vi "Recipe read write.vi"(7 "Use csv file":bool=TRUE, 8 "Write":bool, 9 "Info":string, 10 "Recipe path":path, 11 "Write input":T1={"SEM Scan Parameters"={"X size (um)"=20.0, "Y size (um)"=20.0, "X center (um)"=0.0, "Y center (um)"=0.0, "X size (V)"=6.190428211586902, "X size auto"=TRUE, "X stig"=[[0.0]], "Y stig"=[[0.0]], "X aln"=[[0.0]], "Y aln"=[[0.0]], "Scan rate (Hz)"=10000000, "Oversampling"=5, "Oversampling auto"=TRUE, "Frame line rampdown ratio"=0.1, "Pixel size (nm)"=10.0, "WD (mm)"=[[3.0]], "X tiles"=1, "Y tiles"=1, "Overlap (um)"=1.0, "Interlaced"=TRUE, "dX (um)"=[0.0], "dY (um)"=[0.0], "Frames"=1}, "Detector Information"={"Brightness A"=30.0, "Contrast A"=25.0, "Detector B name"="ESB", "Brightness B"=40.0, "Contrast B"=50.0, "Detector C name"="Detector C", "Detector D name"="Detector D"}, "SEM Options"={"GetInfo"=TRUE, "Set Det A para"=TRUE, "Set WD"=FALSE, "Set Mag"=TRUE, "Set stig"=FALSE, "Set aln"=FALSE, "Display"=TRUE, "Save"=TRUE, "8-bit"=TRUE, "Detector A"=TRUE, "Detector B"=FALSE, "Detector C"=FALSE, "Detector D"=FALSE, "Inverse A"=FALSE, "Inverse B"=FALSE, "Inverse C"=FALSE, "Inverse D"=FALSE, "Inverse PNG"=TRUE, "Freeze"=TRUE, "PNG only"=FALSE, "Upload"=TRUE, "Delete after upload"=FALSE}, "Focus Index Options"={"Keep aspect ratio"=FALSE, "Show Focus Index"=TRUE, "Focus Index primary grid center"=TRUE, "X Grids"=[[0]], "Y Grids"=[[0]], "Primary X index"=[[0]], "Primary Y index"=[[0]]}, "Image fit to"=0, "File Information"={"File path"=path "E:/Images", "Notes"="", "Save recipe"=FALSE, "Load recipe"=FALSE, "Sample ID"=""}, "Low mag SEM"={"Low mag scan"=TRUE, "Prior to main scan"=FALSE, "Low mag interval"=1, "Low mag scan FOV (micron)"=200.0, "Low mag scan rate (Hz)"=1000000, "Show HM box"=TRUE}, "Mid Mag SEM"={"Mid mag scan"=FALSE, "Prior to main scan"=FALSE, "Mid mag interval"=500, "X size (um)"=6144.0, "Y size (um)"=6144.0, "X center (um)"=0.0, "Y center (um)"=0.0, "Mid mag scan rate (Hz)"=1000000, "Pixel size (nm)"=10.0, "Show MM box"=TRUE}, "FIB-SEM Angle"=90.0, "Milling para"={"X resolution"=4096, "Z resolution"=125001, "X offset (um)"=0.0, "Z offset (um)"=0.0, "X center (um)"=0.0, "Z center (um)"=0.0, "X size (um)"=250.0, "Z size (um)"=250.0, "UL-Ang"=90.0, "UR-Ang"=90.0, "Line milling time (s)"=5.0, "Z-step (nm)"=2.0, "Lines auto pause"=1, "Auto pause"=FALSE, "Mill from Bottom"=FALSE, "FIB FOV (um)"=500.0, "Auto Profile"=FALSE, "Mill start from Last"=FALSE, "FIB PID on"=FALSE, "FIB PID reset"=TRUE, "FIB PID measured"=0, "FIB PID target"=0.0, "FIB PID target slope"=0.0, "FIB PID P"=0.001, "FIB PID I"=0.01, "FIB PID D"=0.0, "Emission (uA)"=1.36, "Suppressor (V)"=50.0, "Auto reheat"=FALSE}, "FI Detector"=0, "Auto Optimzation"=TRUE, "Images per Auto Optimization"=200, "AF Range (nm)"=1800.0, "AF Steps"=7, "AS Range (%)"=0.6, "AS Steps"=7, "AA Range (%)"=3.0, "AA Steps"=7, "X shift (nm/frame)"=0.0, "Y shift (nm/frame)"=0.0, "FIB Y zoom pixel (nm)"=20.0, "Mail server"="", "Email Alert Recipients"=[""], "Alert Settings"={"3D imaging paused alarm"=TRUE, "FIB emission limit warning"=TRUE, "Low limit"=1.4, "High limit"=2.0, "Specimen @ SEM alarm"=TRUE, "FIB CL current alarm"=TRUE, "Beam Dump 1 alarm"=TRUE, "Milling Z voltage alarm"=TRUE, "EHT off alarm"=TRUE, "Detector over scale warning"=TRUE, "Image clipping alarm"=TRUE, "Warning limit (um)"=1.4, "Stop limit (um)"=1.4, "Temperature alarm"=TRUE, "Pause 3D-ING"=FALSE, "Low limit (F)"=65.0, "High limit (F)"=80.0, "Temp limit auto"=TRUE, "Delta (F)"=0.2, "Gradient limit (F/min)"=0.03, "SW error warning"=TRUE, "Focus index warning"=TRUE, "Focus index low limit"=0.1, "Focus index stop limit"=0.0, "Run Auto Stig"=FALSE, "FI low limit auto"=TRUE, "FI stop limit auto"=TRUE}, "Reheat Parameters"={"Filament I (A)"=3.0, "Reheat time (s)"=45.0, "Emission (uA)"=2.2, "Calculate V/I slope"=TRUE, "Pre-calc delay (min)"=5.0, "Disable Reheat Retries"=FALSE, "Restore Voltages"=TRUE}, "Start FIB HV DataLog"=FALSE, "Interval (s)"=60} {"Milling para"."Suppressor (V)" step=0.1 format="%.1g"; "Milling para"."Emission (uA)" step=0.1 format="%.2g"; "Milling para"."FIB PID measured" items=["Spec.", "B.D. 1", "B.D. 2", "Mill", "Spec. +"]; "Milling para"."FIB PID target slope" min=-1 max=1 step=0.1; "Milling para"."UR-Ang" format="%.2f"; "Milling para"."UL-Ang" format="%.2f"; "Milling para"."Z offset (um)" step=0.02 format="%.3g"; "Milling para"."X offset (um)" step=1 format="%.3g"; "Milling para"."FIB FOV (um)" format="%.3g"; "Milling para"."Line milling time (s)" format="%.1f"; "Milling para"."Z center (um)" format="%#.3g"; "Milling para"."X center (um)" format="%#.3g"; "Alert Settings"."Stop limit (um)" format="%.2f"; "Alert Settings"."Warning limit (um)" format="%.2f"; "Alert Settings"."Focus index stop limit" format="%_3g"; "Alert Settings"."Focus index low limit" format="%_3g"; "Alert Settings"."High limit (F)" format="%.2g"; "Alert Settings"."Low limit (F)" format="%.2g"; "Alert Settings"."High limit" format="%.2f"; "Alert Settings"."Low limit" format="%.2f"; "SEM Scan Parameters"."dY (um)" format="%.1f"; "SEM Scan Parameters"."dX (um)" format="%.1f"; "SEM Scan Parameters"."Frames" min=1 step=1; "SEM Scan Parameters"."WD (mm)" format="%.1f"; "SEM Scan Parameters"."Y aln" format="%.1f"; "SEM Scan Parameters"."X aln" format="%.1f"; "SEM Scan Parameters"."Y stig" format="%.1f"; "SEM Scan Parameters"."X stig" format="%.1f"; "SEM Scan Parameters"."Overlap (um)" min=0; "SEM Scan Parameters"."Y tiles" min=1; "SEM Scan Parameters"."X tiles" min=1; "SEM Scan Parameters"."X size (um)" format="%.2f"; "SEM Scan Parameters"."Y size (um)" format="%.2f"; "SEM Scan Parameters"."Frame line rampdown ratio" min=0 max=1 step=0.05 format="%.2g"; "SEM Scan Parameters"."X center (um)" step=1.0 format="%.2f"; "SEM Scan Parameters"."Y center (um)" step=1.0 format="%.2f"; "SEM Scan Parameters"."X size (V)" format="%_4g"; "SEM Scan Parameters"."Scan rate (Hz)" max=4000000 step=100000 format="%.2e"; "Reheat Parameters"."Pre-calc delay (min)" format="%.2f"; "Reheat Parameters"."Emission (uA)" format="%.1f"; "Reheat Parameters"."Filament I (A)" format="%.2f"; "Reheat Parameters"."Reheat time (s)" format="%.1f"; "Image fit to" items=["Width", "Height"]; "Mid Mag SEM"."X center (um)" step=1.0 format="%.4f"; "Mid Mag SEM"."Y center (um)" step=1.0 format="%.4f"; "Mid Mag SEM"."Mid mag interval" min=1 step=1; "Mid Mag SEM"."Mid mag scan rate (Hz)" max=4000000 step=100000 format="%.2e"; "FIB Y zoom pixel (nm)" format="%.1g"; "X shift (nm/frame)" step=0.1; "Y shift (nm/frame)" step=0.1; "FI Detector" items=["A", "B", "C", "D"]; "Low mag SEM"."Low mag interval" min=1 step=1; "Low mag SEM"."Low mag scan rate (Hz)" max=4000000 step=100000 format="%.2e"; "Low mag SEM"."Low mag scan FOV (micron)" step=50.0; "FIB-SEM Angle" min=0.0 max=90.0}) -> (0 "error out":errorcluster, 1 "Recipe csv array":string[](array[string]), 2 "Recipe items":string[](array[string])=["SEM X resolution", "SEM Y resolution", "SEM X center", "SEM Y center", "SEM X size (V)", "SEM X size auto", "SEM X stig", "SEM Y stig", "SEM Scan rate (Hz)", "SEM WD (mm)", "SEM pixel size (nm)", "Frame line rampdown ratio", "SEM oversampling", "SEM oversampling auto", "Brightness A", "Contrast A", "Detector B name", "Brightness B", "Contrast B", "GetInfo", "Set Det A para", "Set WD", "Set Mag", "Set stig", "Display", "Save", "Detector A", "Detector B", "Detector C", "Detector D", "Inverse A", "Inverse B", "Inverse C", "Inverse D", "Inverse PNG", "Freeze", "PNG only", "File path", "Notes", "Low mag scan", "Prior to main scan", "per # of images", "Low mag scan FOV (um)", "Low mag scan rate (Hz)", "Show high mag box", "FIB-SEM angle", "Milling X resolution", "Milling Y resolution", "Milling X offset (um)", "Milling Y offset (um)", "Milling X center (um)", "Milling Y center (um)", "Milling X size (um)", "Milling Y size (um)", "Milling line milling time (s)", "Milling auto pause", "Milling lines auto pause", "Mill from bottom", "FIB FOV (um)", "SEM on during milling"], 3 "Read output":T1={"SEM Scan Parameters"={"X size (um)"=20.0, "Y size (um)"=20.0, "X center (um)"=0.0, "Y center (um)"=0.0, "X size (V)"=6.190428211586902, "X size auto"=TRUE, "X stig"=[[0.0]], "Y stig"=[[0.0]], "X aln"=[[0.0]], "Y aln"=[[0.0]], "Scan rate (Hz)"=10000000, "Oversampling"=5, "Oversampling auto"=TRUE, "Frame line rampdown ratio"=0.1, "Pixel size (nm)"=10.0, "WD (mm)"=[[3.0]], "X tiles"=1, "Y tiles"=1, "Overlap (um)"=1.0, "Interlaced"=TRUE, "dX (um)"=[0.0], "dY (um)"=[0.0], "Frames"=1}, "Detector Information"={"Brightness A"=30.0, "Contrast A"=25.0, "Detector B name"="ESB", "Brightness B"=40.0, "Contrast B"=50.0, "Detector C name"="Detector C", "Detector D name"="Detector D"}, "SEM Options"={"GetInfo"=TRUE, "Set Det A para"=TRUE, "Set WD"=FALSE, "Set Mag"=TRUE, "Set stig"=FALSE, "Set aln"=FALSE, "Display"=TRUE, "Save"=TRUE, "8-bit"=TRUE, "Detector A"=TRUE, "Detector B"=FALSE, "Detector C"=FALSE, "Detector D"=FALSE, "Inverse A"=FALSE, "Inverse B"=FALSE, "Inverse C"=FALSE, "Inverse D"=FALSE, "Inverse PNG"=TRUE, "Freeze"=TRUE, "PNG only"=FALSE, "Upload"=TRUE, "Delete after upload"=FALSE}, "Focus Index Options"={"Keep aspect ratio"=FALSE, "Show Focus Index"=TRUE, "Focus Index primary grid center"=TRUE, "X Grids"=[[0]], "Y Grids"=[[0]], "Primary X index"=[[0]], "Primary Y index"=[[0]]}, "Image fit to"=0, "File Information"={"File path"=path "E:/Images", "Notes"="", "Save recipe"=FALSE, "Load recipe"=FALSE, "Sample ID"=""}, "Low mag SEM"={"Low mag scan"=TRUE, "Prior to main scan"=FALSE, "Low mag interval"=1, "Low mag scan FOV (micron)"=200.0, "Low mag scan rate (Hz)"=1000000, "Show HM box"=TRUE}, "Mid Mag SEM"={"Mid mag scan"=FALSE, "Prior to main scan"=FALSE, "Mid mag interval"=500, "X size (um)"=6144.0, "Y size (um)"=6144.0, "X center (um)"=0.0, "Y center (um)"=0.0, "Mid mag scan rate (Hz)"=1000000, "Pixel size (nm)"=10.0, "Show MM box"=TRUE}, "FIB-SEM Angle"=90.0, "Milling para"={"X resolution"=4096, "Z resolution"=125001, "X offset (um)"=0.0, "Z offset (um)"=0.0, "X center (um)"=0.0, "Z center (um)"=0.0, "X size (um)"=250.0, "Z size (um)"=250.0, "UL-Ang"=90.0, "UR-Ang"=90.0, "Line milling time (s)"=5.0, "Z-step (nm)"=2.0, "Lines auto pause"=1, "Auto pause"=FALSE, "Mill from Bottom"=FALSE, "FIB FOV (um)"=500.0, "Auto Profile"=FALSE, "Mill start from Last"=FALSE, "FIB PID on"=FALSE, "FIB PID reset"=TRUE, "FIB PID measured"=0, "FIB PID target"=0.0, "FIB PID target slope"=0.0, "FIB PID P"=0.001, "FIB PID I"=0.01, "FIB PID D"=0.0, "Emission (uA)"=1.36, "Suppressor (V)"=50.0, "Auto reheat"=FALSE}, "FI Detector"=0, "Auto Optimzation"=TRUE, "Images per Auto Optimization"=200, "AF Range (nm)"=1800.0, "AF Steps"=7, "AS Range (%)"=0.6, "AS Steps"=7, "AA Range (%)"=3.0, "AA Steps"=7, "X shift (nm/frame)"=0.0, "Y shift (nm/frame)"=0.0, "FIB Y zoom pixel (nm)"=20.0, "Mail server"="", "Email Alert Recipients"=[""], "Alert Settings"={"3D imaging paused alarm"=TRUE, "FIB emission limit warning"=TRUE, "Low limit"=1.4, "High limit"=2.0, "Specimen @ SEM alarm"=TRUE, "FIB CL current alarm"=TRUE, "Beam Dump 1 alarm"=TRUE, "Milling Z voltage alarm"=TRUE, "EHT off alarm"=TRUE, "Detector over scale warning"=TRUE, "Image clipping alarm"=TRUE, "Warning limit (um)"=1.4, "Stop limit (um)"=1.4, "Temperature alarm"=TRUE, "Pause 3D-ING"=FALSE, "Low limit (F)"=65.0, "High limit (F)"=80.0, "Temp limit auto"=TRUE, "Delta (F)"=0.2, "Gradient limit (F/min)"=0.03, "SW error warning"=TRUE, "Focus index warning"=TRUE, "Focus index low limit"=0.1, "Focus index stop limit"=0.0, "Run Auto Stig"=FALSE, "FI low limit auto"=TRUE, "FI stop limit auto"=TRUE}, "Reheat Parameters"={"Filament I (A)"=3.0, "Reheat time (s)"=45.0, "Emission (uA)"=2.2, "Calculate V/I slope"=TRUE, "Pre-calc delay (min)"=5.0, "Disable Reheat Retries"=FALSE, "Restore Voltages"=TRUE}, "Start FIB HV DataLog"=FALSE, "Interval (s)"=60} {"Milling para"."Suppressor (V)" step=0.1 format="%.1g"; "Milling para"."Emission (uA)" step=0.1 format="%.2g"; "Milling para"."FIB PID measured" items=["Spec.", "B.D. 1", "B.D. 2", "Mill", "Spec. +"]; "Milling para"."FIB PID target slope" min=-1 max=1 step=0.1; "Milling para"."UR-Ang" format="%.2f"; "Milling para"."UL-Ang" format="%.2f"; "Milling para"."Z offset (um)" step=0.02 format="%.3g"; "Milling para"."X offset (um)" step=1 format="%.3g"; "Milling para"."FIB FOV (um)" format="%.3g"; "Milling para"."Line milling time (s)" format="%.1f"; "Milling para"."Z center (um)" format="%#.3g"; "Milling para"."X center (um)" format="%#.3g"; "Alert Settings"."Stop limit (um)" format="%.2f"; "Alert Settings"."Warning limit (um)" format="%.2f"; "Alert Settings"."Focus index stop limit" format="%_3g"; "Alert Settings"."Focus index low limit" format="%_3g"; "Alert Settings"."High limit (F)" format="%.2g"; "Alert Settings"."Low limit (F)" format="%.2g"; "Alert Settings"."High limit" format="%.2f"; "Alert Settings"."Low limit" format="%.2f"; "SEM Scan Parameters"."dY (um)" format="%.1f"; "SEM Scan Parameters"."dX (um)" format="%.1f"; "SEM Scan Parameters"."Frames" min=1 step=1; "SEM Scan Parameters"."WD (mm)" format="%.1f"; "SEM Scan Parameters"."Y aln" format="%.1f"; "SEM Scan Parameters"."X aln" format="%.1f"; "SEM Scan Parameters"."Y stig" format="%.1f"; "SEM Scan Parameters"."X stig" format="%.1f"; "SEM Scan Parameters"."Overlap (um)" min=0; "SEM Scan Parameters"."Y tiles" min=1; "SEM Scan Parameters"."X tiles" min=1; "SEM Scan Parameters"."X size (um)" format="%.2f"; "SEM Scan Parameters"."Y size (um)" format="%.2f"; "SEM Scan Parameters"."Frame line rampdown ratio" min=0 max=1 step=0.05 format="%.2g"; "SEM Scan Parameters"."X center (um)" step=1.0 format="%.2f"; "SEM Scan Parameters"."Y center (um)" step=1.0 format="%.2f"; "SEM Scan Parameters"."X size (V)" format="%_4g"; "SEM Scan Parameters"."Scan rate (Hz)" max=4000000 step=100000 format="%.2e"; "Reheat Parameters"."Pre-calc delay (min)" format="%.2f"; "Reheat Parameters"."Emission (uA)" format="%.1f"; "Reheat Parameters"."Filament I (A)" format="%.2f"; "Reheat Parameters"."Reheat time (s)" format="%.1f"; "Image fit to" items=["Width", "Height"]; "Mid Mag SEM"."X center (um)" step=1.0 format="%.4f"; "Mid Mag SEM"."Y center (um)" step=1.0 format="%.4f"; "Mid Mag SEM"."Mid mag interval" min=1 step=1; "Mid Mag SEM"."Mid mag scan rate (Hz)" max=4000000 step=100000 format="%.2e"; "FIB Y zoom pixel (nm)" format="%.1g"; "X shift (nm/frame)" step=0.1; "Y shift (nm/frame)" step=0.1; "FI Detector" items=["A", "B", "C", "D"]; "Low mag SEM"."Low mag interval" min=1 step=1; "Low mag SEM"."Low mag scan rate (Hz)" max=4000000 step=100000 format="%.2e"; "Low mag SEM"."Low mag scan FOV (micron)" step=50.0; "FIB-SEM Angle" min=0.0 max=90.0})   [LabVIEW 2018]
uses:
  <vilib>/Utility/file.llb/Read From Spreadsheet File (string).vi
  <vilib>/regexp/Match Regular Expression.xnode
panel:
  out "Read output 1":T2={"SEM Scan Parameters"={"X size (um)"=20.0, "Y size (um)"=20.0, "X center (um)"=0.0, "Y center (um)"=0.0, "X size (V)"=6.190428211586902, "X size auto"=TRUE, "X stig"=[[0.0]], "Y stig"=[[0.0]], "X aln"=[[0.0]], "Y aln"=[[0.0]], "Scan rate (Hz)"=10000000, "Oversampling"=5, "Oversampling auto"=TRUE, "Frame line rampdown ratio"=0.1, "Pixel size (nm)"=10.0, "WD (mm)"=[[3.0]], "X tiles"=1, "Y tiles"=1, "Overlap (um)"=1.0, "Interlaced"=TRUE, "dX (um)"=[0.0], "dY (um)"=[0.0], "Frames"=1}, "Detector Information"={"Brightness A"=30.0, "Contrast A"=25.0, "Detector B name"="ESB", "Brightness B"=40.0, "Contrast B"=50.0, "Detector C name"="Detector C", "Detector D name"="Detector D"}, "SEM Options"={"GetInfo"=TRUE, "Set Det A para"=TRUE, "Set WD"=FALSE, "Set Mag"=TRUE, "Set stig"=FALSE, "Set aln"=FALSE, "Display"=TRUE, "Save"=TRUE, "8-bit"=TRUE, "Detector A"=TRUE, "Detector B"=FALSE, "Detector C"=FALSE, "Detector D"=FALSE, "Inverse A"=FALSE, "Inverse B"=FALSE, "Inverse C"=FALSE, "Inverse D"=FALSE, "Inverse PNG"=TRUE, "Freeze"=TRUE, "PNG only"=FALSE, "Upload"=TRUE, "Delete after upload"=FALSE}, "Focus Index Options"={"Keep aspect ratio"=FALSE, "Show Focus Index"=TRUE, "Focus Index primary grid center"=TRUE, "X Grids"=[[0]], "Y Grids"=[[0]], "Primary X index"=[[0]], "Primary Y index"=[[0]]}, "Image fit to"=0, "File Information"={"File path"=path "E:/Images", "Notes"="", "Save recipe"=FALSE, "Load recipe"=FALSE, "Sample ID"=""}, "Low mag SEM"={"Low mag scan"=TRUE, "Prior to main scan"=FALSE, "Low mag interval"=1, "Low mag scan FOV (micron)"=200.0, "Low mag scan rate (Hz)"=1000000, "Show HM box"=TRUE}, "Mid Mag SEM"={"Mid mag scan"=FALSE, "Prior to main scan"=FALSE, "Mid mag interval"=500, "X size (um)"=6144.0, "Y size (um)"=6144.0, "X center (um)"=0.0, "Y center (um)"=0.0, "Mid mag scan rate (Hz)"=1000000, "Pixel size (nm)"=10.0, "Show MM box"=TRUE}, "FIB-SEM Angle"=90.0, "Milling para"={"X resolution"=4096, "Y resolution"=100001, "X offset (um)"=0.0, "Y offset (um)"=0.0, "X center (um)"=0.0, "Y center (um)"=0.0, "X size (um)"=250.0, "Y size (um)"=250.0, "UL-Ang"=90.0, "UR-Ang"=90.0, "Line milling time (s)"=5.0, "Auto pause"=FALSE, "Lines auto pause"=1, "Mill from Bottom"=FALSE, "FIB FOV (um)"=500.0, "Auto Profile"=FALSE, "Mill start from Last"=FALSE, "FIB PID on"=FALSE, "FIB PID reset"=FALSE, "FIB PID measured"=0, "FIB PID target"=0.0, "FIB PID target slope"=0.0, "FIB PID P"=0.0, "FIB PID I"=0.0, "FIB PID D"=0.0}, "FI Detector"=0, "Auto Optimzation"=TRUE, "Images per Auto Optimization"=200, "AF Range (nm)"=1800.0, "AF Steps"=7, "AS Range (%)"=0.6, "AS Steps"=7, "AA Range (%)"=3.0, "AA Steps"=7, "X shift (nm/frame)"=0.0, "Y shift (nm/frame)"=0.0, "FIB Settings"={"Z-step (nm)"=2.5, "Enable alarm"=TRUE, "Label"="Emission Alarm (nA)", "Emission min"=1.2, "Emission max"=2.2, "Auto reheat"=FALSE}, "FIB Y zoom pixel (nm)"=20.0, "Mail server"="", "Email Alert Recipients"=[""], "Alert Settings"={"3D imaging paused alarm"=TRUE, "FIB emission limit warning"=TRUE, "Low limit"=1.4, "High limit"=2.0, "Specimen @ SEM alarm"=TRUE, "FIB CL current alarm"=TRUE, "Beam Dump 1 alarm"=TRUE, "Milling Y voltage alarm"=TRUE, "EHT off alarm"=TRUE, "Detector over scale warning"=TRUE, "Image clipping alarm"=TRUE, "Warning limit (um)"=1.4, "Stop limit (um)"=1.4, "Temperature alarm"=TRUE, "Pause 3D-ING"=FALSE, "Low limit (F)"=65.0, "High limit (F)"=80.0, "Temp limit auto"=TRUE, "Delta (F)"=0.2, "Gradient limit (F/min)"=0.03, "SW error warning"=TRUE, "Focus index warning"=TRUE, "Focus index low limit"=0.1, "Focus index stop limit"=0.0, "Run Auto Stig"=FALSE, "FI low limit auto"=TRUE, "FI stop limit auto"=TRUE}, "Reheat Parameters"={"Filament I (A)"=3.0, "Reheat time (s)"=45.0, "Emission (uA)"=2.2, "Calculate V/I slope"=TRUE, "Pre-calc delay (min)"=5.0, "Disable Reheat Retries"=FALSE, "Restore Voltages"=TRUE}, "Start FIB HV DataLog"=FALSE, "Interval (s)"=60} {"Alert Settings"."Stop limit (um)" format="%.2f"; "Alert Settings"."Warning limit (um)" format="%.2f"; "Alert Settings"."Focus index stop limit" format="%_3g"; "Alert Settings"."Focus index low limit" format="%_3g"; "Alert Settings"."High limit (F)" format="%.2g"; "Alert Settings"."Low limit (F)" format="%.2g"; "Alert Settings"."High limit" format="%.2f"; "Alert Settings"."Low limit" format="%.2f"; "SEM Scan Parameters"."dY (um)" format="%.1f"; "SEM Scan Parameters"."dX (um)" format="%.1f"; "SEM Scan Parameters"."Frames" min=1 step=1; "SEM Scan Parameters"."WD (mm)" format="%.1f"; "SEM Scan Parameters"."Y aln" format="%.1f"; "SEM Scan Parameters"."X aln" format="%.1f"; "SEM Scan Parameters"."Y stig" format="%.1f"; "SEM Scan Parameters"."X stig" format="%.1f"; "SEM Scan Parameters"."Overlap (um)" min=0; "SEM Scan Parameters"."Y tiles" min=1; "SEM Scan Parameters"."X tiles" min=1; "SEM Scan Parameters"."X size (um)" format="%.2f"; "SEM Scan Parameters"."Y size (um)" format="%.2f"; "SEM Scan Parameters"."Frame line rampdown ratio" min=0 max=1 step=0.05 format="%.2g"; "SEM Scan Parameters"."X center (um)" step=1.0 format="%.2f"; "SEM Scan Parameters"."Y center (um)" step=1.0 format="%.2f"; "SEM Scan Parameters"."X size (V)" format="%_4g"; "SEM Scan Parameters"."Scan rate (Hz)" max=4000000 step=100000 format="%.2e"; "Reheat Parameters"."Pre-calc delay (min)" format="%.2f"; "Reheat Parameters"."Emission (uA)" format="%.1f"; "Reheat Parameters"."Filament I (A)" format="%.2f"; "Reheat Parameters"."Reheat time (s)" format="%.1f"; "Image fit to" items=["Width", "Height"]; "Mid Mag SEM"."X center (um)" step=1.0 format="%.4f"; "Mid Mag SEM"."Y center (um)" step=1.0 format="%.4f"; "Mid Mag SEM"."Mid mag interval" min=1 step=1; "Mid Mag SEM"."Mid mag scan rate (Hz)" max=4000000 step=100000 format="%.2e"; "Milling para"."FIB PID measured" items=["Spec.", "B.D.1", "B.D.2", "Mill"]; "Milling para"."UR-Ang" format="%.2f"; "Milling para"."UL-Ang" format="%.2f"; "Milling para"."Y offset (um)" step=0.02 format="%.3g"; "Milling para"."X offset (um)" step=1 format="%.3g"; "Milling para"."FIB FOV (um)" format="%.3g"; "Milling para"."Line milling time (s)" format="%.1f"; "Milling para"."Y center (um)" format="%#.3g"; "Milling para"."X center (um)" format="%#.3g"; "FIB Y zoom pixel (nm)" format="%.1g"; "FIB Settings"."Emission min" format="%.1g"; "FIB Settings"."Emission max" format="%.1g"; "X shift (nm/frame)" step=0.1; "Y shift (nm/frame)" step=0.1; "FI Detector" items=["A", "B", "C", "D"]; "Low mag SEM"."Low mag interval" min=1 step=1; "Low mag SEM"."Low mag scan rate (Hz)" max=4000000 step=100000 format="%.2e"; "Low mag SEM"."Low mag scan FOV (micron)" step=50.0; "FIB-SEM Angle" min=0.0 max=90.0}
  out "Read output 3":T3={"SEM Scan Parameters"={"X size (um)"=20.0, "Y size (um)"=20.0, "X center (um)"=0.0, "Y center (um)"=0.0, "X size (V)"=6.190428211586902, "X size auto"=TRUE, "X stig"=[[0.0]], "Y stig"=[[0.0]], "X aln"=[[0.0]], "Y aln"=[[0.0]], "Scan rate (Hz)"=10000000, "Oversampling"=5, "Oversampling auto"=TRUE, "Frame line rampdown ratio"=0.1, "Pixel size (nm)"=10.0, "WD (mm)"=[[3.0]], "X tiles"=1, "Y tiles"=1, "Overlap (um)"=1.0, "Interlaced"=TRUE, "dX (um)"=[0.0], "dY (um)"=[0.0], "Frames"=1}, "Detector Information"={"Brightness A"=30.0, "Contrast A"=25.0, "Detector B name"="ESB", "Brightness B"=40.0, "Contrast B"=50.0, "Detector C name"="Detector C", "Detector D name"="Detector D"}, "SEM Options"={"GetInfo"=TRUE, "Set Det A para"=TRUE, "Set WD"=FALSE, "Set Mag"=TRUE, "Set stig"=FALSE, "Set aln"=FALSE, "Display"=TRUE, "Save"=TRUE, "8-bit"=TRUE, "Detector A"=TRUE, "Detector B"=FALSE, "Detector C"=FALSE, "Detector D"=FALSE, "Inverse A"=FALSE, "Inverse B"=FALSE, "Inverse C"=FALSE, "Inverse D"=FALSE, "Inverse PNG"=TRUE, "Freeze"=TRUE, "PNG only"=FALSE, "Upload"=TRUE, "Delete after upload"=FALSE}, "Keep aspect ratio"=TRUE, "Show Focus Index"=TRUE, "Focus Index primary grid center"=TRUE, "Focus Index grid X"=1, "Focus Index grid Y"=1, "Focus Index primary X grid"=0, "Focus Index primary Y grid"=0, "Image fit to"=0, "File Information"={"File path"=path "E:/Images", "Notes"="", "Save recipe"=FALSE, "Load recipe"=FALSE, "Sample ID"=""}, "Low mag SEM"={"Low mag scan"=TRUE, "Prior to main scan"=FALSE, "Low mag interval"=1, "Low mag scan FOV (micron)"=200.0, "Low mag scan rate (Hz)"=1000000, "Show HM box"=TRUE}, "Mid Mag SEM"={"Mid mag scan"=FALSE, "Prior to main scan"=FALSE, "Mid mag interval"=500, "X size (um)"=6144.0, "Y size (um)"=6144.0, "X center (um)"=0.0, "Y center (um)"=0.0, "Mid mag scan rate (Hz)"=1000000, "Pixel size (nm)"=10.0, "Show MM box"=TRUE}, "FIB-SEM Angle"=90.0, "Milling para"={"X resolution"=4096, "Y resolution"=100001, "X offset (um)"=0.0, "Y offset (um)"=0.0, "X center (um)"=0.0, "Y center (um)"=0.0, "X size (um)"=250.0, "Y size (um)"=250.0, "UL-Ang"=90.0, "UR-Ang"=90.0, "Line milling time (s)"=5.0, "Auto pause"=FALSE, "Lines auto pause"=1, "Mill from Bottom"=FALSE, "FIB FOV (um)"=500.0, "Auto Profile"=FALSE, "Mill start from Last"=FALSE, "FIB PID on"=FALSE, "FIB PID reset"=FALSE, "FIB PID measured"=0, "FIB PID target"=0.0, "FIB PID target slope"=0.0, "FIB PID P"=0.0, "FIB PID I"=0.0, "FIB PID D"=0.0}, "FI Detector"=0, "Auto Optimzation"=TRUE, "Images per Auto Optimization"=200, "AF Range (nm)"=1800.0, "AF Steps"=7, "AS Range (%)"=0.6, "AS Steps"=7, "AA Range (%)"=3.0, "AA Steps"=7, "X shift (nm/frame)"=0.0, "Y shift (nm/frame)"=0.0, "FIB Settings"={"Z-step (nm)"=2.5, "Enable alarm"=TRUE, "Label"="Emission Alarm (nA)", "Emission min"=1.2, "Emission max"=2.2, "Auto reheat"=FALSE}, "FIB Y zoom pixel (nm)"=20.0, "Mail server"="", "Email Alert Recipients"=[""], "Alert Settings"={"3D imaging paused alarm"=TRUE, "FIB emission limit warning"=TRUE, "Low limit"=17.0, "High limit"=23.0, "Specimen current alarm "=TRUE, "Beam dump alarm"=TRUE, "EHT off alarm"=TRUE, "Temperature alarm"=TRUE, "Pause 3D-ING"=FALSE, "Low limit (F)"=70.0, "High limit (F)"=80.0, "Temp limit auto"=TRUE, "Delta (F)"=0.2, "Gradient limit (F/min)"=0.03, "SW error warning"=TRUE, "Focus index warning"=TRUE, "Focus index low limit"=0.1, "Focus index stop limit"=0.0, "Run Auto Stig"=FALSE, "FI low limit auto"=TRUE, "FI stop limit auto"=TRUE}, "Reheat Parameters"={"Filament I (A)"=3.0, "Reheat time (s)"=45.0, "Emission (uA)"=2.2, "Calculate V/I slope"=TRUE, "Pre-calc delay (min)"=5.0, "Disable Reheat Retries"=FALSE, "Restore Voltages"=TRUE}, "Start FIB HV DataLog"=FALSE, "Interval (s)"=60} {"SEM Scan Parameters"."dY (um)" format="%.1f"; "SEM Scan Parameters"."dX (um)" format="%.1f"; "SEM Scan Parameters"."Frames" min=1 step=1; "SEM Scan Parameters"."WD (mm)" format="%.1f"; "SEM Scan Parameters"."Y aln" format="%.1f"; "SEM Scan Parameters"."X aln" format="%.1f"; "SEM Scan Parameters"."Y stig" format="%.1f"; "SEM Scan Parameters"."X stig" format="%.1f"; "SEM Scan Parameters"."Overlap (um)" min=0; "SEM Scan Parameters"."Y tiles" min=1; "SEM Scan Parameters"."X tiles" min=1; "SEM Scan Parameters"."X size (um)" format="%.2f"; "SEM Scan Parameters"."Y size (um)" format="%.2f"; "SEM Scan Parameters"."Frame line rampdown ratio" min=0 max=1 step=0.05 format="%.2g"; "SEM Scan Parameters"."X center (um)" step=1.0 format="%.2f"; "SEM Scan Parameters"."Y center (um)" step=1.0 format="%.2f"; "SEM Scan Parameters"."X size (V)" format="%_4g"; "SEM Scan Parameters"."Scan rate (Hz)" max=4000000 step=100000 format="%.2e"; "Reheat Parameters"."Pre-calc delay (min)" format="%.2f"; "Reheat Parameters"."Emission (uA)" format="%.1f"; "Reheat Parameters"."Filament I (A)" format="%.2f"; "Reheat Parameters"."Reheat time (s)" format="%.1f"; "Image fit to" items=["Width", "Height"]; "Mid Mag SEM"."X center (um)" step=1.0 format="%.4f"; "Mid Mag SEM"."Y center (um)" step=1.0 format="%.4f"; "Mid Mag SEM"."Mid mag interval" min=1 step=1; "Mid Mag SEM"."Mid mag scan rate (Hz)" max=4000000 step=100000 format="%.2e"; "Alert Settings"."Focus index stop limit" format="%_3g"; "Milling para"."FIB PID measured" items=["Spec.", "B.D.1", "B.D.2", "Mill"]; "Milling para"."UR-Ang" format="%.2f"; "Milling para"."UL-Ang" format="%.2f"; "Milling para"."Y offset (um)" step=0.02 format="%.3g"; "Milling para"."X offset (um)" step=1 format="%.3g"; "Milling para"."FIB FOV (um)" format="%.3g"; "Milling para"."Line milling time (s)" format="%.1f"; "Milling para"."Y center (um)" format="%#.3g"; "Milling para"."X center (um)" format="%#.3g"; "Focus Index grid X" min=1; "Focus Index grid Y" min=1; "FIB Y zoom pixel (nm)" format="%.1g"; "FIB Settings"."Emission min" format="%.1g"; "FIB Settings"."Emission max" format="%.1g"; "X shift (nm/frame)" step=0.1; "Y shift (nm/frame)" step=0.1; "FI Detector" items=["A", "B", "C", "D"]; "Low mag SEM"."Low mag interval" min=1 step=1; "Low mag SEM"."Low mag scan rate (Hz)" max=4000000 step=100000 format="%.2e"; "Low mag SEM"."Low mag scan FOV (micron)" step=50.0; "FIB-SEM Angle" min=0.0 max=90.0}
  out "Read output 4":T4={"SEM Scan Parameters"={"X size (um)"=20.0, "Y size (um)"=20.0, "X center (um)"=0.0, "Y center (um)"=0.0, "X size (V)"=6.190428211586902, "X size auto"=TRUE, "X stig"=[[0.0]], "Y stig"=[[0.0]], "X aln"=[[0.0]], "Y aln"=[[0.0]], "Scan rate (Hz)"=10000000, "Oversampling"=5, "Oversampling auto"=TRUE, "Frame line rampdown ratio"=0.1, "Pixel size (nm)"=10.0, "WD (mm)"=[[3.0]], "X tiles"=1, "Y tiles"=1, "Overlap (um)"=1.0, "Interlaced"=TRUE, "dX (um)"=0.0, "dY (um)"=0.0, "Frames"=1}, "Detector Information"={"Brightness A"=30.0, "Contrast A"=25.0, "Detector B name"="ESB", "Brightness B"=40.0, "Contrast B"=50.0, "Detector C name"="Detector C", "Detector D name"="Detector D"}, "SEM Options"={"GetInfo"=TRUE, "Set Det A para"=TRUE, "Set WD"=FALSE, "Set Mag"=TRUE, "Set stig"=FALSE, "Set aln"=FALSE, "Display"=TRUE, "Save"=TRUE, "8-bit"=TRUE, "Detector A"=TRUE, "Detector B"=FALSE, "Detector C"=FALSE, "Detector D"=FALSE, "Inverse A"=FALSE, "Inverse B"=FALSE, "Inverse C"=FALSE, "Inverse D"=FALSE, "Inverse PNG"=TRUE, "Freeze"=TRUE, "PNG only"=FALSE, "Upload"=TRUE, "Delete after upload"=FALSE}, "Keep aspect ratio"=TRUE, "Show Focus Index"=TRUE, "Focus Index primary grid center"=TRUE, "Focus Index grid X"=1, "Focus Index grid Y"=1, "Focus Index primary X grid"=0, "Focus Index primary Y grid"=0, "Image fit to"=0, "File Information"={"File path"=path "E:/Images", "Notes"="", "Save recipe"=FALSE, "Load recipe"=FALSE, "Sample ID"=""}, "Low mag SEM"={"Low mag scan"=TRUE, "Prior to main scan"=FALSE, "Low mag interval"=1, "Low mag scan FOV (micron)"=200.0, "Low mag scan rate (Hz)"=1000000, "Show HM box"=TRUE}, "Mid Mag SEM"={"Mid mag scan"=FALSE, "Prior to main scan"=FALSE, "Mid mag interval"=500, "X size (um)"=6144.0, "Y size (um)"=6144.0, "X center (um)"=0.0, "Y center (um)"=0.0, "Mid mag scan rate (Hz)"=1000000, "Pixel size (nm)"=10.0, "Show MM box"=TRUE}, "FIB-SEM Angle"=90.0, "Milling para"={"X resolution"=4096, "Y resolution"=100001, "X offset (um)"=0.0, "Y offset (um)"=0.0, "X center (um)"=0.0, "Y center (um)"=0.0, "X size (um)"=250.0, "Y size (um)"=250.0, "UL-Ang"=90.0, "UR-Ang"=90.0, "Line milling time (s)"=5.0, "Auto pause"=FALSE, "Lines auto pause"=1, "Mill from Bottom"=FALSE, "FIB FOV (um)"=500.0, "SEM on"=FALSE, "Mill start from Last"=FALSE, "FIB PID on"=FALSE, "FIB PID reset"=FALSE, "FIB PID measured"=0, "FIB PID target"=0.0, "FIB PID target slope"=0.0, "FIB PID P"=0.0, "FIB PID I"=0.0, "FIB PID D"=0.0}, "FI Detector"=0, "Auto Optimzation"=TRUE, "Images per Auto Optimization"=200, "AF Range (nm)"=1800.0, "AF Steps"=7, "AS Range (%)"=0.6, "AS Steps"=7, "AA Range (%)"=3.0, "AA Steps"=7, "X shift (nm/frame)"=0.0, "Y shift (nm/frame)"=0.0, "FIB Settings"={"Z-step (nm)"=2.5, "Enable alarm"=TRUE, "Label"="Emission Alarm (nA)", "Emission min"=1.2, "Emission max"=2.2, "Auto reheat"=FALSE}, "FIB Y zoom pixel (nm)"=20.0, "Mail server"="", "Email Alert Recipients"=[""], "Alert Settings"={"3D imaging paused alarm"=TRUE, "FIB emission limit warning"=TRUE, "Low limit"=17.0, "High limit"=23.0, "Specimen current alarm "=TRUE, "Beam dump alarm"=TRUE, "EHT off alarm"=TRUE, "Temperature alarm"=TRUE, "Pause 3D-ING"=FALSE, "Low limit (F)"=70.0, "High limit (F)"=80.0, "Temp limit auto"=TRUE, "Delta (F)"=0.2, "Gradient limit (F/min)"=0.03, "SW error warning"=TRUE, "Focus index warning"=TRUE, "Focus index low limit"=0.1, "Focus index stop limit"=0.0, "Run Auto Stig"=FALSE, "FI low limit auto"=TRUE, "FI stop limit auto"=TRUE}, "Reheat Parameters"={"Filament I (A)"=3.0, "Reheat time (s)"=45.0, "Emission (uA)"=2.2, "Calculate V/I slope"=TRUE, "Pre-calc delay (min)"=5.0, "Disable Reheat Retries"=FALSE, "Restore Voltages"=TRUE}, "Start FIB HV DataLog"=FALSE, "Interval (s)"=60} {"SEM Scan Parameters"."Frames" min=1 step=1; "SEM Scan Parameters"."dX (um)" step=1 format="%.2f"; "SEM Scan Parameters"."dY (um)" step=1 format="%.2f"; "SEM Scan Parameters"."WD (mm)" format="%.1f"; "SEM Scan Parameters"."Y aln" format="%.1f"; "SEM Scan Parameters"."X aln" format="%.1f"; "SEM Scan Parameters"."Y stig" format="%.1f"; "SEM Scan Parameters"."X stig" format="%.1f"; "SEM Scan Parameters"."Overlap (um)" min=0; "SEM Scan Parameters"."Y tiles" min=1; "SEM Scan Parameters"."X tiles" min=1; "SEM Scan Parameters"."X size (um)" format="%.2f"; "SEM Scan Parameters"."Y size (um)" format="%.2f"; "SEM Scan Parameters"."Frame line rampdown ratio" min=0 max=1 step=0.05 format="%.2g"; "SEM Scan Parameters"."X center (um)" step=1.0 format="%.2f"; "SEM Scan Parameters"."Y center (um)" step=1.0 format="%.2f"; "SEM Scan Parameters"."X size (V)" format="%_4g"; "SEM Scan Parameters"."Scan rate (Hz)" max=4000000 step=100000 format="%.2e"; "Reheat Parameters"."Pre-calc delay (min)" format="%.2f"; "Reheat Parameters"."Emission (uA)" format="%.1f"; "Reheat Parameters"."Filament I (A)" format="%.2f"; "Reheat Parameters"."Reheat time (s)" format="%.1f"; "Image fit to" items=["Width", "Height"]; "Mid Mag SEM"."X center (um)" step=1.0 format="%.4f"; "Mid Mag SEM"."Y center (um)" step=1.0 format="%.4f"; "Mid Mag SEM"."Mid mag interval" min=1 step=1; "Mid Mag SEM"."Mid mag scan rate (Hz)" max=4000000 step=100000 format="%.2e"; "Alert Settings"."Focus index stop limit" format="%_3g"; "Milling para"."FIB PID measured" items=["Spec.", "B.D.1", "B.D.2", "Mill"]; "Milling para"."UR-Ang" format="%.2f"; "Milling para"."UL-Ang" format="%.2f"; "Milling para"."Y offset (um)" step=0.02 format="%.3g"; "Milling para"."X offset (um)" step=1 format="%.3g"; "Milling para"."FIB FOV (um)" format="%.3g"; "Milling para"."Line milling time (s)" format="%.1f"; "Milling para"."Y center (um)" format="%#.3g"; "Milling para"."X center (um)" format="%#.3g"; "Focus Index grid X" min=1; "Focus Index grid Y" min=1; "FIB Y zoom pixel (nm)" format="%.1g"; "FIB Settings"."Emission min" format="%.1g"; "FIB Settings"."Emission max" format="%.1g"; "X shift (nm/frame)" step=0.1; "Y shift (nm/frame)" step=0.1; "FI Detector" items=["A", "B", "C", "D"]; "Low mag SEM"."Low mag interval" min=1 step=1; "Low mag SEM"."Low mag scan rate (Hz)" max=4000000 step=100000 format="%.2e"; "Low mag SEM"."Low mag scan FOV (micron)" step=50.0; "FIB-SEM Angle" min=0.0 max=90.0}
  out "Read output 2":T5={"SEM Scan Parameters"={"X size (um)"=20.0, "Y size (um)"=20.0, "X center (um)"=0.0, "Y center (um)"=0.0, "X size (V)"=6.190428211586902, "X size auto"=TRUE, "X stig"=[[0.0]], "Y stig"=[[0.0]], "X aln"=[[0.0]], "Y aln"=[[0.0]], "Scan rate (Hz)"=10000000, "Oversampling"=5, "Oversampling auto"=TRUE, "Frame line rampdown ratio"=0.1, "Pixel size (nm)"=10.0, "WD (mm)"=[[3.0]], "X tiles"=1, "Y tiles"=1, "Overlap (um)"=1.0, "Interlaced"=TRUE, "dX (um)"=[0.0], "dY (um)"=[0.0], "Frames"=1}, "Detector Information"={"Brightness A"=30.0, "Contrast A"=25.0, "Detector B name"="ESB", "Brightness B"=40.0, "Contrast B"=50.0, "Detector C name"="Detector C", "Detector D name"="Detector D"}, "SEM Options"={"GetInfo"=TRUE, "Set Det A para"=TRUE, "Set WD"=FALSE, "Set Mag"=TRUE, "Set stig"=FALSE, "Set aln"=FALSE, "Display"=TRUE, "Save"=TRUE, "8-bit"=TRUE, "Detector A"=TRUE, "Detector B"=FALSE, "Detector C"=FALSE, "Detector D"=FALSE, "Inverse A"=FALSE, "Inverse B"=FALSE, "Inverse C"=FALSE, "Inverse D"=FALSE, "Inverse PNG"=TRUE, "Freeze"=TRUE, "PNG only"=FALSE, "Upload"=TRUE, "Delete after upload"=FALSE}, "Keep aspect ratio"=TRUE, "Show Focus Index"=TRUE, "Focus Index primary grid center"=TRUE, "Focus Index grid X"=1, "Focus Index grid Y"=1, "Focus Index primary X grid"=0, "Focus Index primary Y grid"=0, "Image fit to"=0, "File Information"={"File path"=path "E:/Images", "Notes"="", "Save recipe"=FALSE, "Load recipe"=FALSE, "Sample ID"=""}, "Low mag SEM"={"Low mag scan"=TRUE, "Prior to main scan"=FALSE, "Low mag interval"=1, "Low mag scan FOV (micron)"=200.0, "Low mag scan rate (Hz)"=1000000, "Show HM box"=TRUE}, "Mid Mag SEM"={"Mid mag scan"=FALSE, "Prior to main scan"=FALSE, "Mid mag interval"=500, "X size (um)"=6144.0, "Y size (um)"=6144.0, "X center (um)"=0.0, "Y center (um)"=0.0, "Mid mag scan rate (Hz)"=1000000, "Pixel size (nm)"=10.0, "Show MM box"=TRUE}, "FIB-SEM Angle"=90.0, "Milling para"={"X resolution"=4096, "Y resolution"=100001, "X offset (um)"=0.0, "Y offset (um)"=0.0, "X center (um)"=0.0, "Y center (um)"=0.0, "X size (um)"=250.0, "Y size (um)"=250.0, "UL-Ang"=90.0, "UR-Ang"=90.0, "Line milling time (s)"=5.0, "Auto pause"=FALSE, "Lines auto pause"=1, "Mill from Bottom"=FALSE, "FIB FOV (um)"=500.0, "Auto Profile"=FALSE, "Mill start from Last"=FALSE, "FIB PID on"=FALSE, "FIB PID reset"=FALSE, "FIB PID measured"=0, "FIB PID target"=0.0, "FIB PID target slope"=0.0, "FIB PID P"=0.0, "FIB PID I"=0.0, "FIB PID D"=0.0}, "FI Detector"=0, "Auto Optimzation"=TRUE, "Images per Auto Optimization"=200, "AF Range (nm)"=1800.0, "AF Steps"=7, "AS Range (%)"=0.6, "AS Steps"=7, "AA Range (%)"=3.0, "AA Steps"=7, "X shift (nm/frame)"=0.0, "Y shift (nm/frame)"=0.0, "FIB Settings"={"Z-step (nm)"=2.5, "Enable alarm"=TRUE, "Label"="Emission Alarm (nA)", "Emission min"=1.2, "Emission max"=2.2, "Auto reheat"=FALSE}, "FIB Y zoom pixel (nm)"=20.0, "Mail server"="", "Email Alert Recipients"=[""], "Alert Settings"={"3D imaging paused alarm"=TRUE, "FIB emission limit warning"=TRUE, "Low limit"=1.4, "High limit"=2.0, "Specimen @ SEM alarm"=TRUE, "FIB CL current alarm"=TRUE, "Beam Dump 1 alarm"=TRUE, "Milling Y voltage alarm"=TRUE, "EHT off alarm"=TRUE, "Temperature alarm"=TRUE, "Pause 3D-ING"=FALSE, "Low limit (F)"=65.0, "High limit (F)"=80.0, "Temp limit auto"=TRUE, "Delta (F)"=0.2, "Gradient limit (F/min)"=0.03, "SW error warning"=TRUE, "Focus index warning"=TRUE, "Focus index low limit"=0.1, "Focus index stop limit"=0.0, "Run Auto Stig"=FALSE, "FI low limit auto"=TRUE, "FI stop limit auto"=TRUE}, "Reheat Parameters"={"Filament I (A)"=3.0, "Reheat time (s)"=45.0, "Emission (uA)"=2.2, "Calculate V/I slope"=TRUE, "Pre-calc delay (min)"=5.0, "Disable Reheat Retries"=FALSE, "Restore Voltages"=TRUE}, "Start FIB HV DataLog"=FALSE, "Interval (s)"=60} {"Alert Settings"."Focus index stop limit" format="%_3g"; "Alert Settings"."Focus index low limit" format="%_3g"; "Alert Settings"."High limit (F)" format="%.2g"; "Alert Settings"."Low limit (F)" format="%.2g"; "SEM Scan Parameters"."dY (um)" format="%.1f"; "SEM Scan Parameters"."dX (um)" format="%.1f"; "SEM Scan Parameters"."Frames" min=1 step=1; "SEM Scan Parameters"."WD (mm)" format="%.1f"; "SEM Scan Parameters"."Y aln" format="%.1f"; "SEM Scan Parameters"."X aln" format="%.1f"; "SEM Scan Parameters"."Y stig" format="%.1f"; "SEM Scan Parameters"."X stig" format="%.1f"; "SEM Scan Parameters"."Overlap (um)" min=0; "SEM Scan Parameters"."Y tiles" min=1; "SEM Scan Parameters"."X tiles" min=1; "SEM Scan Parameters"."X size (um)" format="%.2f"; "SEM Scan Parameters"."Y size (um)" format="%.2f"; "SEM Scan Parameters"."Frame line rampdown ratio" min=0 max=1 step=0.05 format="%.2g"; "SEM Scan Parameters"."X center (um)" step=1.0 format="%.2f"; "SEM Scan Parameters"."Y center (um)" step=1.0 format="%.2f"; "SEM Scan Parameters"."X size (V)" format="%_4g"; "SEM Scan Parameters"."Scan rate (Hz)" max=4000000 step=100000 format="%.2e"; "Reheat Parameters"."Pre-calc delay (min)" format="%.2f"; "Reheat Parameters"."Emission (uA)" format="%.1f"; "Reheat Parameters"."Filament I (A)" format="%.2f"; "Reheat Parameters"."Reheat time (s)" format="%.1f"; "Image fit to" items=["Width", "Height"]; "Mid Mag SEM"."X center (um)" step=1.0 format="%.4f"; "Mid Mag SEM"."Y center (um)" step=1.0 format="%.4f"; "Mid Mag SEM"."Mid mag interval" min=1 step=1; "Mid Mag SEM"."Mid mag scan rate (Hz)" max=4000000 step=100000 format="%.2e"; "Milling para"."FIB PID measured" items=["Spec.", "B.D.1", "B.D.2", "Mill"]; "Milling para"."UR-Ang" format="%.2f"; "Milling para"."UL-Ang" format="%.2f"; "Milling para"."Y offset (um)" step=0.02 format="%.3g"; "Milling para"."X offset (um)" step=1 format="%.3g"; "Milling para"."FIB FOV (um)" format="%.3g"; "Milling para"."Line milling time (s)" format="%.1f"; "Milling para"."Y center (um)" format="%#.3g"; "Milling para"."X center (um)" format="%#.3g"; "Focus Index grid X" min=1; "Focus Index grid Y" min=1; "FIB Y zoom pixel (nm)" format="%.1g"; "FIB Settings"."Emission min" format="%.1g"; "FIB Settings"."Emission max" format="%.1g"; "X shift (nm/frame)" step=0.1; "Y shift (nm/frame)" step=0.1; "FI Detector" items=["A", "B", "C", "D"]; "Low mag SEM"."Low mag interval" min=1 step=1; "Low mag SEM"."Low mag scan rate (Hz)" max=4000000 step=100000 format="%.2e"; "Low mag SEM"."Low mag scan FOV (micron)" step=50.0; "FIB-SEM Angle" min=0.0 max=90.0}
  # "Images"
  # "nm"
  # "%"
  # "%"
  # "Direction"
  # "Start\nfrom"
  # "<"
  # "Grids"
  # "Primary"
  # "Det"
  # "Recipe"
  # "Brightness & Contrast (%)"
  # "Detector A"
  # "Brightness & Contrast (%)"
  # "Images"
  # "nm"
  # "%"
  # "%"
  # "Grids"
  # "Primary"
  # "Direction"
  # "Start\nfrom"
  # "Det"
  # "Recipe"
  # "Brightness & Contrast (%)"
  # "Detector A"
  # "Brightness & Contrast (%)"
  # "Images"
  # "nm"
  # "%"
  # "%"
  # "Direction"
  # "Start\nfrom"
  # "Det"
  # "Recipe"
  # "Brightness & Contrast (%)"
  # "Detector A"
  # "Brightness & Contrast (%)"
  # "Images"
  # "nm"
  # "%"
  # "%"
  # "Direction"
  # "Start\nfrom"
  # "Det"
  # "Recipe"
  # "Brightness & Contrast (%)"
  # "Detector A"
  # "Brightness & Contrast (%)"
  # "Images"
  # "nm"
  # "%"
  # "%"
  # "Direction"
  # "Start\nfrom"
  # "Det"
  # "Recipe"
  # "Brightness & Contrast (%)"
  # "Detector A"
  # "Brightness & Contrast (%)"
  # "Images"
  # "nm"
  # "%"
  # "%"
  # "Direction"
  # "Start\nfrom"
  # "<"
  # "Grids"
  # "Primary"
  # "Det"
  # "Recipe"
  # "Brightness & Contrast (%)"
  # "Detector A"
  # "Brightness & Contrast (%)"
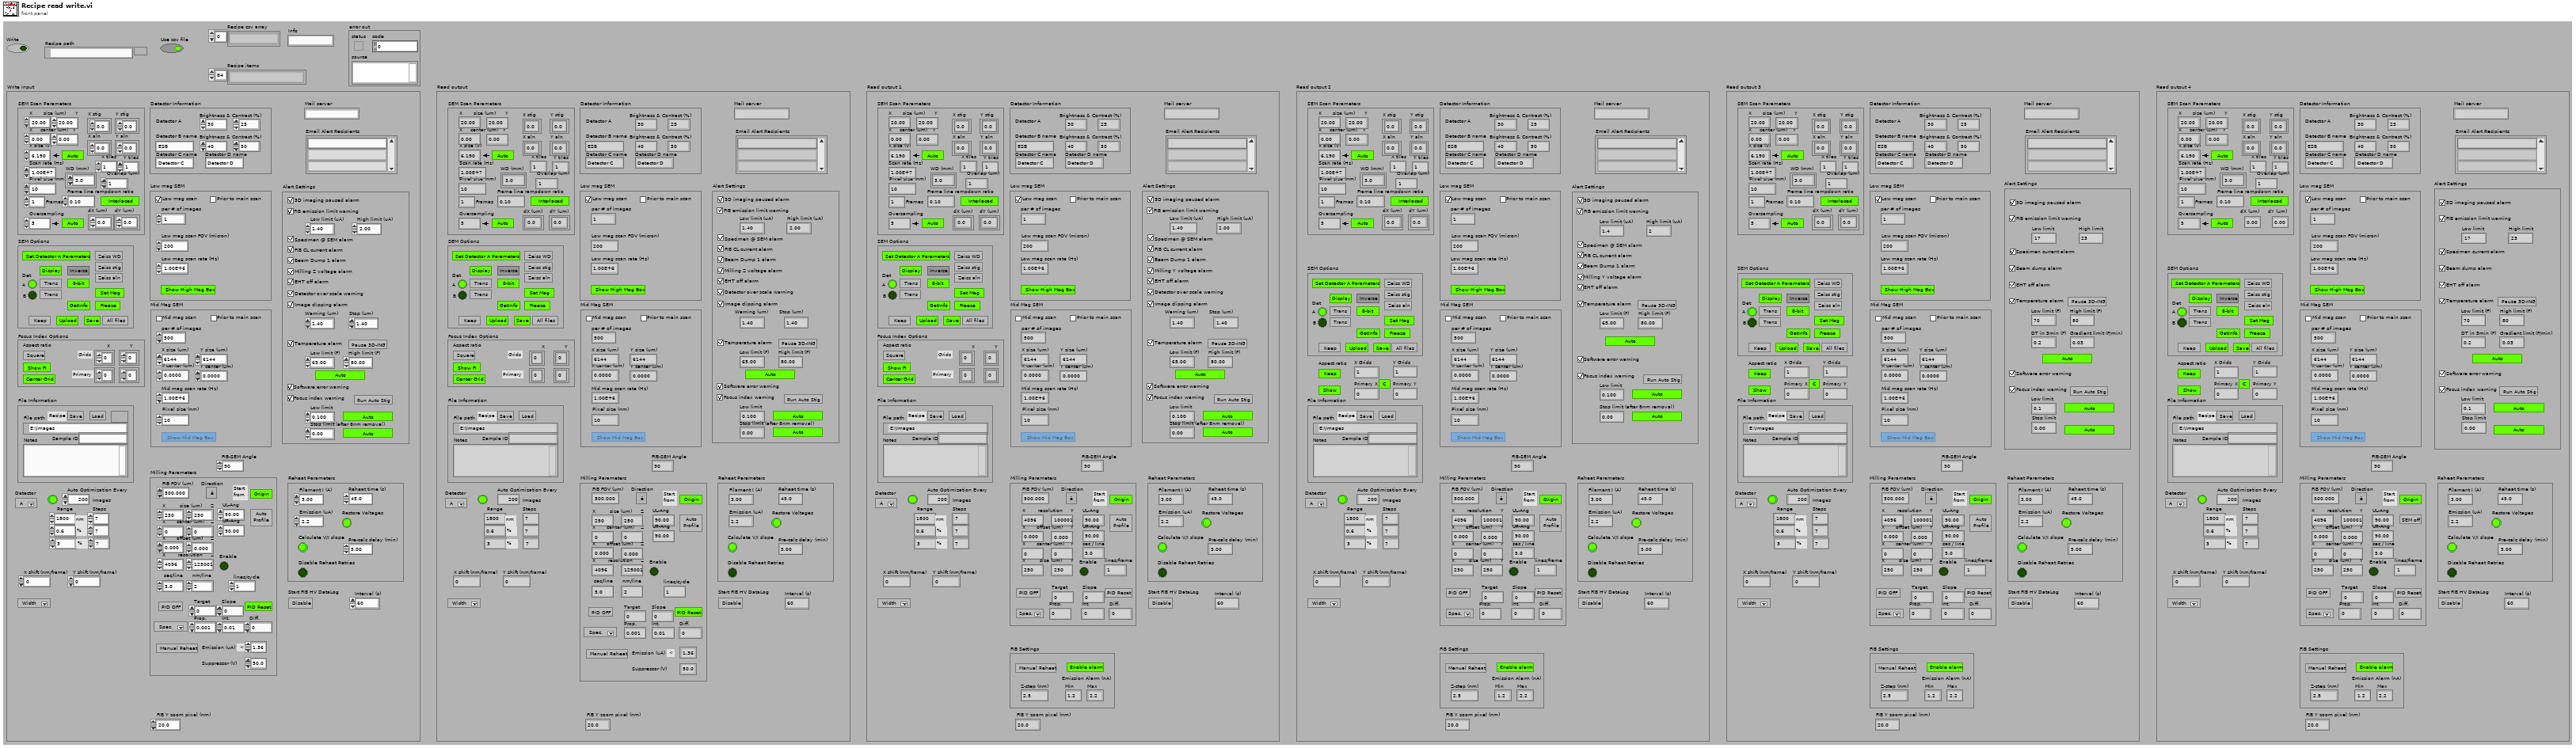
[diagram p1: front panel]
types:
  T1 = cluster{"SEM Scan Parameters":cluster{"X size (um)":sgl, "Y size (um)":sgl, "X center (um)":dbl, "Y center (um)":dbl, "X size (V)":dbl, "X size auto":bool, "X stig":sgl[][], "Y stig":sgl[][], "X aln":sgl[][], "Y aln":sgl[][], "Scan rate (Hz)":u32, "Oversampling":u32, "Oversampling auto":bool, "Frame line rampdown ratio":sgl, "Pixel size (nm)":sgl, "WD (mm)":sgl[][], "X tiles":u8, "Y tiles":u8, "Overlap (um)":sgl, "Interlaced":bool, "dX (um)":sgl[], "dY (um)":sgl[], "Frames":u8}, "Detector Information":cluster{"Brightness A":dbl, "Contrast A":dbl, "Detector B name":string, "Brightness B":dbl, "Contrast B":dbl, "Detector C name":string, "Detector D name":string}, "SEM Options":cluster{"GetInfo":bool, "Set Det A para":bool, "Set WD":bool, "Set Mag":bool, "Set stig":bool, "Set aln":bool, "Display":bool, "Save":bool, "8-bit":bool, "Detector A":bool, "Detector B":bool, "Detector C":bool, "Detector D":bool, "Inverse A":bool, "Inverse B":bool, "Inverse C":bool, "Inverse D":bool, "Inverse PNG":bool, "Freeze":bool, "PNG only":bool, "Upload":bool, "Delete after upload":bool}, "Focus Index Options":cluster{"Keep aspect ratio":bool, "Show Focus Index":bool, "Focus Index primary grid center":bool, "X Grids":u8[][], "Y Grids":u8[][], "Primary X index":u8[][], "Primary Y index":u8[][]}, "Image fit to":u8, "File Information":cluster{"File path":path, "Notes":string, "Save recipe":bool, "Load recipe":bool, "Sample ID":string}, "Low mag SEM":cluster{"Low mag scan":bool, "Prior to main scan":bool, "Low mag interval":u32, "Low mag scan FOV (micron)":dbl, "Low mag scan rate (Hz)":u32, "Show HM box":bool}, "Mid Mag SEM":cluster{"Mid mag scan":bool, "Prior to main scan":bool, "Mid mag interval":u32, "X size (um)":sgl, "Y size (um)":sgl, "X center (um)":dbl, "Y center (um)":dbl, "Mid mag scan rate (Hz)":u32, "Pixel size (nm)":dbl, "Show MM box":bool}, "FIB-SEM Angle":dbl, "Milling para":cluster{"X resolution":u32, "Z resolution":u32, "X offset (um)":sgl, "Z offset (um)":sgl, "X center (um)":sgl, "Z center (um)":sgl, "X size (um)":sgl, "Z size (um)":sgl, "UL-Ang":sgl, "UR-Ang":sgl, "Line milling time (s)":sgl, "Z-step (nm)":dbl, "Lines auto pause":u16, "Auto pause":bool, "Mill from Bottom":bool, "FIB FOV (um)":sgl, "Auto Profile":bool, "Mill start from Last":bool, "FIB PID on":bool, "FIB PID reset":bool, "FIB PID measured":u8, "FIB PID target":sgl, "FIB PID target slope":sgl, "FIB PID P":sgl, "FIB PID I":sgl, "FIB PID D":sgl, "Emission (uA)":dbl, "Suppressor (V)":sgl, "Auto reheat":bool}, "FI Detector":u16, "Auto Optimzation":bool, "Images per Auto Optimization":u16, "AF Range (nm)":sgl, "AF Steps":u8, "AS Range (%)":sgl, "AS Steps":u8, "AA Range (%)":sgl, "AA Steps":u8, "X shift (nm/frame)":dbl, "Y shift (nm/frame)":dbl, "FIB Y zoom pixel (nm)":dbl, "Mail server":string, "Email Alert Recipients":string[], "Alert Settings":cluster{"3D imaging paused alarm":bool, "FIB emission limit warning":bool, "Low limit":sgl, "High limit":sgl, "Specimen @ SEM alarm":bool, "FIB CL current alarm":bool, "Beam Dump 1 alarm":bool, "Milling Z voltage alarm":bool, "EHT off alarm":bool, "Detector over scale warning":bool, "Image clipping alarm":bool, "Warning limit (um)":sgl, "Stop limit (um)":sgl, "Temperature alarm":bool, "Pause 3D-ING":bool, "Low limit (F)":sgl, "High limit (F)":sgl, "Temp limit auto":bool, "Delta (F)":sgl, "Gradient limit (F/min)":sgl, "SW error warning":bool, "Focus index warning":bool, "Focus index low limit":sgl, "Focus index stop limit":sgl, "Run Auto Stig":bool, "FI low limit auto":bool, "FI stop limit auto":bool}, "Reheat Parameters":cluster{"Filament I (A)":sgl, "Reheat time (s)":sgl, "Emission (uA)":sgl, "Calculate V/I slope":bool, "Pre-calc delay (min)":sgl, "Disable Reheat Retries":bool, "Restore Voltages":bool}, "Start FIB HV DataLog":bool, "Interval (s)":u16}
  T2 = cluster{"SEM Scan Parameters":cluster{"X size (um)":sgl, "Y size (um)":sgl, "X center (um)":dbl, "Y center (um)":dbl, "X size (V)":dbl, "X size auto":bool, "X stig":sgl[][], "Y stig":sgl[][], "X aln":sgl[][], "Y aln":sgl[][], "Scan rate (Hz)":u32, "Oversampling":u32, "Oversampling auto":bool, "Frame line rampdown ratio":sgl, "Pixel size (nm)":sgl, "WD (mm)":sgl[][], "X tiles":u8, "Y tiles":u8, "Overlap (um)":sgl, "Interlaced":bool, "dX (um)":sgl[], "dY (um)":sgl[], "Frames":u8}, "Detector Information":cluster{"Brightness A":dbl, "Contrast A":dbl, "Detector B name":string, "Brightness B":dbl, "Contrast B":dbl, "Detector C name":string, "Detector D name":string}, "SEM Options":cluster{"GetInfo":bool, "Set Det A para":bool, "Set WD":bool, "Set Mag":bool, "Set stig":bool, "Set aln":bool, "Display":bool, "Save":bool, "8-bit":bool, "Detector A":bool, "Detector B":bool, "Detector C":bool, "Detector D":bool, "Inverse A":bool, "Inverse B":bool, "Inverse C":bool, "Inverse D":bool, "Inverse PNG":bool, "Freeze":bool, "PNG only":bool, "Upload":bool, "Delete after upload":bool}, "Focus Index Options":cluster{"Keep aspect ratio":bool, "Show Focus Index":bool, "Focus Index primary grid center":bool, "X Grids":u8[][], "Y Grids":u8[][], "Primary X index":u8[][], "Primary Y index":u8[][]}, "Image fit to":u8, "File Information":cluster{"File path":path, "Notes":string, "Save recipe":bool, "Load recipe":bool, "Sample ID":string}, "Low mag SEM":cluster{"Low mag scan":bool, "Prior to main scan":bool, "Low mag interval":u32, "Low mag scan FOV (micron)":dbl, "Low mag scan rate (Hz)":u32, "Show HM box":bool}, "Mid Mag SEM":cluster{"Mid mag scan":bool, "Prior to main scan":bool, "Mid mag interval":u32, "X size (um)":sgl, "Y size (um)":sgl, "X center (um)":dbl, "Y center (um)":dbl, "Mid mag scan rate (Hz)":u32, "Pixel size (nm)":dbl, "Show MM box":bool}, "FIB-SEM Angle":dbl, "Milling para":cluster{"X resolution":u32, "Y resolution":u32, "X offset (um)":sgl, "Y offset (um)":sgl, "X center (um)":sgl, "Y center (um)":sgl, "X size (um)":sgl, "Y size (um)":sgl, "UL-Ang":sgl, "UR-Ang":sgl, "Line milling time (s)":sgl, "Auto pause":bool, "Lines auto pause":u16, "Mill from Bottom":bool, "FIB FOV (um)":sgl, "Auto Profile":bool, "Mill start from Last":bool, "FIB PID on":bool, "FIB PID reset":bool, "FIB PID measured":u8, "FIB PID target":sgl, "FIB PID target slope":sgl, "FIB PID P":sgl, "FIB PID I":sgl, "FIB PID D":sgl}, "FI Detector":u16, "Auto Optimzation":bool, "Images per Auto Optimization":u16, "AF Range (nm)":sgl, "AF Steps":u8, "AS Range (%)":sgl, "AS Steps":u8, "AA Range (%)":sgl, "AA Steps":u8, "X shift (nm/frame)":dbl, "Y shift (nm/frame)":dbl, "FIB Settings":cluster{"Z-step (nm)":dbl, "Enable alarm":bool, "Label":string, "Emission min":dbl, "Emission max":dbl, "Auto reheat":bool}, "FIB Y zoom pixel (nm)":dbl, "Mail server":string, "Email Alert Recipients":string[], "Alert Settings":cluster{"3D imaging paused alarm":bool, "FIB emission limit warning":bool, "Low limit":sgl, "High limit":sgl, "Specimen @ SEM alarm":bool, "FIB CL current alarm":bool, "Beam Dump 1 alarm":bool, "Milling Y voltage alarm":bool, "EHT off alarm":bool, "Detector over scale warning":bool, "Image clipping alarm":bool, "Warning limit (um)":sgl, "Stop limit (um)":sgl, "Temperature alarm":bool, "Pause 3D-ING":bool, "Low limit (F)":sgl, "High limit (F)":sgl, "Temp limit auto":bool, "Delta (F)":sgl, "Gradient limit (F/min)":sgl, "SW error warning":bool, "Focus index warning":bool, "Focus index low limit":sgl, "Focus index stop limit":sgl, "Run Auto Stig":bool, "FI low limit auto":bool, "FI stop limit auto":bool}, "Reheat Parameters":cluster{"Filament I (A)":sgl, "Reheat time (s)":sgl, "Emission (uA)":sgl, "Calculate V/I slope":bool, "Pre-calc delay (min)":sgl, "Disable Reheat Retries":bool, "Restore Voltages":bool}, "Start FIB HV DataLog":bool, "Interval (s)":u16}
  T3 = cluster{"SEM Scan Parameters":cluster{"X size (um)":sgl, "Y size (um)":sgl, "X center (um)":dbl, "Y center (um)":dbl, "X size (V)":dbl, "X size auto":bool, "X stig":sgl[][], "Y stig":sgl[][], "X aln":sgl[][], "Y aln":sgl[][], "Scan rate (Hz)":u32, "Oversampling":u32, "Oversampling auto":bool, "Frame line rampdown ratio":sgl, "Pixel size (nm)":sgl, "WD (mm)":sgl[][], "X tiles":u8, "Y tiles":u8, "Overlap (um)":sgl, "Interlaced":bool, "dX (um)":sgl[], "dY (um)":sgl[], "Frames":u8}, "Detector Information":cluster{"Brightness A":dbl, "Contrast A":dbl, "Detector B name":string, "Brightness B":dbl, "Contrast B":dbl, "Detector C name":string, "Detector D name":string}, "SEM Options":cluster{"GetInfo":bool, "Set Det A para":bool, "Set WD":bool, "Set Mag":bool, "Set stig":bool, "Set aln":bool, "Display":bool, "Save":bool, "8-bit":bool, "Detector A":bool, "Detector B":bool, "Detector C":bool, "Detector D":bool, "Inverse A":bool, "Inverse B":bool, "Inverse C":bool, "Inverse D":bool, "Inverse PNG":bool, "Freeze":bool, "PNG only":bool, "Upload":bool, "Delete after upload":bool}, "Keep aspect ratio":bool, "Show Focus Index":bool, "Focus Index primary grid center":bool, "Focus Index grid X":u8, "Focus Index grid Y":u8, "Focus Index primary X grid":u8, "Focus Index primary Y grid":u8, "Image fit to":u8, "File Information":cluster{"File path":path, "Notes":string, "Save recipe":bool, "Load recipe":bool, "Sample ID":string}, "Low mag SEM":cluster{"Low mag scan":bool, "Prior to main scan":bool, "Low mag interval":u32, "Low mag scan FOV (micron)":dbl, "Low mag scan rate (Hz)":u32, "Show HM box":bool}, "Mid Mag SEM":cluster{"Mid mag scan":bool, "Prior to main scan":bool, "Mid mag interval":u32, "X size (um)":sgl, "Y size (um)":sgl, "X center (um)":dbl, "Y center (um)":dbl, "Mid mag scan rate (Hz)":u32, "Pixel size (nm)":dbl, "Show MM box":bool}, "FIB-SEM Angle":dbl, "Milling para":cluster{"X resolution":u32, "Y resolution":u32, "X offset (um)":sgl, "Y offset (um)":sgl, "X center (um)":sgl, "Y center (um)":sgl, "X size (um)":sgl, "Y size (um)":sgl, "UL-Ang":sgl, "UR-Ang":sgl, "Line milling time (s)":sgl, "Auto pause":bool, "Lines auto pause":u16, "Mill from Bottom":bool, "FIB FOV (um)":sgl, "Auto Profile":bool, "Mill start from Last":bool, "FIB PID on":bool, "FIB PID reset":bool, "FIB PID measured":u8, "FIB PID target":sgl, "FIB PID target slope":sgl, "FIB PID P":sgl, "FIB PID I":sgl, "FIB PID D":sgl}, "FI Detector":u16, "Auto Optimzation":bool, "Images per Auto Optimization":u16, "AF Range (nm)":sgl, "AF Steps":u8, "AS Range (%)":sgl, "AS Steps":u8, "AA Range (%)":sgl, "AA Steps":u8, "X shift (nm/frame)":dbl, "Y shift (nm/frame)":dbl, "FIB Settings":cluster{"Z-step (nm)":dbl, "Enable alarm":bool, "Label":string, "Emission min":dbl, "Emission max":dbl, "Auto reheat":bool}, "FIB Y zoom pixel (nm)":dbl, "Mail server":string, "Email Alert Recipients":string[], "Alert Settings":cluster{"3D imaging paused alarm":bool, "FIB emission limit warning":bool, "Low limit":dbl, "High limit":dbl, "Specimen current alarm ":bool, "Beam dump alarm":bool, "EHT off alarm":bool, "Temperature alarm":bool, "Pause 3D-ING":bool, "Low limit (F)":sgl, "High limit (F)":sgl, "Temp limit auto":bool, "Delta (F)":sgl, "Gradient limit (F/min)":sgl, "SW error warning":bool, "Focus index warning":bool, "Focus index low limit":dbl, "Focus index stop limit":sgl, "Run Auto Stig":bool, "FI low limit auto":bool, "FI stop limit auto":bool}, "Reheat Parameters":cluster{"Filament I (A)":sgl, "Reheat time (s)":sgl, "Emission (uA)":sgl, "Calculate V/I slope":bool, "Pre-calc delay (min)":sgl, "Disable Reheat Retries":bool, "Restore Voltages":bool}, "Start FIB HV DataLog":bool, "Interval (s)":u16}
  T4 = cluster{"SEM Scan Parameters":cluster{"X size (um)":sgl, "Y size (um)":sgl, "X center (um)":dbl, "Y center (um)":dbl, "X size (V)":dbl, "X size auto":bool, "X stig":sgl[][], "Y stig":sgl[][], "X aln":sgl[][], "Y aln":sgl[][], "Scan rate (Hz)":u32, "Oversampling":u32, "Oversampling auto":bool, "Frame line rampdown ratio":sgl, "Pixel size (nm)":sgl, "WD (mm)":sgl[][], "X tiles":u8, "Y tiles":u8, "Overlap (um)":sgl, "Interlaced":bool, "dX (um)":sgl, "dY (um)":sgl, "Frames":u8}, "Detector Information":cluster{"Brightness A":dbl, "Contrast A":dbl, "Detector B name":string, "Brightness B":dbl, "Contrast B":dbl, "Detector C name":string, "Detector D name":string}, "SEM Options":cluster{"GetInfo":bool, "Set Det A para":bool, "Set WD":bool, "Set Mag":bool, "Set stig":bool, "Set aln":bool, "Display":bool, "Save":bool, "8-bit":bool, "Detector A":bool, "Detector B":bool, "Detector C":bool, "Detector D":bool, "Inverse A":bool, "Inverse B":bool, "Inverse C":bool, "Inverse D":bool, "Inverse PNG":bool, "Freeze":bool, "PNG only":bool, "Upload":bool, "Delete after upload":bool}, "Keep aspect ratio":bool, "Show Focus Index":bool, "Focus Index primary grid center":bool, "Focus Index grid X":u8, "Focus Index grid Y":u8, "Focus Index primary X grid":u8, "Focus Index primary Y grid":u8, "Image fit to":u8, "File Information":cluster{"File path":path, "Notes":string, "Save recipe":bool, "Load recipe":bool, "Sample ID":string}, "Low mag SEM":cluster{"Low mag scan":bool, "Prior to main scan":bool, "Low mag interval":u32, "Low mag scan FOV (micron)":dbl, "Low mag scan rate (Hz)":u32, "Show HM box":bool}, "Mid Mag SEM":cluster{"Mid mag scan":bool, "Prior to main scan":bool, "Mid mag interval":u32, "X size (um)":sgl, "Y size (um)":sgl, "X center (um)":dbl, "Y center (um)":dbl, "Mid mag scan rate (Hz)":u32, "Pixel size (nm)":dbl, "Show MM box":bool}, "FIB-SEM Angle":dbl, "Milling para":cluster{"X resolution":u32, "Y resolution":u32, "X offset (um)":sgl, "Y offset (um)":sgl, "X center (um)":sgl, "Y center (um)":sgl, "X size (um)":sgl, "Y size (um)":sgl, "UL-Ang":sgl, "UR-Ang":sgl, "Line milling time (s)":sgl, "Auto pause":bool, "Lines auto pause":u16, "Mill from Bottom":bool, "FIB FOV (um)":sgl, "SEM on":bool, "Mill start from Last":bool, "FIB PID on":bool, "FIB PID reset":bool, "FIB PID measured":u8, "FIB PID target":sgl, "FIB PID target slope":sgl, "FIB PID P":sgl, "FIB PID I":sgl, "FIB PID D":sgl}, "FI Detector":u16, "Auto Optimzation":bool, "Images per Auto Optimization":u16, "AF Range (nm)":sgl, "AF Steps":u8, "AS Range (%)":sgl, "AS Steps":u8, "AA Range (%)":sgl, "AA Steps":u8, "X shift (nm/frame)":dbl, "Y shift (nm/frame)":dbl, "FIB Settings":cluster{"Z-step (nm)":dbl, "Enable alarm":bool, "Label":string, "Emission min":dbl, "Emission max":dbl, "Auto reheat":bool}, "FIB Y zoom pixel (nm)":dbl, "Mail server":string, "Email Alert Recipients":string[], "Alert Settings":cluster{"3D imaging paused alarm":bool, "FIB emission limit warning":bool, "Low limit":dbl, "High limit":dbl, "Specimen current alarm ":bool, "Beam dump alarm":bool, "EHT off alarm":bool, "Temperature alarm":bool, "Pause 3D-ING":bool, "Low limit (F)":sgl, "High limit (F)":sgl, "Temp limit auto":bool, "Delta (F)":sgl, "Gradient limit (F/min)":sgl, "SW error warning":bool, "Focus index warning":bool, "Focus index low limit":dbl, "Focus index stop limit":sgl, "Run Auto Stig":bool, "FI low limit auto":bool, "FI stop limit auto":bool}, "Reheat Parameters":cluster{"Filament I (A)":sgl, "Reheat time (s)":sgl, "Emission (uA)":sgl, "Calculate V/I slope":bool, "Pre-calc delay (min)":sgl, "Disable Reheat Retries":bool, "Restore Voltages":bool}, "Start FIB HV DataLog":bool, "Interval (s)":u16}
  T5 = cluster{"SEM Scan Parameters":cluster{"X size (um)":sgl, "Y size (um)":sgl, "X center (um)":dbl, "Y center (um)":dbl, "X size (V)":dbl, "X size auto":bool, "X stig":sgl[][], "Y stig":sgl[][], "X aln":sgl[][], "Y aln":sgl[][], "Scan rate (Hz)":u32, "Oversampling":u32, "Oversampling auto":bool, "Frame line rampdown ratio":sgl, "Pixel size (nm)":sgl, "WD (mm)":sgl[][], "X tiles":u8, "Y tiles":u8, "Overlap (um)":sgl, "Interlaced":bool, "dX (um)":sgl[], "dY (um)":sgl[], "Frames":u8}, "Detector Information":cluster{"Brightness A":dbl, "Contrast A":dbl, "Detector B name":string, "Brightness B":dbl, "Contrast B":dbl, "Detector C name":string, "Detector D name":string}, "SEM Options":cluster{"GetInfo":bool, "Set Det A para":bool, "Set WD":bool, "Set Mag":bool, "Set stig":bool, "Set aln":bool, "Display":bool, "Save":bool, "8-bit":bool, "Detector A":bool, "Detector B":bool, "Detector C":bool, "Detector D":bool, "Inverse A":bool, "Inverse B":bool, "Inverse C":bool, "Inverse D":bool, "Inverse PNG":bool, "Freeze":bool, "PNG only":bool, "Upload":bool, "Delete after upload":bool}, "Keep aspect ratio":bool, "Show Focus Index":bool, "Focus Index primary grid center":bool, "Focus Index grid X":u8, "Focus Index grid Y":u8, "Focus Index primary X grid":u8, "Focus Index primary Y grid":u8, "Image fit to":u8, "File Information":cluster{"File path":path, "Notes":string, "Save recipe":bool, "Load recipe":bool, "Sample ID":string}, "Low mag SEM":cluster{"Low mag scan":bool, "Prior to main scan":bool, "Low mag interval":u32, "Low mag scan FOV (micron)":dbl, "Low mag scan rate (Hz)":u32, "Show HM box":bool}, "Mid Mag SEM":cluster{"Mid mag scan":bool, "Prior to main scan":bool, "Mid mag interval":u32, "X size (um)":sgl, "Y size (um)":sgl, "X center (um)":dbl, "Y center (um)":dbl, "Mid mag scan rate (Hz)":u32, "Pixel size (nm)":dbl, "Show MM box":bool}, "FIB-SEM Angle":dbl, "Milling para":cluster{"X resolution":u32, "Y resolution":u32, "X offset (um)":sgl, "Y offset (um)":sgl, "X center (um)":sgl, "Y center (um)":sgl, "X size (um)":sgl, "Y size (um)":sgl, "UL-Ang":sgl, "UR-Ang":sgl, "Line milling time (s)":sgl, "Auto pause":bool, "Lines auto pause":u16, "Mill from Bottom":bool, "FIB FOV (um)":sgl, "Auto Profile":bool, "Mill start from Last":bool, "FIB PID on":bool, "FIB PID reset":bool, "FIB PID measured":u8, "FIB PID target":sgl, "FIB PID target slope":sgl, "FIB PID P":sgl, "FIB PID I":sgl, "FIB PID D":sgl}, "FI Detector":u16, "Auto Optimzation":bool, "Images per Auto Optimization":u16, "AF Range (nm)":sgl, "AF Steps":u8, "AS Range (%)":sgl, "AS Steps":u8, "AA Range (%)":sgl, "AA Steps":u8, "X shift (nm/frame)":dbl, "Y shift (nm/frame)":dbl, "FIB Settings":cluster{"Z-step (nm)":dbl, "Enable alarm":bool, "Label":string, "Emission min":dbl, "Emission max":dbl, "Auto reheat":bool}, "FIB Y zoom pixel (nm)":dbl, "Mail server":string, "Email Alert Recipients":string[], "Alert Settings":cluster{"3D imaging paused alarm":bool, "FIB emission limit warning":bool, "Low limit":dbl, "High limit":dbl, "Specimen @ SEM alarm":bool, "FIB CL current alarm":bool, "Beam Dump 1 alarm":bool, "Milling Y voltage alarm":bool, "EHT off alarm":bool, "Temperature alarm":bool, "Pause 3D-ING":bool, "Low limit (F)":sgl, "High limit (F)":sgl, "Temp limit auto":bool, "Delta (F)":sgl, "Gradient limit (F/min)":sgl, "SW error warning":bool, "Focus index warning":bool, "Focus index low limit":sgl, "Focus index stop limit":sgl, "Run Auto Stig":bool, "FI low limit auto":bool, "FI stop limit auto":bool}, "Reheat Parameters":cluster{"Filament I (A)":sgl, "Reheat time (s)":sgl, "Emission (uA)":sgl, "Calculate V/I slope":bool, "Pre-calc delay (min)":sgl, "Disable Reheat Retries":bool, "Restore Voltages":bool}, "Start FIB HV DataLog":bool, "Interval (s)":u16}
  T6 = enum16{"open", "replace", "create", "open or create", "replace or create", "replace or create with confirmation"}
  T7 = cluster{"X size (um)":sgl, "Y size (um)":sgl, "X center (um)":dbl, "Y center (um)":dbl, "X size (V)":dbl, "X size auto":bool, "X stig":sgl[][], "Y stig":sgl[][], "X aln":sgl[][], "Y aln":sgl[][], "Scan rate (Hz)":u32, "Oversampling":u32, "Oversampling auto":bool, "Frame line rampdown ratio":sgl, "Pixel size (nm)":sgl, "WD (mm)":sgl[][], "X tiles":u8, "Y tiles":u8, "Overlap (um)":sgl, "Interlaced":bool, "dX (um)":sgl, "dY (um)":sgl, "Frames":u8}
  T8 = cluster{"Brightness A":dbl, "Contrast A":dbl, "Detector B name":string, "Brightness B":dbl, "Contrast B":dbl, "Detector C name":string, "Detector D name":string}
  T9 = cluster{"GetInfo":bool, "Set Det A para":bool, "Set WD":bool, "Set Mag":bool, "Set stig":bool, "Set aln":bool, "Display":bool, "Save":bool, "8-bit":bool, "Detector A":bool, "Detector B":bool, "Detector C":bool, "Detector D":bool, "Inverse A":bool, "Inverse B":bool, "Inverse C":bool, "Inverse D":bool, "Inverse PNG":bool, "Freeze":bool, "PNG only":bool, "Upload":bool, "Delete after upload":bool}
  T10 = cluster{"File path":path, "Notes":string, "Save recipe":bool, "Load recipe":bool, "Sample ID":string}
  T11 = cluster{"Low mag scan":bool, "Prior to main scan":bool, "Low mag interval":u32, "Low mag scan FOV (micron)":dbl, "Low mag scan rate (Hz)":u32, "Show HM box":bool}
  T12 = cluster{"Mid mag scan":bool, "Prior to main scan":bool, "Mid mag interval":u32, "X size (um)":sgl, "Y size (um)":sgl, "X center (um)":dbl, "Y center (um)":dbl, "Mid mag scan rate (Hz)":u32, "Pixel size (nm)":dbl, "Show MM box":bool}
  T13 = cluster{"X resolution":u32, "Y resolution":u32, "X offset (um)":sgl, "Y offset (um)":sgl, "X center (um)":sgl, "Y center (um)":sgl, "X size (um)":sgl, "Y size (um)":sgl, "UL-Ang":sgl, "UR-Ang":sgl, "Line milling time (s)":sgl, "Auto pause":bool, "Lines auto pause":u16, "Mill from Bottom":bool, "FIB FOV (um)":sgl, "SEM on":bool, "Mill start from Last":bool, "FIB PID on":bool, "FIB PID reset":bool, "FIB PID measured":u8, "FIB PID target":sgl, "FIB PID target slope":sgl, "FIB PID P":sgl, "FIB PID I":sgl, "FIB PID D":sgl}
  T14 = cluster{"Z-step (nm)":dbl, "Enable alarm":bool, "Label":string, "Emission min":dbl, "Emission max":dbl, "Auto reheat":bool}
  T15 = cluster{"3D imaging paused alarm":bool, "FIB emission limit warning":bool, "Low limit":dbl, "High limit":dbl, "Specimen current alarm ":bool, "Beam dump alarm":bool, "EHT off alarm":bool, "Temperature alarm":bool, "Pause 3D-ING":bool, "Low limit (F)":sgl, "High limit (F)":sgl, "Temp limit auto":bool, "Delta (F)":sgl, "Gradient limit (F/min)":sgl, "SW error warning":bool, "Focus index warning":bool, "Focus index low limit":dbl, "Focus index stop limit":sgl, "Run Auto Stig":bool, "FI low limit auto":bool, "FI stop limit auto":bool}
  T16 = cluster{"Filament I (A)":sgl, "Reheat time (s)":sgl, "Emission (uA)":sgl, "Calculate V/I slope":bool, "Pre-calc delay (min)":sgl, "Disable Reheat Retries":bool, "Restore Voltages":bool}
  T17 = cluster{"X size (um)":sgl, "Y size (um)":sgl, "X center (um)":dbl, "Y center (um)":dbl, "X size (V)":dbl, "X size auto":bool, "X stig":sgl[][], "Y stig":sgl[][], "X aln":sgl[][], "Y aln":sgl[][], "Scan rate (Hz)":u32, "Oversampling":u32, "Oversampling auto":bool, "Frame line rampdown ratio":sgl, "Pixel size (nm)":sgl, "WD (mm)":sgl[][], "X tiles":u8, "Y tiles":u8, "Overlap (um)":sgl, "Interlaced":bool, sgl[], sgl[], "X tiles":u8}
  T18 = cluster{"X resolution":u32, "Y resolution":u32, "X offset (um)":sgl, "Y offset (um)":sgl, "X center (um)":sgl, "Y center (um)":sgl, "X size (um)":sgl, "Y size (um)":sgl, "UL-Ang":sgl, "UR-Ang":sgl, "Line milling time (s)":sgl, "Z-step (nm)":dbl, "Lines auto pause":u16, "Auto pause":bool, "Mill from Bottom":bool, "FIB FOV (um)":sgl, "SEM on":bool, "Mill start from Last":bool, "FIB PID on":bool, "FIB PID reset":bool, "FIB PID measured":u8, "FIB PID target":sgl, "FIB PID target slope":sgl, "FIB PID P":sgl, "FIB PID I":sgl, "FIB PID D":sgl, "Emission min":dbl, "Emission min":dbl, "Auto reheat":bool}
  T19 = cluster{"3D imaging paused alarm":bool, "FIB emission limit warning":bool, "Low limit":dbl, "High limit":dbl, "Pause 3D-ING":bool, "Specimen current alarm ":bool, "Beam dump alarm":bool, "Pause 3D-ING":bool, "EHT off alarm":bool, "Pause 3D-ING":bool, "Pause 3D-ING":bool, "Low limit":sgl, "Low limit":sgl, "Temperature alarm":bool, "Pause 3D-ING":bool, "Low limit (F)":sgl, "High limit (F)":sgl, "Temp limit auto":bool, "Delta (F)":sgl, "Gradient limit (F/min)":sgl, "SW error warning":bool, "Focus index warning":bool, "Focus index low limit":dbl, "Focus index stop limit":sgl, "Run Auto Stig":bool, "FI low limit auto":bool, "FI stop limit auto":bool}
  T20 = cluster{"X size (um)":sgl, "Y size (um)":sgl, "X center (um)":dbl, "Y center (um)":dbl, "X size (V)":dbl, "X size auto":bool, "X stig":sgl[][], "Y stig":sgl[][], "X aln":sgl[][], "Y aln":sgl[][], "Scan rate (Hz)":u32, "Oversampling":u32, "Oversampling auto":bool, "Frame line rampdown ratio":sgl, "Pixel size (nm)":sgl, "WD (mm)":sgl[][], "X tiles":u8, "Y tiles":u8, "Overlap (um)":sgl, "Interlaced":bool, "dX (um)":sgl[], "dY (um)":sgl[], "Frames":u8}
  T21 = cluster{"X resolution":u32, "Y resolution":u32, "X offset (um)":sgl, "Y offset (um)":sgl, "X center (um)":sgl, "Y center (um)":sgl, "X size (um)":sgl, "Y size (um)":sgl, "UL-Ang":sgl, "UR-Ang":sgl, "Line milling time (s)":sgl, "Auto pause":bool, "Lines auto pause":u16, "Mill from Bottom":bool, "FIB FOV (um)":sgl, "Auto Profile":bool, "Mill start from Last":bool, "FIB PID on":bool, "FIB PID reset":bool, "FIB PID measured":u8, "FIB PID target":sgl, "FIB PID target slope":sgl, "FIB PID P":sgl, "FIB PID I":sgl, "FIB PID D":sgl}
  T22 = cluster{"X resolution":u32, "Y resolution":u32, "X offset (um)":sgl, "Y offset (um)":sgl, "X center (um)":sgl, "Y center (um)":sgl, "X size (um)":sgl, "Y size (um)":sgl, "UL-Ang":sgl, "UR-Ang":sgl, "Line milling time (s)":sgl, "Z-step (nm)":dbl, "Lines auto pause":u16, "Auto pause":bool, "Mill from Bottom":bool, "FIB FOV (um)":sgl, "Auto Profile":bool, "Mill start from Last":bool, "FIB PID on":bool, "FIB PID reset":bool, "FIB PID measured":u8, "FIB PID target":sgl, "FIB PID target slope":sgl, "FIB PID P":sgl, "FIB PID I":sgl, "FIB PID D":sgl, "Emission min":dbl, "Emission min":dbl, "Auto reheat":bool}
  T23 = cluster{"3D imaging paused alarm":bool, "FIB emission limit warning":bool, "Low limit":dbl, "High limit":dbl, "Specimen @ SEM alarm":bool, "FIB CL current alarm":bool, "Beam Dump 1 alarm":bool, "Milling Y voltage alarm":bool, "EHT off alarm":bool, "Temperature alarm":bool, "Pause 3D-ING":bool, "Low limit (F)":sgl, "High limit (F)":sgl, "Temp limit auto":bool, "Delta (F)":sgl, "Gradient limit (F/min)":sgl, "SW error warning":bool, "Focus index warning":bool, "Focus index low limit":sgl, "Focus index stop limit":sgl, "Run Auto Stig":bool, "FI low limit auto":bool, "FI stop limit auto":bool}
  T24 = cluster{"3D imaging paused alarm":bool, "FIB emission limit warning":bool, "Low limit":dbl, "High limit":dbl, "Specimen @ SEM alarm":bool, "FIB CL current alarm":bool, "Beam Dump 1 alarm":bool, "Milling Y voltage alarm":bool, "EHT off alarm":bool, "Pause 3D-ING":bool, "Pause 3D-ING":bool, "Low limit":sgl, "Low limit":sgl, "Temperature alarm":bool, "Pause 3D-ING":bool, "Low limit (F)":sgl, "High limit (F)":sgl, "Temp limit auto":bool, "Delta (F)":sgl, "Gradient limit (F/min)":sgl, "SW error warning":bool, "Focus index warning":bool, "Focus index low limit":sgl, "Focus index stop limit":sgl, "Run Auto Stig":bool, "FI low limit auto":bool, "FI stop limit auto":bool}
  T25 = cluster{"Keep aspect ratio":bool, "Show Focus Index":bool, "Focus Index primary grid center":bool, "X Grids":u8[][], "Y Grids":u8[][], "Primary X index":u8[][], "Primary Y index":u8[][]}
  T26 = cluster{"3D imaging paused alarm":bool, "FIB emission limit warning":bool, "Low limit":sgl, "High limit":sgl, "Specimen @ SEM alarm":bool, "FIB CL current alarm":bool, "Beam Dump 1 alarm":bool, "Milling Y voltage alarm":bool, "EHT off alarm":bool, "Detector over scale warning":bool, "Image clipping alarm":bool, "Warning limit (um)":sgl, "Stop limit (um)":sgl, "Temperature alarm":bool, "Pause 3D-ING":bool, "Low limit (F)":sgl, "High limit (F)":sgl, "Temp limit auto":bool, "Delta (F)":sgl, "Gradient limit (F/min)":sgl, "SW error warning":bool, "Focus index warning":bool, "Focus index low limit":sgl, "Focus index stop limit":sgl, "Run Auto Stig":bool, "FI low limit auto":bool, "FI stop limit auto":bool}
  T27 = cluster{"[0]":bool, "[1]":bool, "[2]":bool, "[3]":bool, "[4]":bool, "[5]":bool, "[6]":bool, "[7]":bool, "[8]":bool, "[9]":bool, "[10]":bool, "[11]":bool, "[12]":bool, "[13]":bool, "[14]":bool, "[15]":bool, "[16]":bool, "[17]":bool, "[18]":bool, "[19]":bool, "[20]":bool, "[21]":bool}
  T28 = cluster{"X resolution":u32, "Z resolution":u32, "X offset (um)":sgl, "Z offset (um)":sgl, "X center (um)":sgl, "Z center (um)":sgl, "X size (um)":sgl, "Z size (um)":sgl, "UL-Ang":sgl, "UR-Ang":sgl, "Line milling time (s)":sgl, "Z-step (nm)":dbl, "Lines auto pause":u16, "Auto pause":bool, "Mill from Bottom":bool, "FIB FOV (um)":sgl, "Auto Profile":bool, "Mill start from Last":bool, "FIB PID on":bool, "FIB PID reset":bool, "FIB PID measured":u8, "FIB PID target":sgl, "FIB PID target slope":sgl, "FIB PID P":sgl, "FIB PID I":sgl, "FIB PID D":sgl, "Emission (uA)":dbl, "Suppressor (V)":sgl, "Auto reheat":bool}
  T29 = cluster{"3D imaging paused alarm":bool, "FIB emission limit warning":bool, "Low limit":sgl, "High limit":sgl, "Specimen @ SEM alarm":bool, "FIB CL current alarm":bool, "Beam Dump 1 alarm":bool, "Milling Z voltage alarm":bool, "EHT off alarm":bool, "Detector over scale warning":bool, "Image clipping alarm":bool, "Warning limit (um)":sgl, "Stop limit (um)":sgl, "Temperature alarm":bool, "Pause 3D-ING":bool, "Low limit (F)":sgl, "High limit (F)":sgl, "Temp limit auto":bool, "Delta (F)":sgl, "Gradient limit (F/min)":sgl, "SW error warning":bool, "Focus index warning":bool, "Focus index low limit":sgl, "Focus index stop limit":sgl, "Run Auto Stig":bool, "FI low limit auto":bool, "FI stop limit auto":bool}
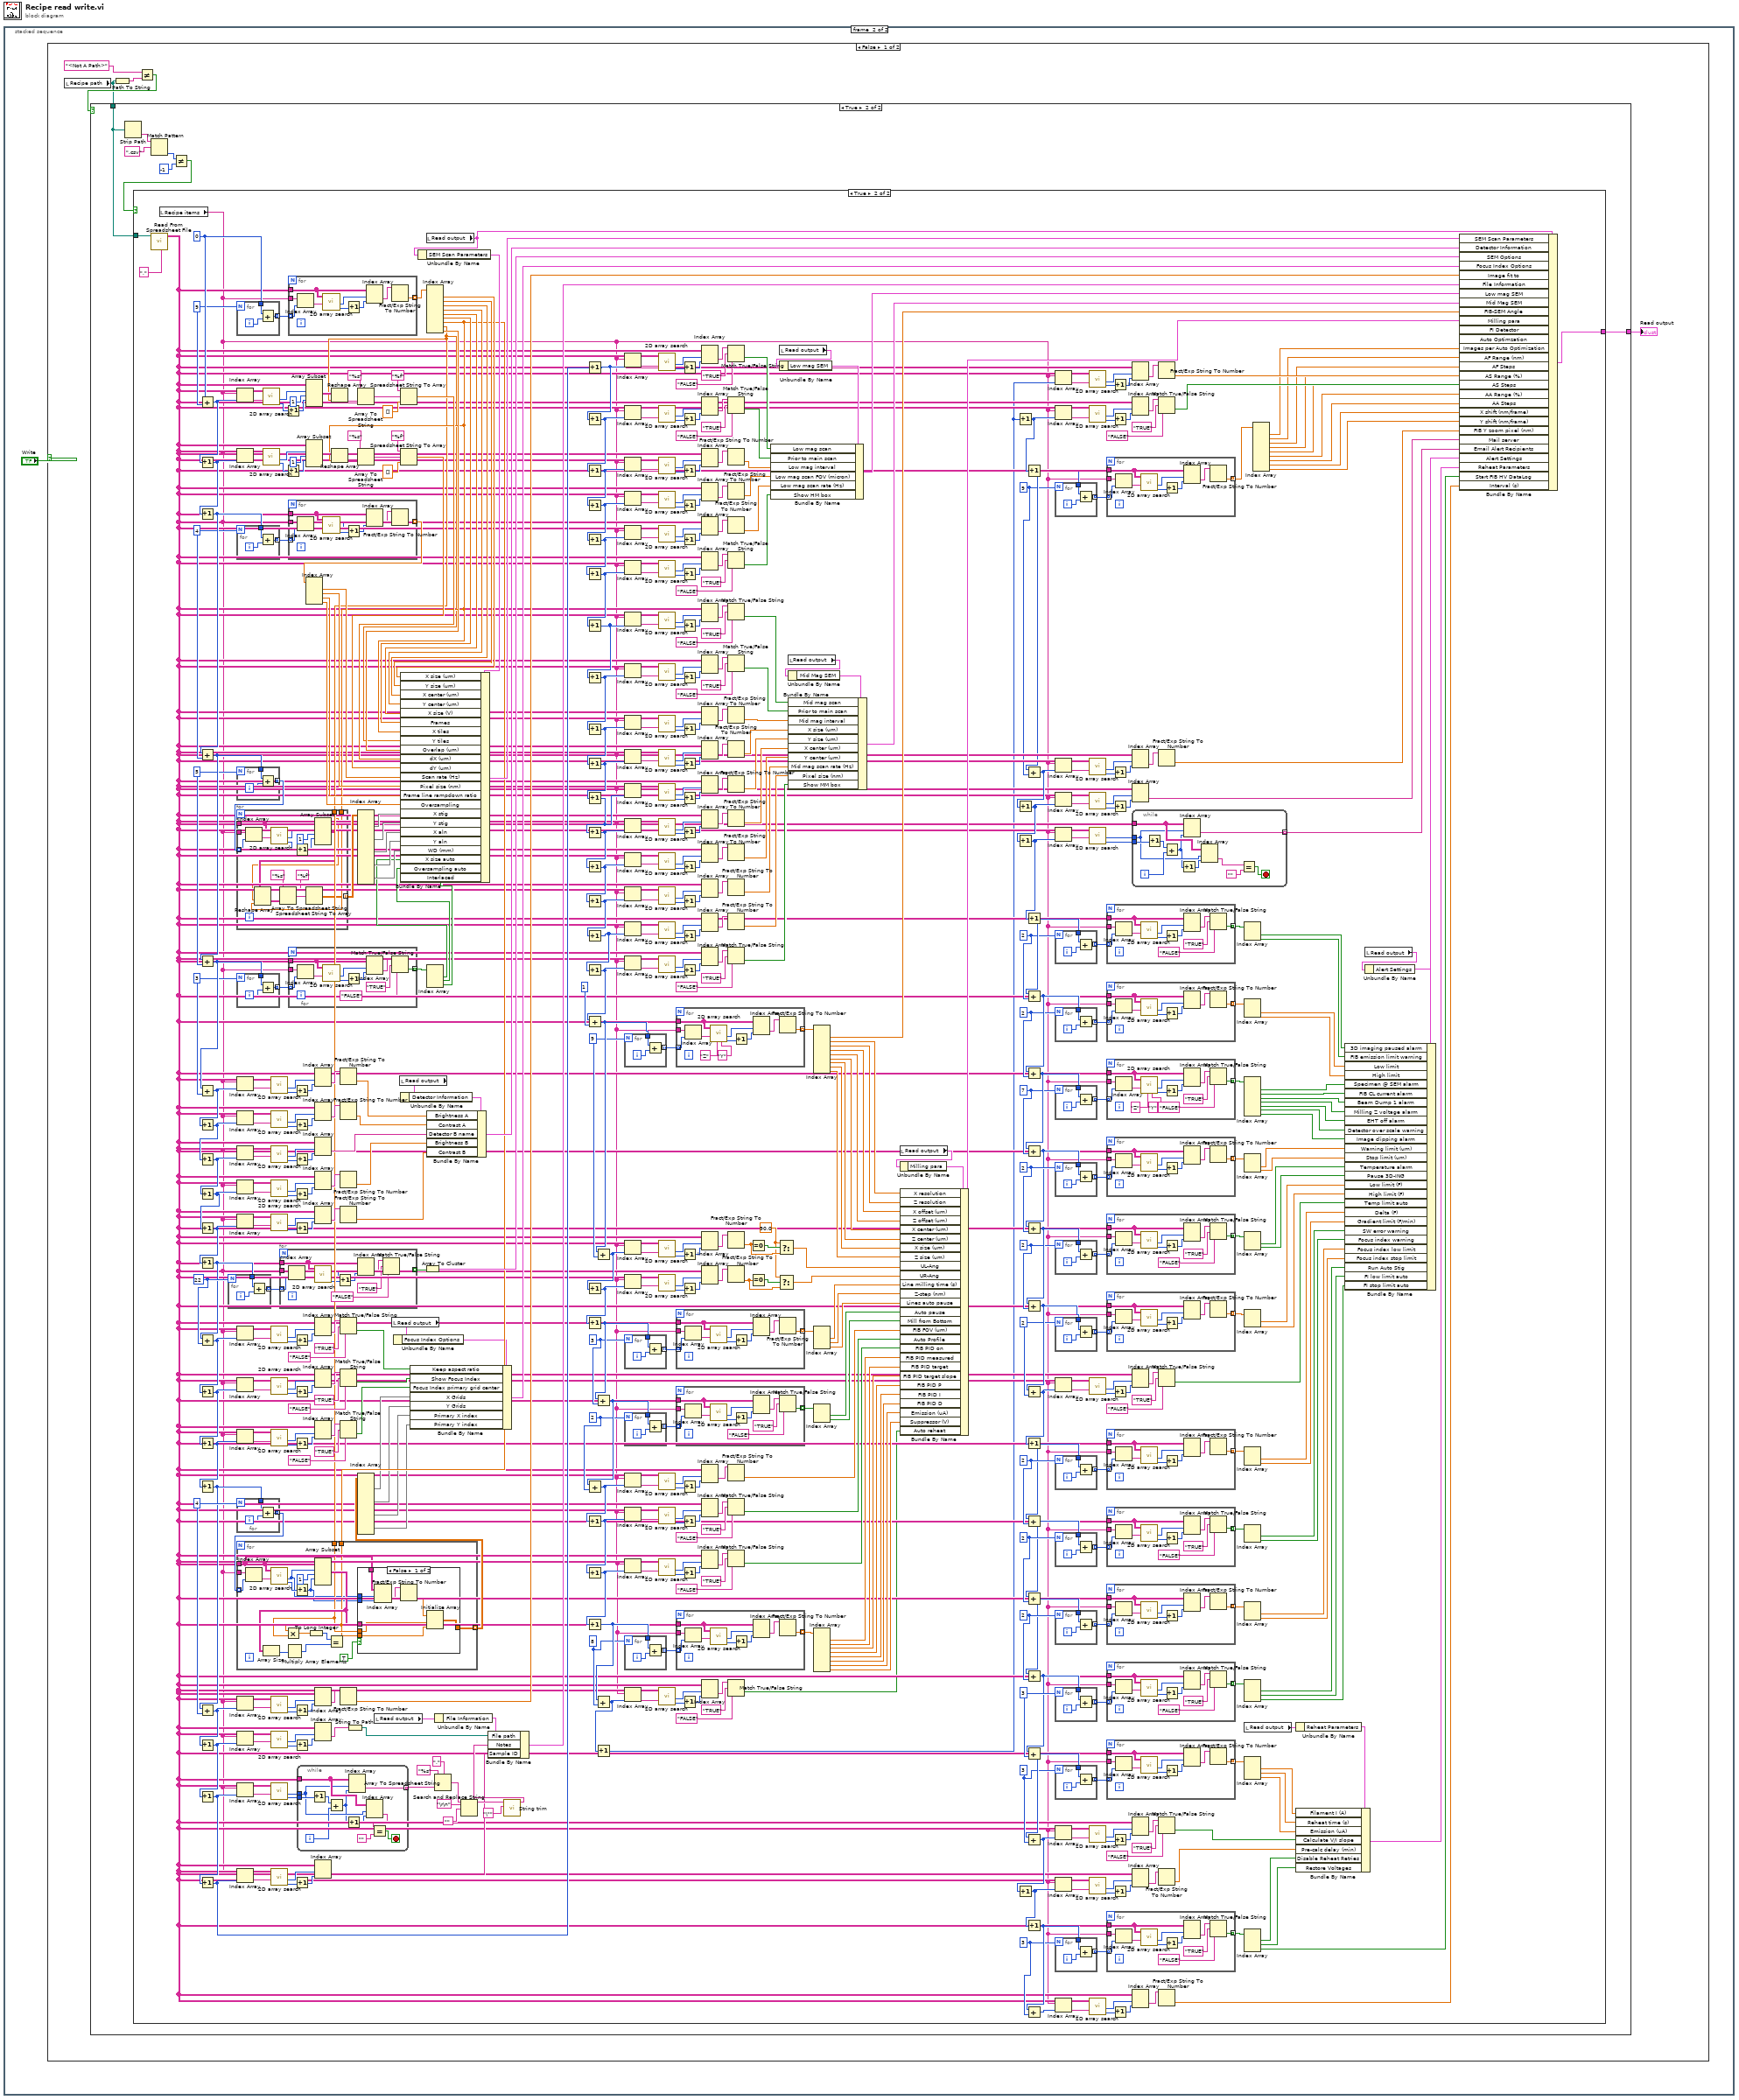
[diagram p0: block diagram]
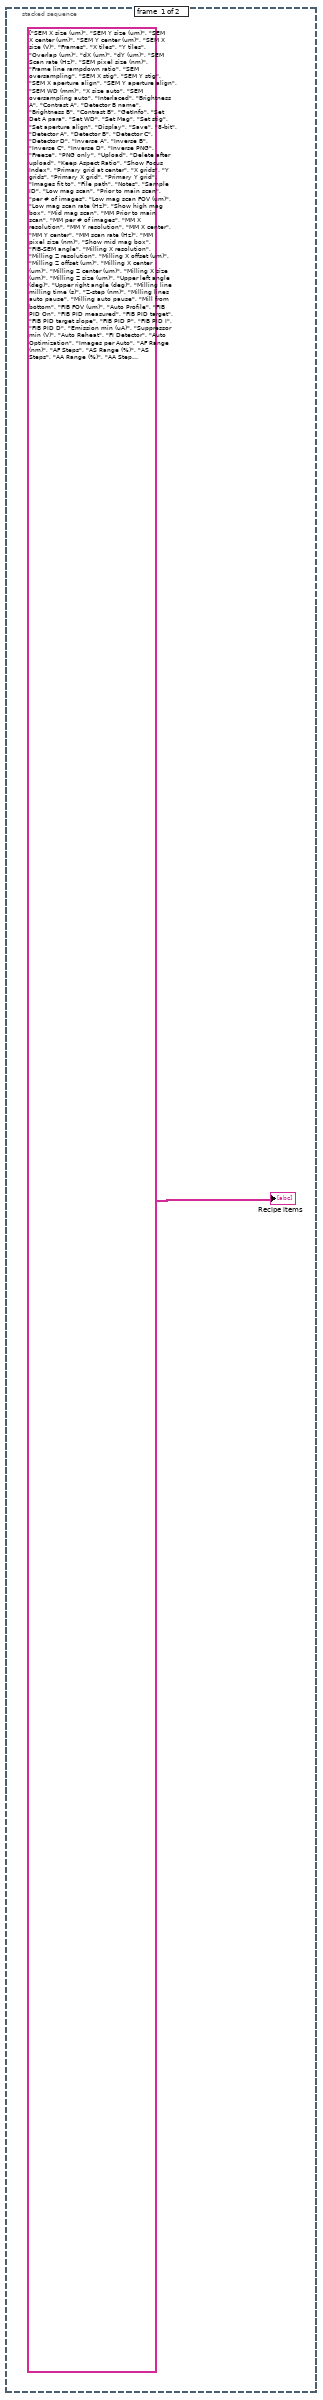
[diagram p2: hidden frame]
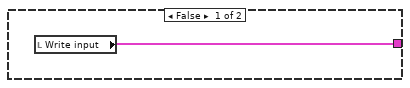
[diagram p3: hidden frame]
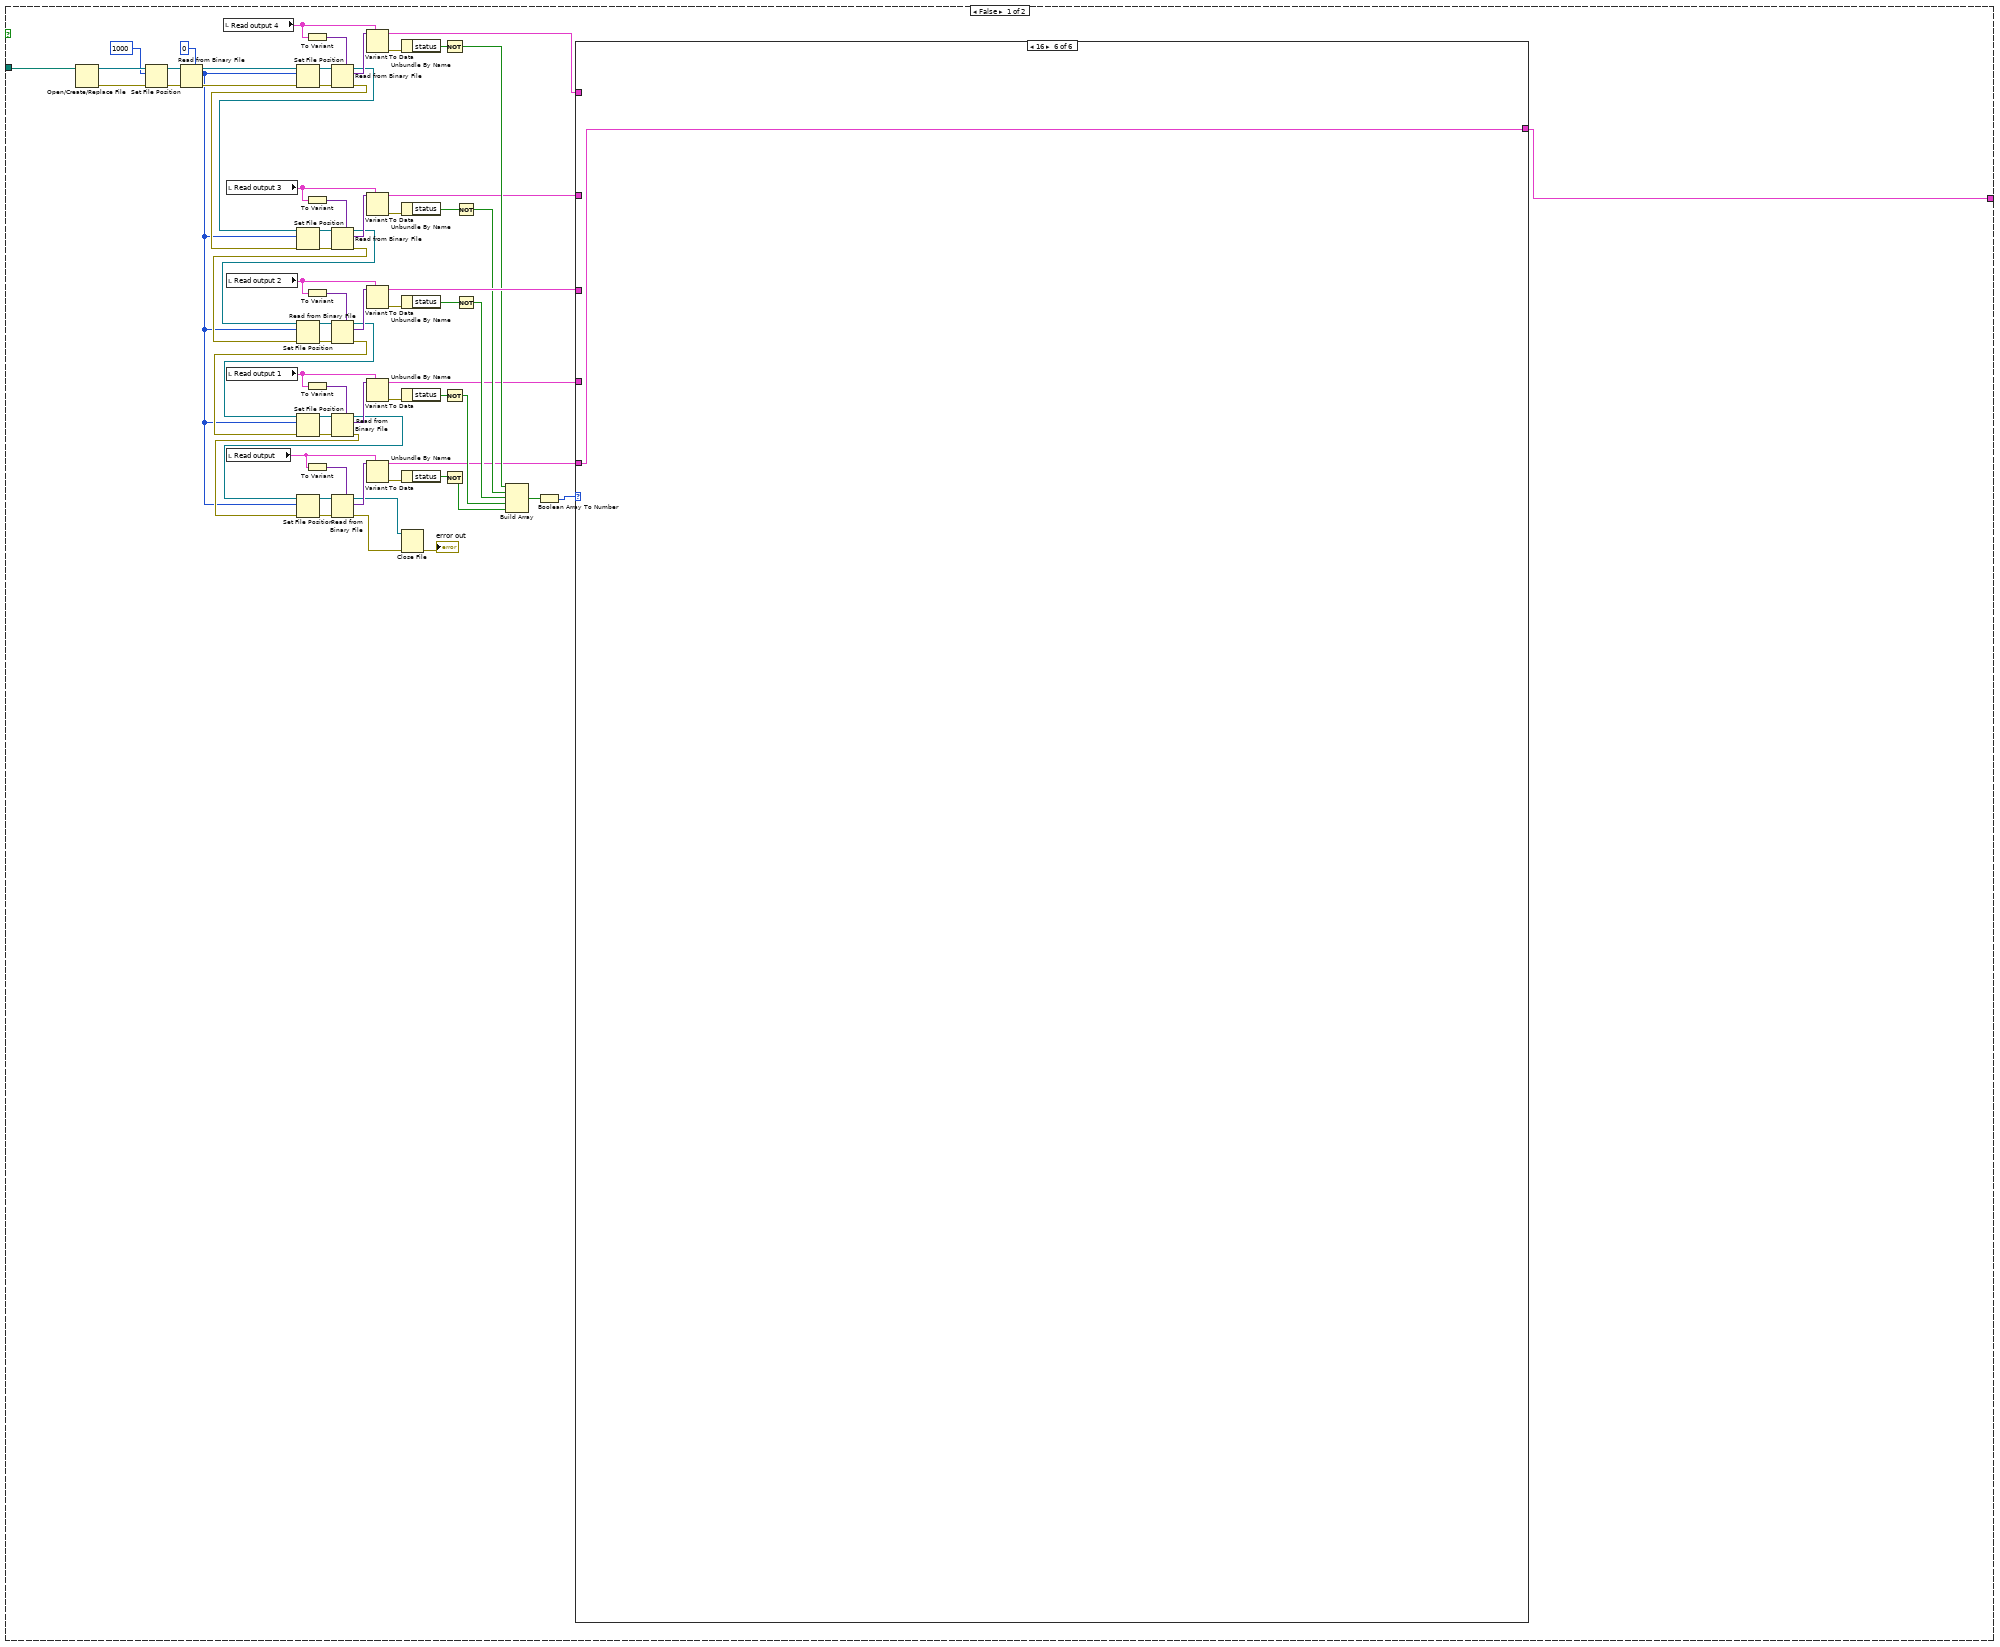
[diagram p4: hidden frame]
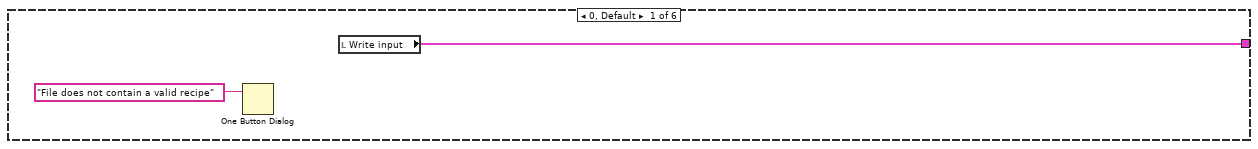
[diagram p5: hidden frame]
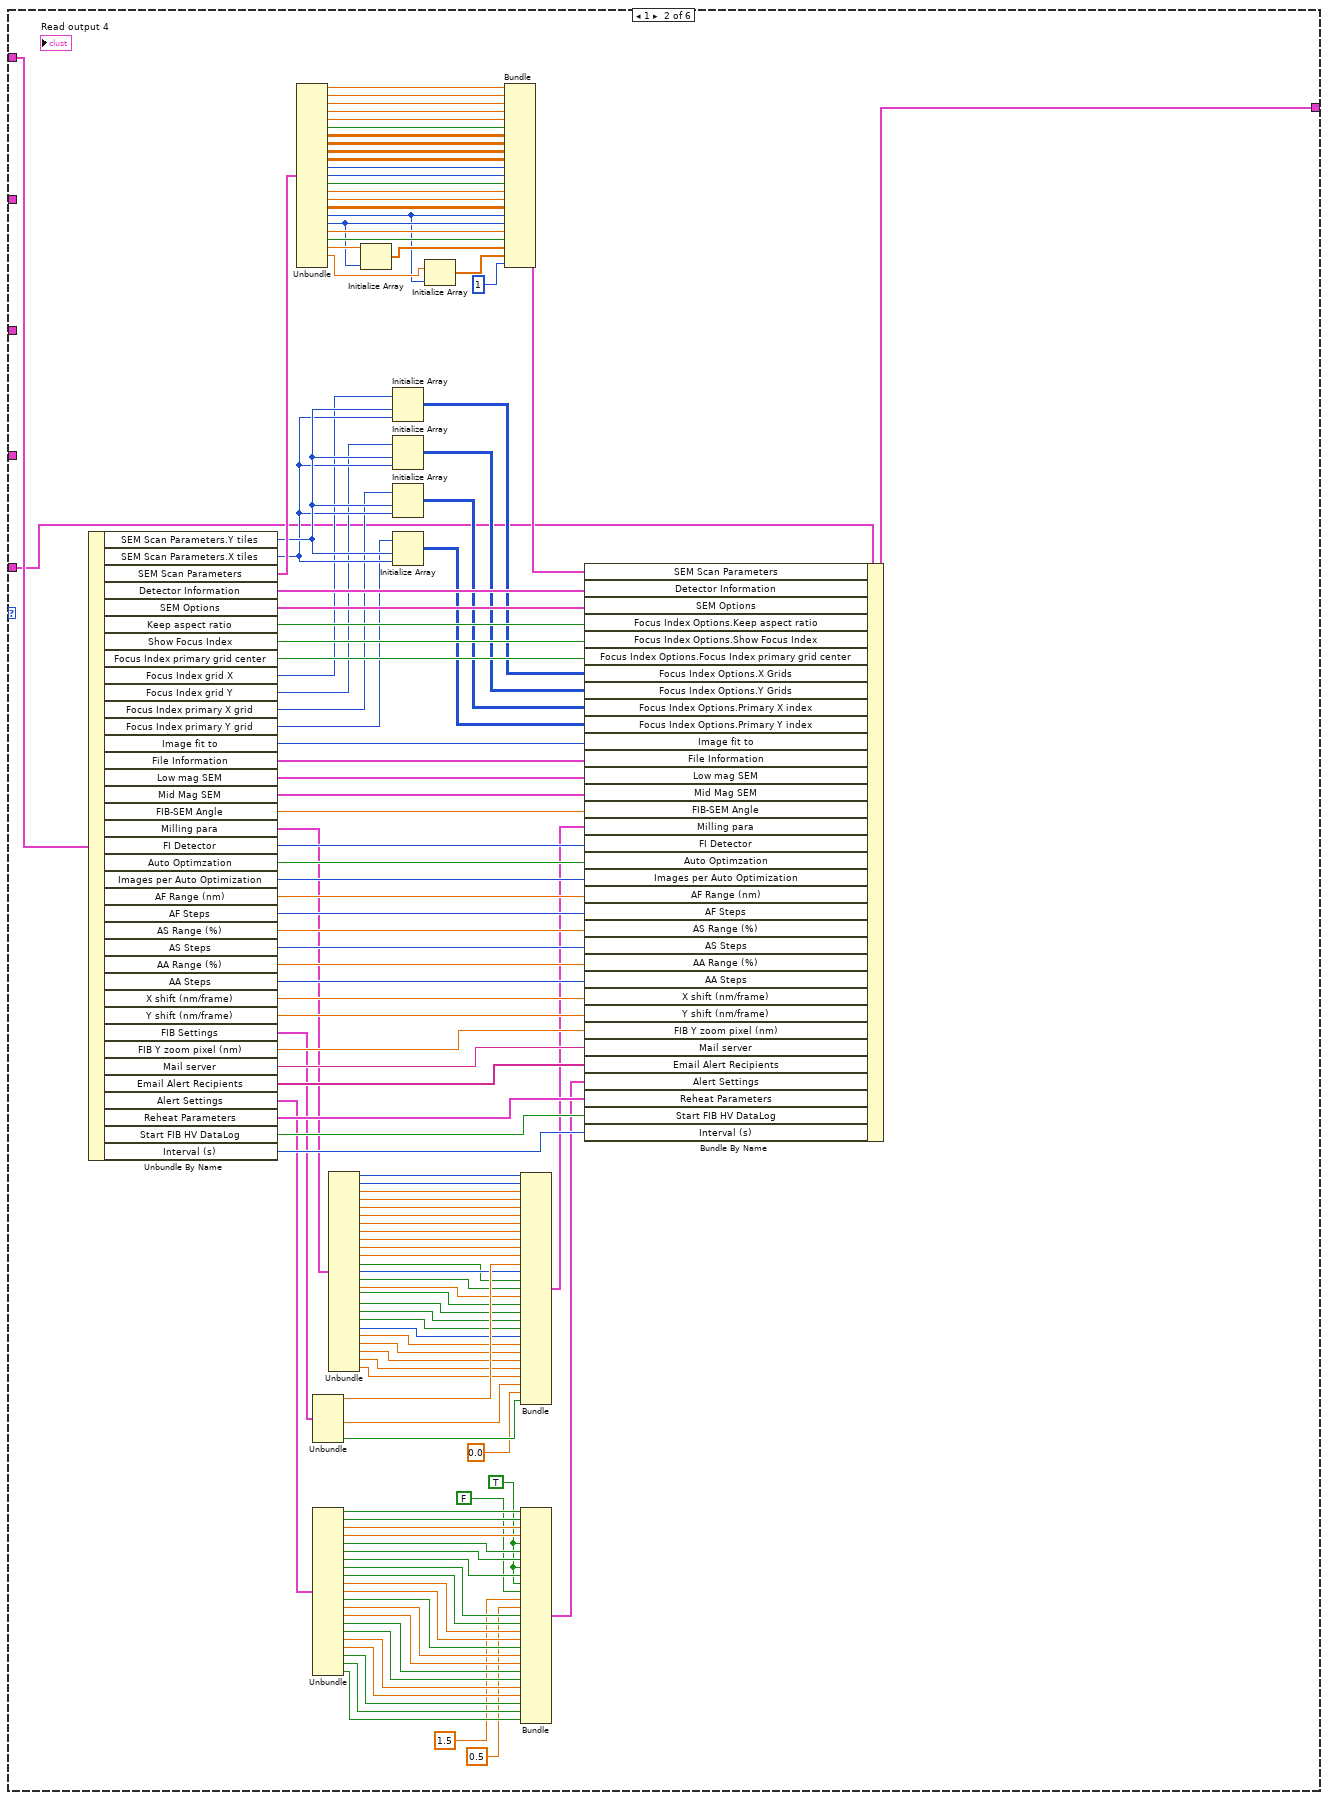
[diagram p6: hidden frame]
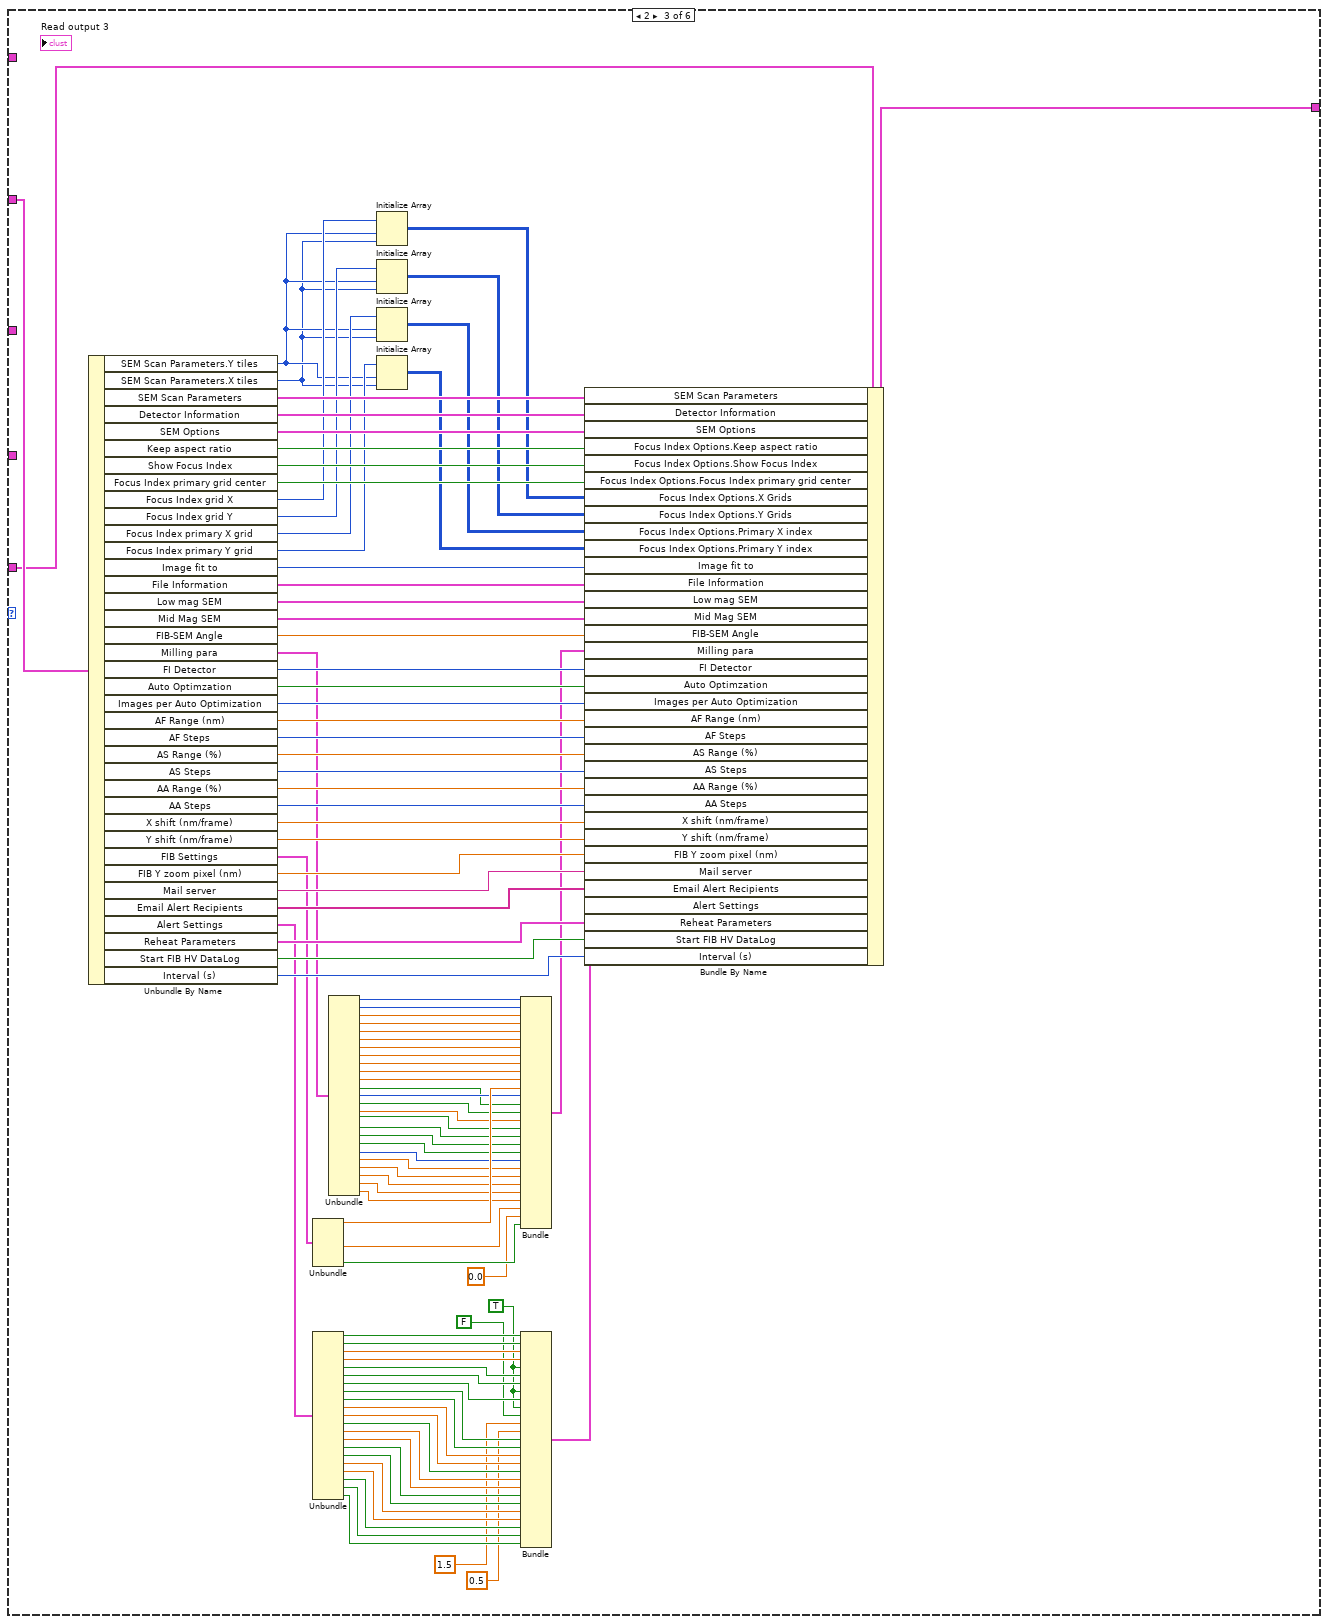
[diagram p7: hidden frame]
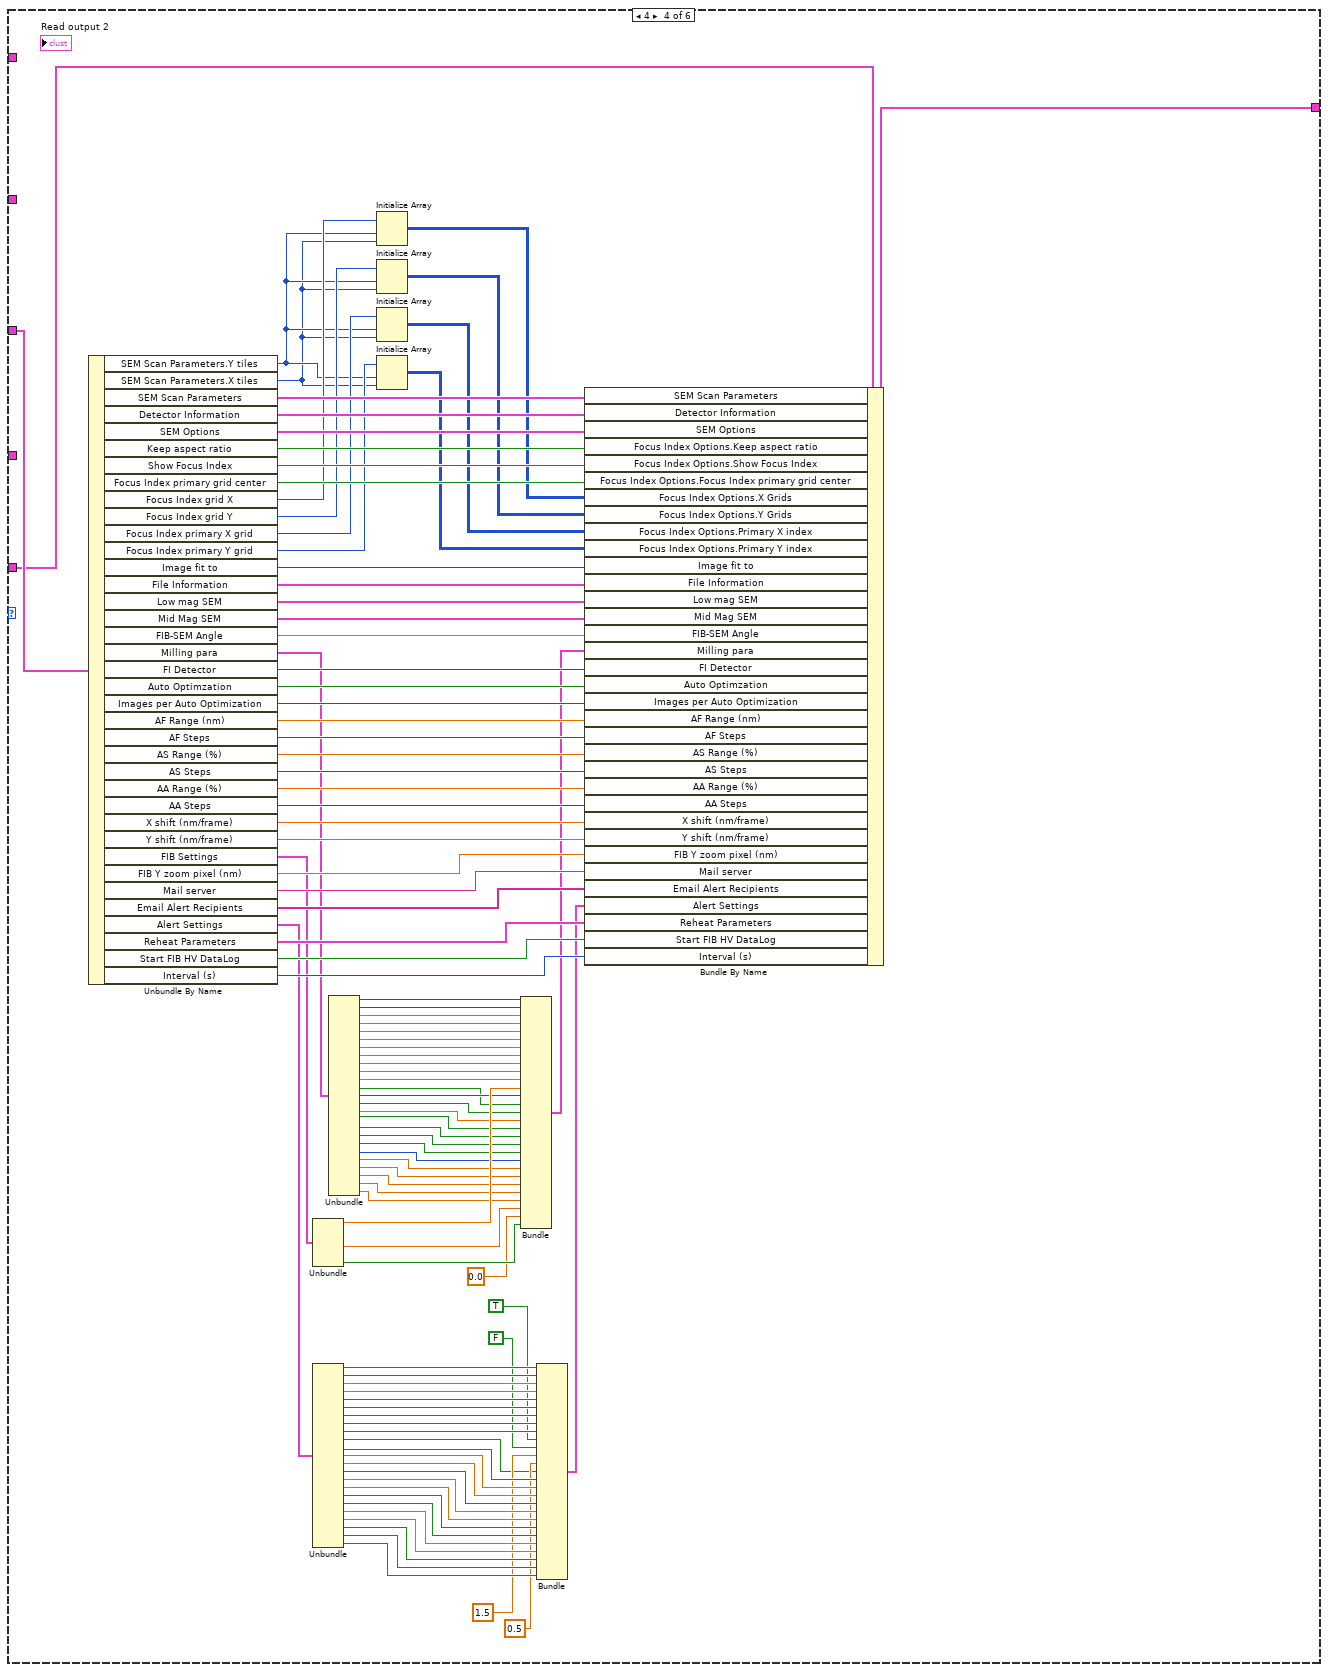
[diagram p8: hidden frame]
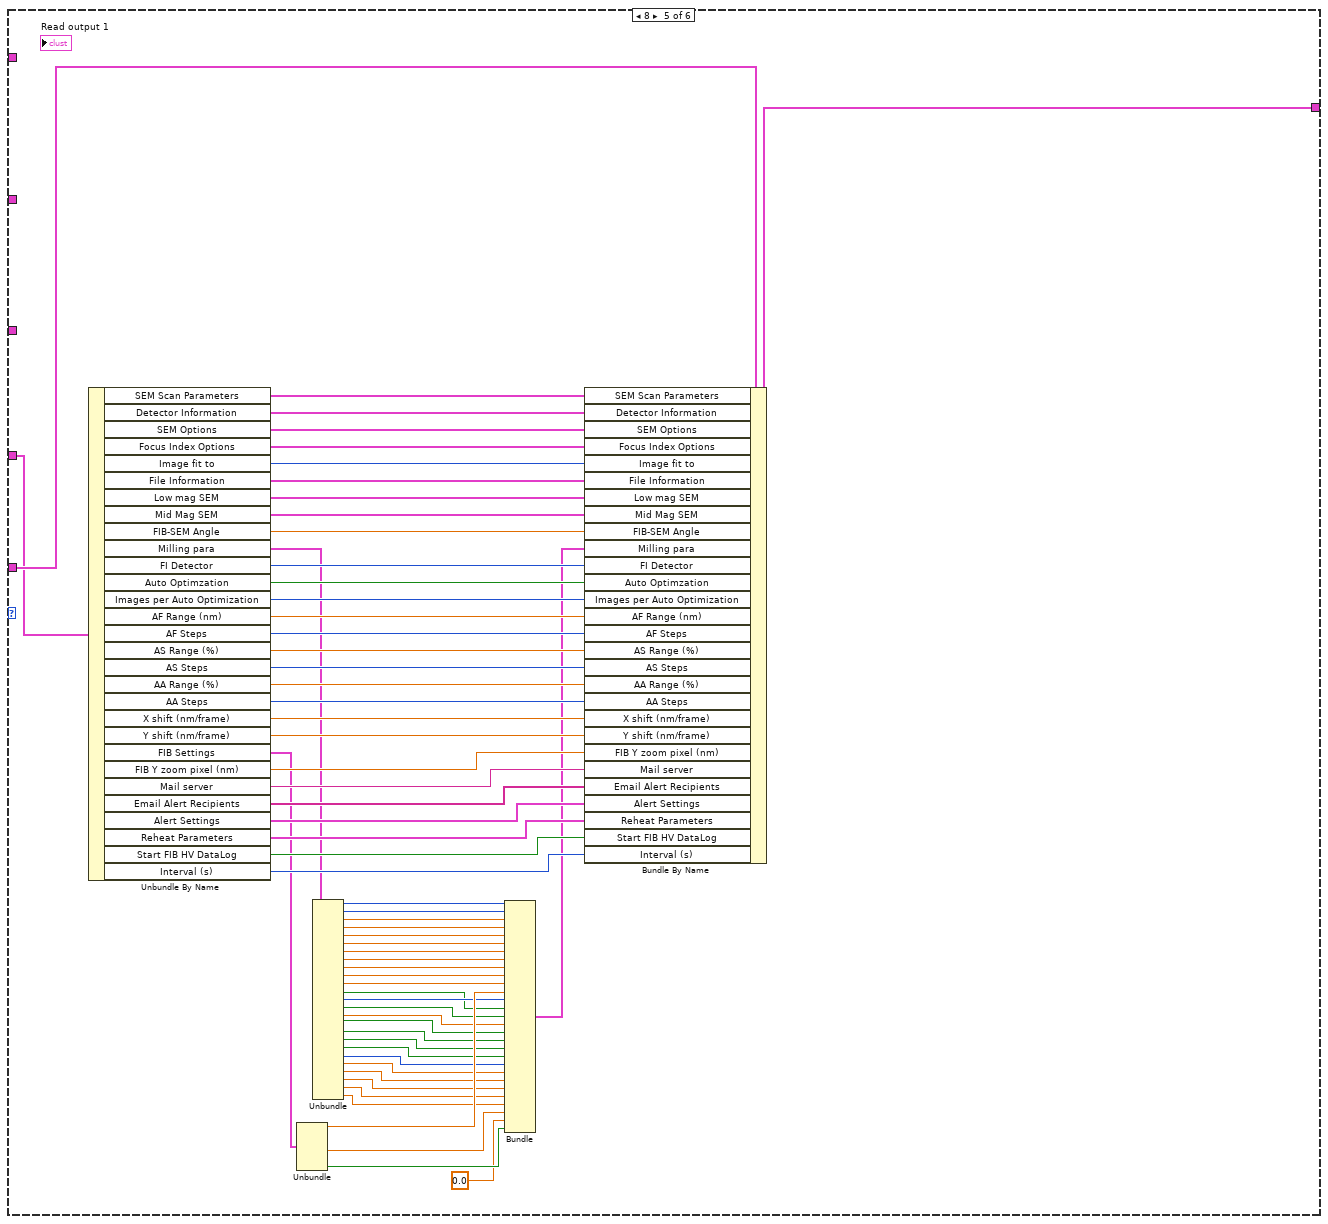
[diagram p9: hidden frame]
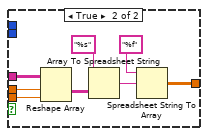
[diagram p10: hidden frame]
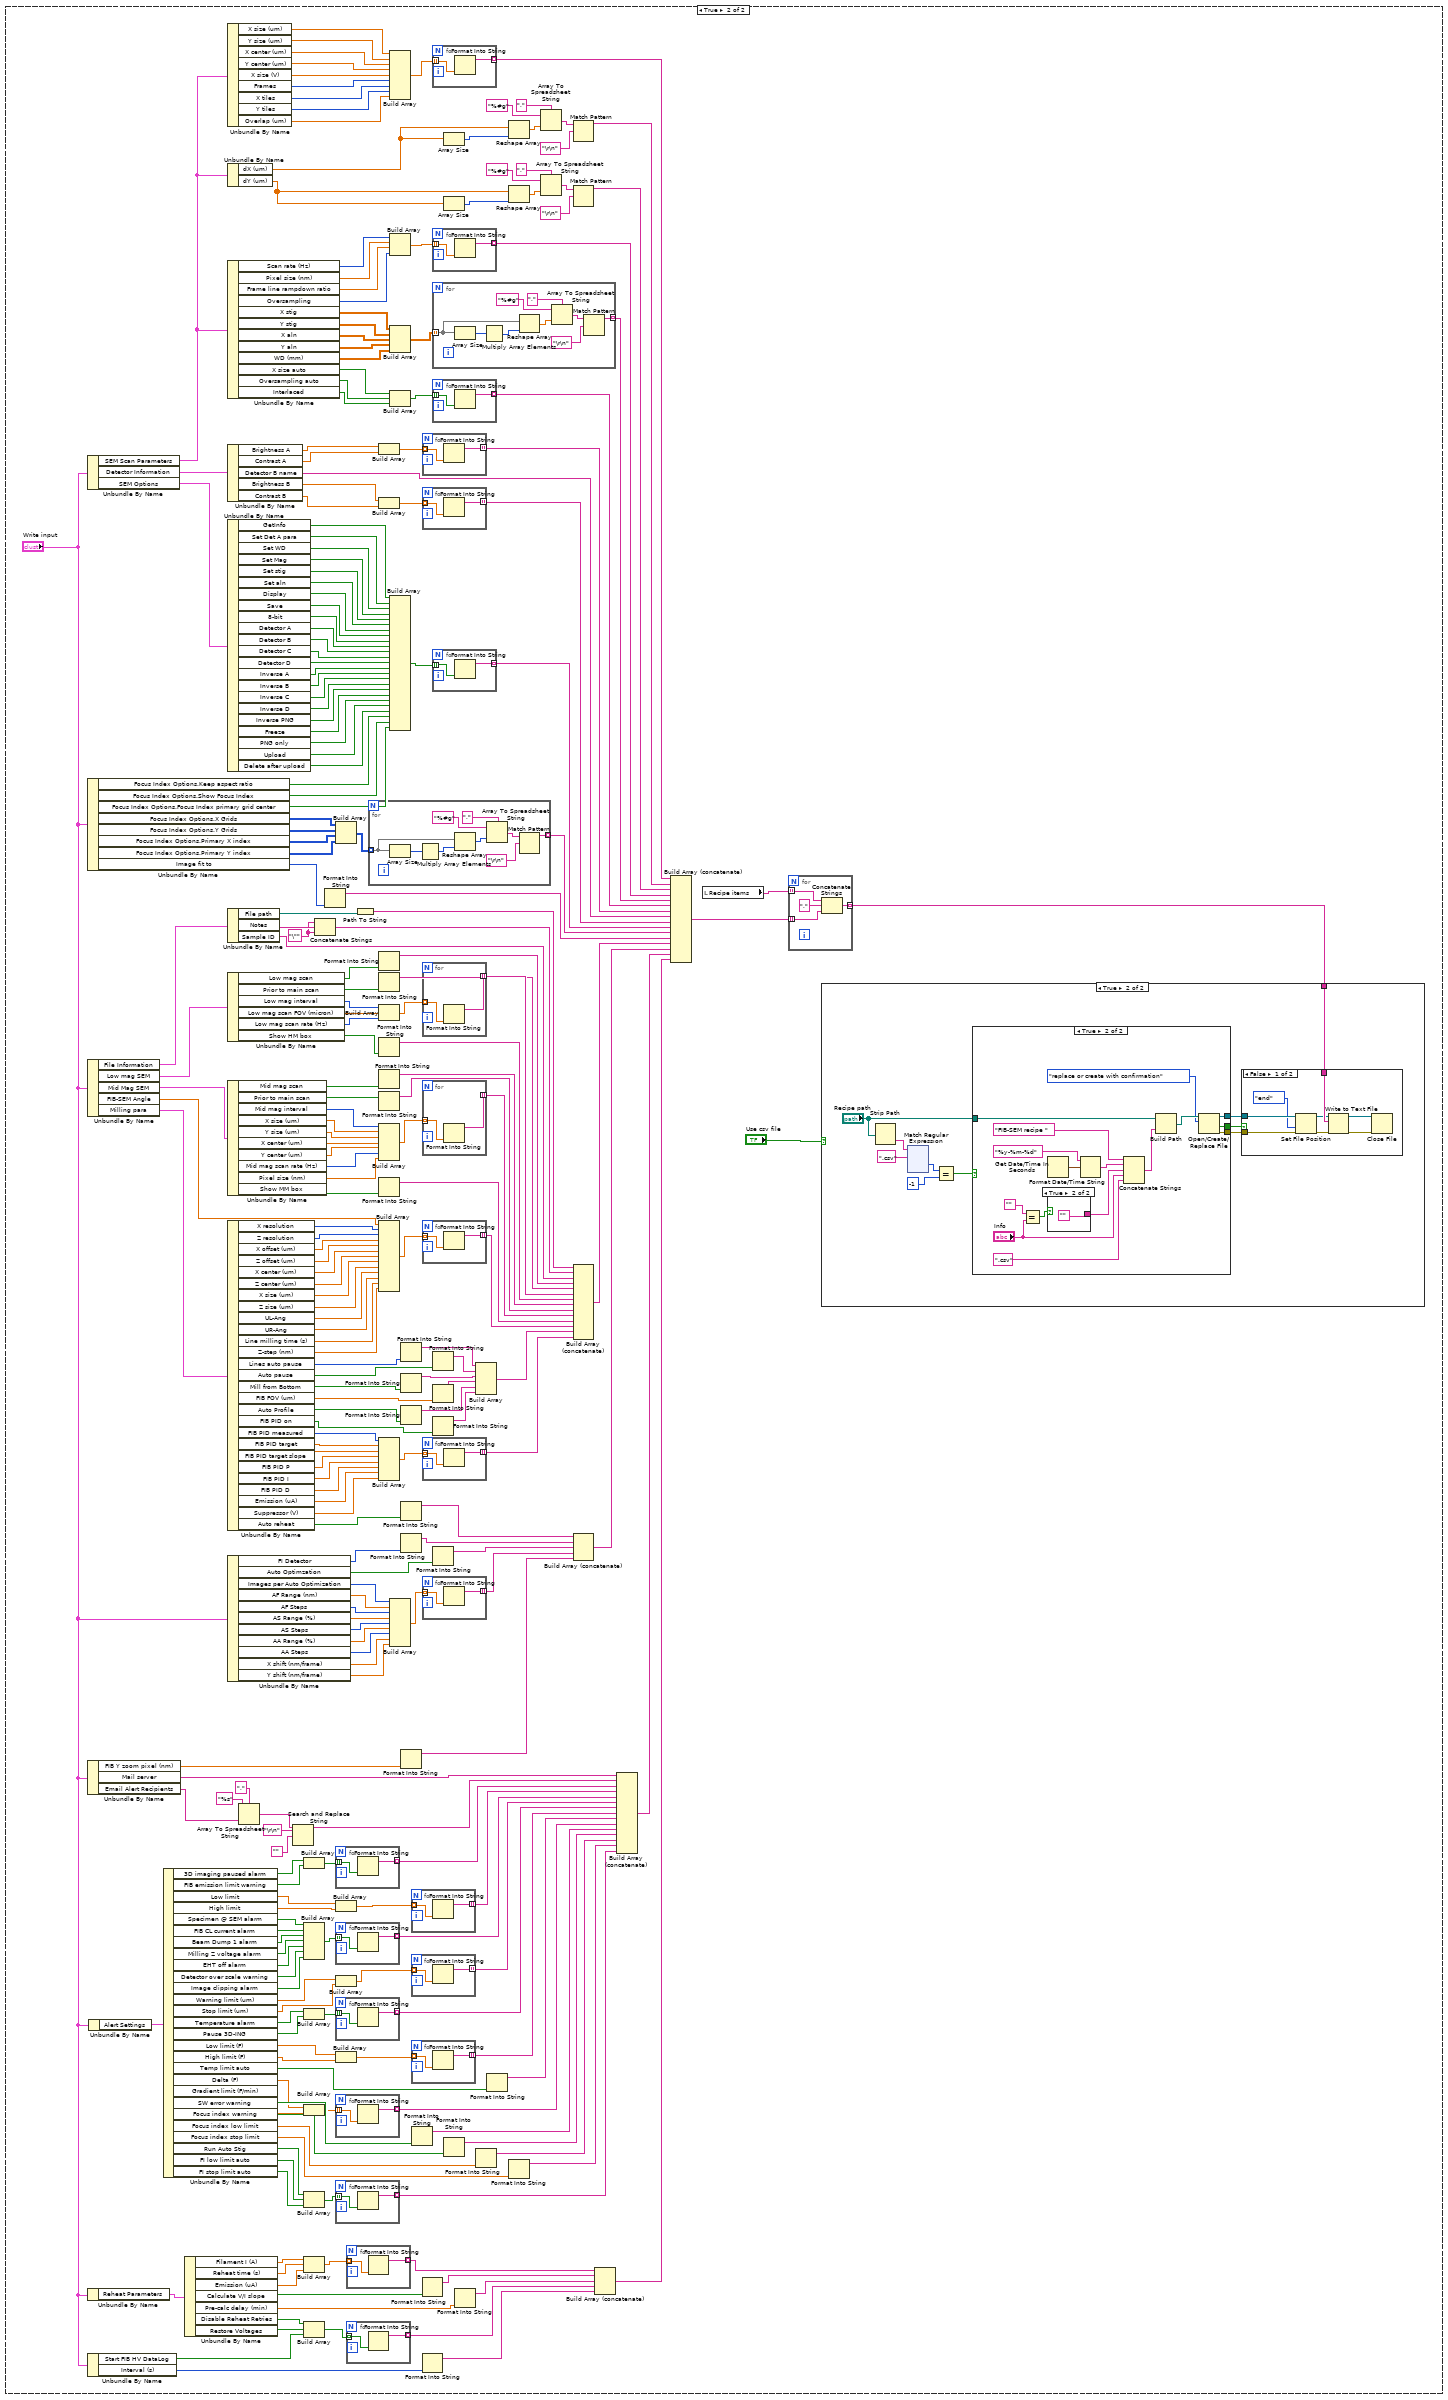
[diagram p11: hidden frame]
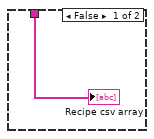
[diagram p12: hidden frame]
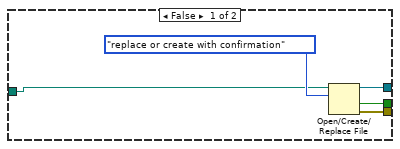
[diagram p13: hidden frame]
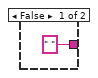
[diagram p14: hidden frame]
diagram:
  n1 = stacked-sequence {
    frame #0 {
      "Recipe items" <- string[] ["SEM X size (um)", "SEM Y size (um)", "SEM X center (um)", "SEM Y center (um)", "SEM X size (V)", "Frames", "X tiles", "Y tiles", "Overlap (um)", "dX (um)", "dY (um)", "SEM Scan rate (Hz)", "SEM pixel size (nm)", "Frame line rampdown ratio", "SEM oversampling", "SEM X stig", "SEM Y stig", "SEM X aperture align", "SEM Y aperture align", "SEM WD (mm)", "X size auto", "SEM oversampling auto", "Interlaced", "Brightness A", "Contrast A", "Detector B name", "Brightness B", "Contrast B", "GetInfo", "Set Det A para", "Set WD", "Set Mag", "Set stig", "Set aperture align", "Display", "Save", "8-bit", "Detector A", "Detector B", "Detector C", "Detector D", "Inverse A", "Inverse B", "Inverse C", "Inverse D", "Inverse PNG", "Freeze", "PNG only", "Upload", "Delete after upload", "Keep Aspect Ratio", "Show Focus Index", "Primary grid at center", "X grids", "Y grids", "Primary X grid", "Primary Y grid", "Images fit to", "File path", "Notes", "Sample ID", "Low mag scan", "Prior to main scan", "per # of images", "Low mag scan FOV (um)", "Low mag scan rate (Hz)", "Show high mag box", "Mid mag scan", "MM Prior to main scan", "MM per # of images", "MM X resolution", "MM Y resolution", "MM X center", "MM Y center", "MM scan rate (Hz)", "MM pixel size (nm)", "Show mid mag box", "FIB-SEM angle", "Milling X resolution", "Milling Z resolution", "Milling X offset (um)", "Milling Z offset (um)", "Milling X center (um)", "Milling Z center (um)", "Milling X size (um)", "Milling Z size (um)", "Upper left angle (deg)", "Upper right angle (deg)", "Milling line milling time (s)", "Z-step (nm)", "Milling lines auto pause", "Milling auto pause", "Mill from bottom", "FIB FOV (um)", "Auto Profile", "FIB PID On", "FIB PID measured", "FIB PID target", "FIB PID target slope", "FIB PID P", "FIB PID I", "FIB PID D", "Emission min (uA)", "Suppressor min (V)", "Auto Reheat", "FI Detector", "Auto Optimization", "Images per Auto", "AF Range (nm)", "AF Steps", "AS Range (%)", "AS Steps", "AA Range (%)", "AA Steps", "X shift (nm/frame)", "Y shift (nm/frame)", "FIB Z zoom pixel (nm)", "Mail server", "Email alert recipients", "3D imaging pause alarm", "FIB emission limit warning", "Low limit", "High limit", "Specimen @ SEM alarm", "FIB CL current alarm", "Beam Dump 1 alarm", "Milling Z voltage alarm", "EHT off alarm", "Detector over scale warning", "Image clipping alarm", "Warning limit (um)", "Stop limit (um)", "Temperature alarm", "Pause 3D-ING", "Low limit (F)", "High limit (F)", "Temp limit auto", "Temperature range (F)", "Gradient limit (F/min)", "SW error warning", "Focus index warning", "Focus index low limit", "Focus index stop limit", "Run Auto Stig", "FI low limit auto", "FI stop limit auto", "FIB reheat filament I (uA)", "FIB reheat time (s)", "FIB emission target (uA)", "Calculate V/I slope", "Pre-calc delay (min)", "Disable reheat retries", "Restore voltages", "Start FIB HV Datalog", "FIB HV Datalog interval (s)"] ("appended array")
    }
    frame #1 {
      n2 = case shown="False" "Write" {
        frame False {
          n3 = local read "Recipe path"() -> (w4:path)
          n4 = Path To String(path=w4) -> (string=w5:string)
          n5 = Not Equal?(x="<Not A Path>", y=w5) -> (x != y?=w7:bool)
          n6 = case shown="True" w7 {
            tunnel: [w8 w9] -> w3
            tunnel: w4 -> [_ w15]
            frame False {
              n7 = local read "Write input"() -> (w8:T1)
            }
            frame True {
              n8 = Strip Path(path=w15) -> (name=w13:string)  [unwired: 1 out]
              n9 = Match Pattern(string=w13, regular expression=".csv") -> (offset past match=w12:i32)  [unwired: 1 in, 3 out]
              n10 = Not Equal?(x=w12, y=-1) -> (x != y?=w10:bool)
              n11 = case shown="True" w10 {
                tunnel: [w30 w481] -> w9
                tunnel: w15 -> [w78 w742]
                frame False {
                  n12 = Open/Create/Replace File(file path (use dialog)=w78) -> (refnum out=w83:refnum<file>, error out=w84:errorcluster)  [unwired: 5 in, 1 out]
                  n13 = Set File Position(offset (in bytes) (0)=i64 1000, refnum=w83, error in=w84) -> (refnum out=w82:refnum<file>, error out=w81:errorcluster)  [unwired: 1 in]
                  n14 = Read from Binary File(5:i64 0, 8:w81, 11:w82) -> (0:w58:errorcluster, 2:w18:i64, 3:w59:refnum<file>)  [unwired: 3 in, 1 out]
                  n15 = local read "Read output 4"() -> (w57:T4)
                  n16 = local read "Read output 3"() -> (w55:T3)
                  n17 = local read "Read output 2"() -> (w68:T5)
                  n18 = local read "Read output 1"() -> (w41:T2)
                  n19 = local read "Read output"() -> (w23:T1)
                  n20 = Set File Position(offset (in bytes) (0)=w18, refnum=w59, error in=w58) -> (refnum out=w62:refnum<file>, error out=w61:errorcluster)  [unwired: 1 in]
                  n21 = To Variant(anything=w57) -> (Variant=w63:variant)
                  n22 = To Variant(anything=w55) -> (Variant=w51:variant)
                  n23 = To Variant(anything=w68) -> (Variant=w74:variant)
                  n24 = To Variant(anything=w41) -> (Variant=w38:variant)
                  n25 = To Variant(anything=w23) -> (Variant=w27:variant)
                  n26 = Read from Binary File(5:w63, 8:w61, 11:w62) -> (0:w44:errorcluster, 2:w64:variant, 3:w46:refnum<file>)  [unwired: 3 in, 1 out]
                  n27 = Set File Position(offset (in bytes) (0)=w18, refnum=w46, error in=w44) -> (refnum out=w52:refnum<file>, error out=w53:errorcluster)  [unwired: 1 in]
                  n28 = Read from Binary File(5:w51, 8:w53, 11:w52) -> (0:w43:errorcluster, 2:w50:variant, 3:w45:refnum<file>)  [unwired: 3 in, 1 out]
                  n29 = Set File Position(offset (in bytes) (0)=w18, refnum=w45, error in=w43) -> (refnum out=w75:refnum<file>, error out=w76:errorcluster)  [unwired: 1 in]
                  n30 = Read from Binary File(5:w74, 8:w76, 11:w75) -> (0:w33:errorcluster, 2:w73:variant, 3:w34:refnum<file>)  [unwired: 3 in, 1 out]
                  n31 = Set File Position(offset (in bytes) (0)=w18, refnum=w34, error in=w33) -> (refnum out=w37:refnum<file>, error out=w36:errorcluster)  [unwired: 1 in]
                  n32 = Read from Binary File(5:w38, 8:w36, 11:w37) -> (0:w20:errorcluster, 2:w39:variant, 3:w19:refnum<file>)  [unwired: 3 in, 1 out]
                  n33 = Set File Position(offset (in bytes) (0)=w18, refnum=w19, error in=w20) -> (refnum out=w26:refnum<file>, error out=w25:errorcluster)  [unwired: 1 in]
                  n34 = Read from Binary File(5:w27, 8:w25, 11:w26) -> (0:w21:errorcluster, 2:w28:variant, 3:w22:refnum<file>)  [unwired: 3 in, 1 out]
                  n35 = Variant To Data(type=w57, Variant=w64) -> (data=w56:T4, error out=w60:errorcluster)  [unwired: 1 in]
                  n36 = Variant To Data(type=w55, Variant=w50) -> (data=w42:T3, error out=w54:errorcluster)  [unwired: 1 in]
                  n37 = Variant To Data(type=w68, Variant=w73) -> (data=w67:T5, error out=w77:errorcluster)  [unwired: 1 in]
                  n38 = Variant To Data(type=w41, Variant=w39) -> (data=w31:T2, error out=w35:errorcluster)  [unwired: 1 in]
                  n39 = Variant To Data(type=w23, Variant=w28) -> (data=w16:T1, error out=w24:errorcluster)  [unwired: 1 in]
                  n40 = Unbundle By Name(w60) -> ("status"=w65:bool)
                  n41 = Unbundle By Name(w54) -> ("status"=w49:bool)
                  n42 = Unbundle By Name(w77) -> ("status"=w72:bool)
                  n43 = Unbundle By Name(w35) -> ("status"=w40:bool)
                  n44 = Unbundle By Name(w24) -> ("status"=w29:bool)
                  n45 = Close File(refnum=w22, error in=w21) -> (error out=→"error out":errorcluster)  [unwired: 1 out]
                  n46 = Not(x=w65) -> (.not. x?=w47:bool)
                  n47 = Not(x=w40) -> (.not. x?=w32:bool)
                  n48 = Not(x=w29) -> (.not. x?=w17:bool)
                  n49 = Not(x=w49) -> (.not. x?=w48:bool)
                  n50 = Not(x=w72) -> (.not. x?=w66:bool)
                  n51 = Build Array(w47, w48, w66, w32, w17) -> (w71:bool[])
                  n52 = Boolean Array To Number(Boolean array=w71) -> (number=w70:u32)
                  n53 = case shown="16" w70 {
                    tunnel: w67 -> [_ _ _ w356 _ _]
                    tunnel: [w85 w88 w214 w345 w449 w477] -> w30
                    tunnel: w56 -> [_ w158 _ _ _ _]
                    tunnel: w42 -> [_ _ w284 _ _ _]
                    tunnel: w31 -> [_ _ _ _ w448 _]
                    tunnel: w16 -> [_ w120 w246 w346 w450 w477]
                    frame 0, Default {
                      n54 = One Button Dialog(message="File does not contain a valid recipe") -> ()  [unwired: 1 in, 1 out]
                      n55 = local read "Write input"() -> (w85:T1)
                    }
                    frame 1 {
                      w126 = TRUE ("Pause 3D-ING")
                      n56 = Unbundle By Name(w158) -> ("SEM Scan Parameters.Y tiles"=w157:u8, "SEM Scan Parameters.X tiles"=w156:u8, "SEM Scan Parameters"=w166:T7, "Detector Information"=w186:T8, "SEM Options"=w187:T9, "Keep aspect ratio"=w188:bool, "Show Focus Index"=w189:bool, "Focus Index primary grid center"=w190:bool, "Focus Index grid X"=w155:u8, "Focus Index grid Y"=w154:u8, "Focus Index primary X grid"=w153:u8, "Focus Index primary Y grid"=w152:u8, "Image fit to"=w191:u8, "File Information"=w192:T10, "Low mag SEM"=w193:T11, "Mid Mag SEM"=w194:T12, "FIB-SEM Angle"=w195:dbl, "Milling para"=w90:T13, "FI Detector"=w196:u16, "Auto Optimzation"=w197:bool, "Images per Auto Optimization"=w198:u16, "AF Range (nm)"=w199:sgl, "AF Steps"=w200:u8, "AS Range (%)"=w201:sgl, "AS Steps"=w202:u8, "AA Range (%)"=w203:sgl, "AA Steps"=w204:u8, "X shift (nm/frame)"=w205:dbl, "Y shift (nm/frame)"=w206:dbl, "FIB Settings"=w91:T14, "FIB Y zoom pixel (nm)"=w207:dbl, "Mail server"=w208:string, "Email Alert Recipients"=w209:string[], "Alert Settings"=w122:T15, "Reheat Parameters"=w210:T16, "Start FIB HV DataLog"=w211:bool, "Interval (s)"=w212:u16)
                      n57 = Unbundle(w166) -> ("X size (um)"=w185:sgl, "Y size (um)"=w184:sgl, "X center (um)"=w183:dbl, "Y center (um)"=w182:dbl, "X size (V)"=w180:dbl, "X size auto"=w181:bool, "X stig"=w179:sgl[][], "Y stig"=w178:sgl[][], "X aln"=w177:sgl[][], "Y aln"=w176:sgl[][], "Scan rate (Hz)"=w175:u32, "Oversampling"=w174:u32, "Oversampling auto"=w173:bool, "Frame line rampdown ratio"=w172:sgl, "Pixel size (nm)"=w171:sgl, "WD (mm)"=w170:sgl[][], "X tiles"=w161:u8, "Y tiles"=w164:u8, "Overlap (um)"=w167:sgl, "Interlaced"=w168:bool, "dX (um)"=w165:sgl, "dY (um)"=w162:sgl)  [unwired: 1 out]
                      n58 = Unbundle(w91) -> ("Z-step (nm)"=w108:dbl, "Emission min"=w96:dbl, "Auto reheat"=w92:bool)  [unwired: 3 out]
                      n59 = Unbundle(w122) -> ("3D imaging paused alarm"=w147:bool, "FIB emission limit warning"=w146:bool, "Low limit"=w145:dbl, "High limit"=w144:dbl, "Specimen current alarm"=w142:bool, "Beam dump alarm"=w141:bool, "EHT off alarm"=w138:bool, "Temperature alarm"=w139:bool, "Pause 3D-ING"=w140:bool, "Low limit (F)"=w143:sgl, "High limit (F)"=w137:sgl, "Temp limit auto"=w136:bool, "Delta (F)"=w135:sgl, "Gradient limit (F/min)"=w134:sgl, "SW error warning"=w133:bool, "Focus index warning"=w132:bool, "Focus index low limit"=w131:dbl, "Focus index stop limit"=w130:sgl, "Run Auto Stig"=w129:bool, "FI low limit auto"=w128:bool, "FI stop limit auto"=w127:bool)
                      n60 = Unbundle(w90) -> ("X resolution"=w119:u32, "Y resolution"=w118:u32, "X offset (um)"=w117:sgl, "Y offset (um)"=w116:sgl, "X center (um)"=w115:sgl, "Y center (um)"=w114:sgl, "X size (um)"=w113:sgl, "Y size (um)"=w112:sgl, "UL-Ang"=w111:sgl, "UR-Ang"=w110:sgl, "Line milling time (s)"=w109:sgl, "Auto pause"=w106:bool, "Lines auto pause"=w107:u16, "Mill from Bottom"=w105:bool, "FIB FOV (um)"=w104:sgl, "SEM on"=w103:bool, "Mill start from Last"=w95:bool, "FIB PID on"=w94:bool, "FIB PID reset"=w93:bool, "FIB PID measured"=w102:u8, "FIB PID target"=w101:sgl, "FIB PID target slope"=w100:sgl, "FIB PID P"=w99:sgl, "FIB PID I"=w98:sgl, "FIB PID D"=w97:sgl)
                      n61 = Initialize Array(w165, w164) -> (w163:sgl[])
                      n62 = Initialize Array(w155, w157, w156) -> (w151:u8[][])
                      n63 = Initialize Array(w154, w157, w156) -> (w150:u8[][])
                      n64 = Initialize Array(w153, w157, w156) -> (w149:u8[][])
                      n65 = Initialize Array(w152, w157, w156) -> (w148:u8[][])
                      n66 = Initialize Array(w162, w161) -> (w160:sgl[])
                      n67 = Bundle("X size (um)"=w185, "Y size (um)"=w184, "X center (um)"=w183, "Y center (um)"=w182, "X size (V)"=w180, "X size auto"=w181, "X stig"=w179, "Y stig"=w178, "X aln"=w177, "Y aln"=w176, "Scan rate (Hz)"=w175, "Oversampling"=w174, "Oversampling auto"=w173, "Frame line rampdown ratio"=w172, "Pixel size (nm)"=w171, "WD (mm)"=w170, "X tiles"=w161, "Y tiles"=w164, "Overlap (um)"=w167, "Interlaced"=w168, w163, w160, "X tiles"=u8 1) -> (w159:T17)  [unwired: 1 in]
                      n68 = Bundle("X resolution"=w119, "Y resolution"=w118, "X offset (um)"=w117, "Y offset (um)"=w116, "X center (um)"=w115, "Y center (um)"=w114, "X size (um)"=w113, "Y size (um)"=w112, "UL-Ang"=w111, "UR-Ang"=w110, "Line milling time (s)"=w109, "Z-step (nm)"=w108, "Lines auto pause"=w107, "Auto pause"=w106, "Mill from Bottom"=w105, "FIB FOV (um)"=w104, "SEM on"=w103, "Mill start from Last"=w95, "FIB PID on"=w94, "FIB PID reset"=w93, "FIB PID measured"=w102, "FIB PID target"=w101, "FIB PID target slope"=w100, "FIB PID P"=w99, "FIB PID I"=w98, "FIB PID D"=w97, "Emission min"=w96, "Emission min"=0.0, "Auto reheat"=w92) -> (w89:T18)  [unwired: 1 in]
                      n69 = Bundle("3D imaging paused alarm"=w147, "FIB emission limit warning"=w146, "Low limit"=w145, "High limit"=w144, "Pause 3D-ING"=w126, "Specimen current alarm"=w142, "Beam dump alarm"=w141, "Pause 3D-ING"=w126, "EHT off alarm"=w138, "Pause 3D-ING"=w126, "Pause 3D-ING"=FALSE, "Low limit"=sgl 1.5, "Low limit"=sgl 0.5, "Temperature alarm"=w139, "Pause 3D-ING"=w140, "Low limit (F)"=w143, "High limit (F)"=w137, "Temp limit auto"=w136, "Delta (F)"=w135, "Gradient limit (F/min)"=w134, "SW error warning"=w133, "Focus index warning"=w132, "Focus index low limit"=w131, "Focus index stop limit"=w130, "Run Auto Stig"=w129, "FI low limit auto"=w128, "FI stop limit auto"=w127) -> (w121:T19)  [unwired: 1 in]
                      n70 = Bundle By Name(cluster=w120, "SEM Scan Parameters"=w159, "Detector Information"=w186, "SEM Options"=w187, "Focus Index Options.Keep aspect ratio"=w188, "Focus Index Options.Show Focus Index"=w189, "Focus Index Options.Focus Index primary grid center"=w190, "Focus Index Options.X Grids"=w151, "Focus Index Options.Y Grids"=w150, "Focus Index Options.Primary X index"=w149, "Focus Index Options.Primary Y index"=w148, "Image fit to"=w191, "File Information"=w192, "Low mag SEM"=w193, "Mid Mag SEM"=w194, "FIB-SEM Angle"=w195, "Milling para"=w89, "FI Detector"=w196, "Auto Optimzation"=w197, "Images per Auto Optimization"=w198, "AF Range (nm)"=w199, "AF Steps"=w200, "AS Range (%)"=w201, "AS Steps"=w202, "AA Range (%)"=w203, "AA Steps"=w204, "X shift (nm/frame)"=w205, "Y shift (nm/frame)"=w206, "FIB Y zoom pixel (nm)"=w207, "Mail server"=w208, "Email Alert Recipients"=w209, "Alert Settings"=w121, "Reheat Parameters"=w210, "Start FIB HV DataLog"=w211, "Interval (s)"=w212) -> (w88:T1)
                    }
                    frame 2 {
                      w250 = TRUE ("Pause 3D-ING")
                      n71 = Unbundle By Name(w284) -> ("SEM Scan Parameters.Y tiles"=w256:u8, "SEM Scan Parameters.X tiles"=w251:u8, "SEM Scan Parameters"=w285:T20, "Detector Information"=w286:T8, "SEM Options"=w287:T9, "Keep aspect ratio"=w288:bool, "Show Focus Index"=w289:bool, "Focus Index primary grid center"=w290:bool, "Focus Index grid X"=w260:u8, "Focus Index grid Y"=w259:u8, "Focus Index primary X grid"=w258:u8, "Focus Index primary Y grid"=w257:u8, "Image fit to"=w291:u8, "File Information"=w292:T10, "Low mag SEM"=w293:T11, "Mid Mag SEM"=w294:T12, "FIB-SEM Angle"=w295:dbl, "Milling para"=w216:T21, "FI Detector"=w296:u16, "Auto Optimzation"=w297:bool, "Images per Auto Optimization"=w298:u16, "AF Range (nm)"=w299:sgl, "AF Steps"=w300:u8, "AS Range (%)"=w301:sgl, "AS Steps"=w302:u8, "AA Range (%)"=w303:sgl, "AA Steps"=w304:u8, "X shift (nm/frame)"=w305:dbl, "Y shift (nm/frame)"=w306:dbl, "FIB Settings"=w217:T14, "FIB Y zoom pixel (nm)"=w307:dbl, "Mail server"=w308:string, "Email Alert Recipients"=w309:string[], "Alert Settings"=w283:T15, "Reheat Parameters"=w310:T16, "Start FIB HV DataLog"=w311:bool, "Interval (s)"=w312:u16)
                      n72 = Unbundle(w217) -> ("Z-step (nm)"=w234:dbl, "Emission min"=w222:dbl, "Auto reheat"=w218:bool)  [unwired: 3 out]
                      n73 = Unbundle(w283) -> ("3D imaging paused alarm"=w282:bool, "FIB emission limit warning"=w281:bool, "Low limit"=w280:dbl, "High limit"=w279:dbl, "Specimen current alarm"=w277:bool, "Beam dump alarm"=w276:bool, "EHT off alarm"=w273:bool, "Temperature alarm"=w274:bool, "Pause 3D-ING"=w275:bool, "Low limit (F)"=w278:sgl, "High limit (F)"=w272:sgl, "Temp limit auto"=w271:bool, "Delta (F)"=w270:sgl, "Gradient limit (F/min)"=w269:sgl, "SW error warning"=w268:bool, "Focus index warning"=w267:bool, "Focus index low limit"=w266:dbl, "Focus index stop limit"=w265:sgl, "Run Auto Stig"=w264:bool, "FI low limit auto"=w263:bool, "FI stop limit auto"=w262:bool)
                      n74 = Unbundle(w216) -> ("X resolution"=w245:u32, "Y resolution"=w244:u32, "X offset (um)"=w243:sgl, "Y offset (um)"=w242:sgl, "X center (um)"=w241:sgl, "Y center (um)"=w240:sgl, "X size (um)"=w239:sgl, "Y size (um)"=w238:sgl, "UL-Ang"=w237:sgl, "UR-Ang"=w236:sgl, "Line milling time (s)"=w235:sgl, "Auto pause"=w232:bool, "Lines auto pause"=w233:u16, "Mill from Bottom"=w231:bool, "FIB FOV (um)"=w230:sgl, "Auto Profile"=w229:bool, "Mill start from Last"=w221:bool, "FIB PID on"=w220:bool, "FIB PID reset"=w219:bool, "FIB PID measured"=w228:u8, "FIB PID target"=w227:sgl, "FIB PID target slope"=w226:sgl, "FIB PID P"=w225:sgl, "FIB PID I"=w224:sgl, "FIB PID D"=w223:sgl)
                      n75 = Initialize Array(w260, w256, w251) -> (w255:u8[][])
                      n76 = Initialize Array(w259, w256, w251) -> (w254:u8[][])
                      n77 = Initialize Array(w258, w256, w251) -> (w253:u8[][])
                      n78 = Initialize Array(w257, w256, w251) -> (w252:u8[][])
                      n79 = Bundle("X resolution"=w245, "Y resolution"=w244, "X offset (um)"=w243, "Y offset (um)"=w242, "X center (um)"=w241, "Y center (um)"=w240, "X size (um)"=w239, "Y size (um)"=w238, "UL-Ang"=w237, "UR-Ang"=w236, "Line milling time (s)"=w235, "Z-step (nm)"=w234, "Lines auto pause"=w233, "Auto pause"=w232, "Mill from Bottom"=w231, "FIB FOV (um)"=w230, "Auto Profile"=w229, "Mill start from Last"=w221, "FIB PID on"=w220, "FIB PID reset"=w219, "FIB PID measured"=w228, "FIB PID target"=w227, "FIB PID target slope"=w226, "FIB PID P"=w225, "FIB PID I"=w224, "FIB PID D"=w223, "Emission min"=w222, "Emission min"=0.0, "Auto reheat"=w218) -> (w215:T22)  [unwired: 1 in]
                      n80 = Bundle("3D imaging paused alarm"=w282, "FIB emission limit warning"=w281, "Low limit"=w280, "High limit"=w279, "Pause 3D-ING"=w250, "Specimen current alarm"=w277, "Beam dump alarm"=w276, "Pause 3D-ING"=w250, "EHT off alarm"=w273, "Pause 3D-ING"=w250, "Pause 3D-ING"=FALSE, "Low limit"=sgl 1.5, "Low limit"=sgl 0.5, "Temperature alarm"=w274, "Pause 3D-ING"=w275, "Low limit (F)"=w278, "High limit (F)"=w272, "Temp limit auto"=w271, "Delta (F)"=w270, "Gradient limit (F/min)"=w269, "SW error warning"=w268, "Focus index warning"=w267, "Focus index low limit"=w266, "Focus index stop limit"=w265, "Run Auto Stig"=w264, "FI low limit auto"=w263, "FI stop limit auto"=w262) -> (w261:T19)  [unwired: 1 in]
                      n81 = Bundle By Name(cluster=w246, "SEM Scan Parameters"=w285, "Detector Information"=w286, "SEM Options"=w287, "Focus Index Options.Keep aspect ratio"=w288, "Focus Index Options.Show Focus Index"=w289, "Focus Index Options.Focus Index primary grid center"=w290, "Focus Index Options.X Grids"=w255, "Focus Index Options.Y Grids"=w254, "Focus Index Options.Primary X index"=w253, "Focus Index Options.Primary Y index"=w252, "Image fit to"=w291, "File Information"=w292, "Low mag SEM"=w293, "Mid Mag SEM"=w294, "FIB-SEM Angle"=w295, "Milling para"=w215, "FI Detector"=w296, "Auto Optimzation"=w297, "Images per Auto Optimization"=w298, "AF Range (nm)"=w299, "AF Steps"=w300, "AS Range (%)"=w301, "AS Steps"=w302, "AA Range (%)"=w303, "AA Steps"=w304, "X shift (nm/frame)"=w305, "Y shift (nm/frame)"=w306, "FIB Y zoom pixel (nm)"=w307, "Mail server"=w308, "Email Alert Recipients"=w309, "Alert Settings"=w261, "Reheat Parameters"=w310, "Start FIB HV DataLog"=w311, "Interval (s)"=w312) -> (w214:T1)
                    }
                    frame 4 {
                      n82 = Unbundle By Name(w356) -> ("SEM Scan Parameters.Y tiles"=w361:u8, "SEM Scan Parameters.X tiles"=w352:u8, "SEM Scan Parameters"=w387:T20, "Detector Information"=w388:T8, "SEM Options"=w389:T9, "Keep aspect ratio"=w390:bool, "Show Focus Index"=w391:bool, "Focus Index primary grid center"=w392:bool, "Focus Index grid X"=w365:u8, "Focus Index grid Y"=w364:u8, "Focus Index primary X grid"=w363:u8, "Focus Index primary Y grid"=w362:u8, "Image fit to"=w393:u8, "File Information"=w394:T10, "Low mag SEM"=w395:T11, "Mid Mag SEM"=w396:T12, "FIB-SEM Angle"=w397:dbl, "Milling para"=w314:T21, "FI Detector"=w398:u16, "Auto Optimzation"=w399:bool, "Images per Auto Optimization"=w400:u16, "AF Range (nm)"=w401:sgl, "AF Steps"=w402:u8, "AS Range (%)"=w403:sgl, "AS Steps"=w404:u8, "AA Range (%)"=w405:sgl, "AA Steps"=w406:u8, "X shift (nm/frame)"=w407:dbl, "Y shift (nm/frame)"=w408:dbl, "FIB Settings"=w316:T14, "FIB Y zoom pixel (nm)"=w409:dbl, "Mail server"=w410:string, "Email Alert Recipients"=w411:string[], "Alert Settings"=w386:T23, "Reheat Parameters"=w412:T16, "Start FIB HV DataLog"=w413:bool, "Interval (s)"=w414:u16)
                      n83 = Unbundle(w316) -> ("Z-step (nm)"=w333:dbl, "Emission min"=w321:dbl, "Auto reheat"=w317:bool)  [unwired: 3 out]
                      n84 = Unbundle(w386) -> ("3D imaging paused alarm"=w385:bool, "FIB emission limit warning"=w384:bool, "Low limit"=w383:dbl, "High limit"=w382:dbl, "Specimen @ SEM alarm"=w381:bool, "FIB CL current alarm"=w380:bool, "Beam Dump 1 alarm"=w378:bool, "Milling Y voltage alarm"=w379:bool, "EHT off alarm"=w353:bool, "Temperature alarm"=w348:bool, "Pause 3D-ING"=w377:bool, "Low limit (F)"=w376:sgl, "High limit (F)"=w375:sgl, "Temp limit auto"=w374:bool, "Delta (F)"=w373:sgl, "Gradient limit (F/min)"=w372:sgl, "SW error warning"=w371:bool, "Focus index warning"=w370:bool, "Focus index low limit"=w369:sgl, "Focus index stop limit"=w368:sgl, "Run Auto Stig"=w367:bool, "FI low limit auto"=w355:bool, "FI stop limit auto"=w354:bool)
                      n85 = Unbundle(w314) -> ("X resolution"=w344:u32, "Y resolution"=w343:u32, "X offset (um)"=w342:sgl, "Y offset (um)"=w341:sgl, "X center (um)"=w340:sgl, "Y center (um)"=w339:sgl, "X size (um)"=w338:sgl, "Y size (um)"=w337:sgl, "UL-Ang"=w336:sgl, "UR-Ang"=w335:sgl, "Line milling time (s)"=w334:sgl, "Auto pause"=w331:bool, "Lines auto pause"=w332:u16, "Mill from Bottom"=w330:bool, "FIB FOV (um)"=w329:sgl, "Auto Profile"=w328:bool, "Mill start from Last"=w320:bool, "FIB PID on"=w319:bool, "FIB PID reset"=w318:bool, "FIB PID measured"=w327:u8, "FIB PID target"=w326:sgl, "FIB PID target slope"=w325:sgl, "FIB PID P"=w324:sgl, "FIB PID I"=w323:sgl, "FIB PID D"=w322:sgl)
                      n86 = Initialize Array(w365, w361, w352) -> (w360:u8[][])
                      n87 = Initialize Array(w364, w361, w352) -> (w359:u8[][])
                      n88 = Initialize Array(w363, w361, w352) -> (w358:u8[][])
                      n89 = Initialize Array(w362, w361, w352) -> (w357:u8[][])
                      n90 = Bundle("X resolution"=w344, "Y resolution"=w343, "X offset (um)"=w342, "Y offset (um)"=w341, "X center (um)"=w340, "Y center (um)"=w339, "X size (um)"=w338, "Y size (um)"=w337, "UL-Ang"=w336, "UR-Ang"=w335, "Line milling time (s)"=w334, "Z-step (nm)"=w333, "Lines auto pause"=w332, "Auto pause"=w331, "Mill from Bottom"=w330, "FIB FOV (um)"=w329, "Auto Profile"=w328, "Mill start from Last"=w320, "FIB PID on"=w319, "FIB PID reset"=w318, "FIB PID measured"=w327, "FIB PID target"=w326, "FIB PID target slope"=w325, "FIB PID P"=w324, "FIB PID I"=w323, "FIB PID D"=w322, "Emission min"=w321, "Emission min"=0.0, "Auto reheat"=w317) -> (w315:T22)  [unwired: 1 in]
                      n91 = Bundle("3D imaging paused alarm"=w385, "FIB emission limit warning"=w384, "Low limit"=w383, "High limit"=w382, "Specimen @ SEM alarm"=w381, "FIB CL current alarm"=w380, "Beam Dump 1 alarm"=w378, "Milling Y voltage alarm"=w379, "EHT off alarm"=w353, "Pause 3D-ING"=TRUE, "Pause 3D-ING"=FALSE, "Low limit"=sgl 1.5, "Low limit"=sgl 0.5, "Temperature alarm"=w348, "Pause 3D-ING"=w377, "Low limit (F)"=w376, "High limit (F)"=w375, "Temp limit auto"=w374, "Delta (F)"=w373, "Gradient limit (F/min)"=w372, "SW error warning"=w371, "Focus index warning"=w370, "Focus index low limit"=w369, "Focus index stop limit"=w368, "Run Auto Stig"=w367, "FI low limit auto"=w355, "FI stop limit auto"=w354) -> (w366:T24)  [unwired: 1 in]
                      n92 = Bundle By Name(cluster=w346, "SEM Scan Parameters"=w387, "Detector Information"=w388, "SEM Options"=w389, "Focus Index Options.Keep aspect ratio"=w390, "Focus Index Options.Show Focus Index"=w391, "Focus Index Options.Focus Index primary grid center"=w392, "Focus Index Options.X Grids"=w360, "Focus Index Options.Y Grids"=w359, "Focus Index Options.Primary X index"=w358, "Focus Index Options.Primary Y index"=w357, "Image fit to"=w393, "File Information"=w394, "Low mag SEM"=w395, "Mid Mag SEM"=w396, "FIB-SEM Angle"=w397, "Milling para"=w315, "FI Detector"=w398, "Auto Optimzation"=w399, "Images per Auto Optimization"=w400, "AF Range (nm)"=w401, "AF Steps"=w402, "AS Range (%)"=w403, "AS Steps"=w404, "AA Range (%)"=w405, "AA Steps"=w406, "X shift (nm/frame)"=w407, "Y shift (nm/frame)"=w408, "FIB Y zoom pixel (nm)"=w409, "Mail server"=w410, "Email Alert Recipients"=w411, "Alert Settings"=w366, "Reheat Parameters"=w412, "Start FIB HV DataLog"=w413, "Interval (s)"=w414) -> (w345:T1)
                    }
                    frame 8 {
                      n93 = Unbundle By Name(w448) -> ("SEM Scan Parameters"=w451:T20, "Detector Information"=w452:T8, "SEM Options"=w453:T9, "Focus Index Options"=w454:T25, "Image fit to"=w455:u8, "File Information"=w456:T10, "Low mag SEM"=w457:T11, "Mid Mag SEM"=w458:T12, "FIB-SEM Angle"=w459:dbl, "Milling para"=w446:T21, "FI Detector"=w460:u16, "Auto Optimzation"=w461:bool, "Images per Auto Optimization"=w462:u16, "AF Range (nm)"=w463:sgl, "AF Steps"=w464:u8, "AS Range (%)"=w465:sgl, "AS Steps"=w466:u8, "AA Range (%)"=w467:sgl, "AA Steps"=w468:u8, "X shift (nm/frame)"=w469:dbl, "Y shift (nm/frame)"=w470:dbl, "FIB Settings"=w445:T14, "FIB Y zoom pixel (nm)"=w471:dbl, "Mail server"=w472:string, "Email Alert Recipients"=w473:string[], "Alert Settings"=w447:T26, "Reheat Parameters"=w474:T16, "Start FIB HV DataLog"=w475:bool, "Interval (s)"=w476:u16)
                      n94 = Unbundle(w445) -> ("Z-step (nm)"=w433:dbl, "Emission min"=w421:dbl, "Auto reheat"=w416:bool)  [unwired: 3 out]
                      n95 = Unbundle(w446) -> ("X resolution"=w444:u32, "Y resolution"=w443:u32, "X offset (um)"=w442:sgl, "Y offset (um)"=w441:sgl, "X center (um)"=w440:sgl, "Y center (um)"=w439:sgl, "X size (um)"=w438:sgl, "Y size (um)"=w437:sgl, "UL-Ang"=w436:sgl, "UR-Ang"=w435:sgl, "Line milling time (s)"=w434:sgl, "Auto pause"=w431:bool, "Lines auto pause"=w432:u16, "Mill from Bottom"=w430:bool, "FIB FOV (um)"=w429:sgl, "Auto Profile"=w428:bool, "Mill start from Last"=w419:bool, "FIB PID on"=w418:bool, "FIB PID reset"=w417:bool, "FIB PID measured"=w427:u8, "FIB PID target"=w426:sgl, "FIB PID target slope"=w425:sgl, "FIB PID P"=w424:sgl, "FIB PID I"=w423:sgl, "FIB PID D"=w422:sgl)
                      n96 = Bundle("X resolution"=w444, "Y resolution"=w443, "X offset (um)"=w442, "Y offset (um)"=w441, "X center (um)"=w440, "Y center (um)"=w439, "X size (um)"=w438, "Y size (um)"=w437, "UL-Ang"=w436, "UR-Ang"=w435, "Line milling time (s)"=w434, "Z-step (nm)"=w433, "Lines auto pause"=w432, "Auto pause"=w431, "Mill from Bottom"=w430, "FIB FOV (um)"=w429, "Auto Profile"=w428, "Mill start from Last"=w419, "FIB PID on"=w418, "FIB PID reset"=w417, "FIB PID measured"=w427, "FIB PID target"=w426, "FIB PID target slope"=w425, "FIB PID P"=w424, "FIB PID I"=w423, "FIB PID D"=w422, "Emission min"=w421, "Emission min"=0.0, "Auto reheat"=w416) -> (w420:T22)  [unwired: 1 in]
                      n97 = Bundle By Name(cluster=w450, "SEM Scan Parameters"=w451, "Detector Information"=w452, "SEM Options"=w453, "Focus Index Options"=w454, "Image fit to"=w455, "File Information"=w456, "Low mag SEM"=w457, "Mid Mag SEM"=w458, "FIB-SEM Angle"=w459, "Milling para"=w420, "FI Detector"=w460, "Auto Optimzation"=w461, "Images per Auto Optimization"=w462, "AF Range (nm)"=w463, "AF Steps"=w464, "AS Range (%)"=w465, "AS Steps"=w466, "AA Range (%)"=w467, "AA Steps"=w468, "X shift (nm/frame)"=w469, "Y shift (nm/frame)"=w470, "FIB Y zoom pixel (nm)"=w471, "Mail server"=w472, "Email Alert Recipients"=w473, "Alert Settings"=w447, "Reheat Parameters"=w474, "Start FIB HV DataLog"=w475, "Interval (s)"=w476) -> (w449:T1)
                    }
                    frame 16 {
                    }
                  }
                }
                frame True {
                  w496 = 2
                  w504 = 3
                  w511 = 9
                  w532 = 2
                  w541 = 2
                  w556 = 4
                  w570 = 4
                  w615 = 5
                  w613 = 3
                  w596 = 9
                  w631 = 2
                  w486 = 8
                  w648 = 3
                  w665 = 3
                  w683 = 3
                  w633 = 2
                  w700 = 2
                  w701 = 2
                  w534 = 7
                  w707 = 2
                  w709 = 2
                  w479 = 9
                  w851 = 90.0 ("t")
                  w877 = 22
                  w597 = 0 ("index")
                  n98 = call-poly <vilib>:"Read From Spreadsheet File.vi"("delimiter (\\t)"="," ("delimiter (\\t)"), "file path (dialog if empty)"=w742) -> ("all rows"=w485:string[][])  [unwired: 5 in, 4 out]
                  n99 = local read "Recipe items"() -> (w478:string[])
                  n100 = Add(x=w597, y=w596) -> (x+y=w564:i32)
                  n101 = Increment(x=w564) -> (x+1=w572:i32)
                  n102 = Increment(x=w572) -> (x+1=w571:i32)
                  n103 = Add(x=w571, y=w570) -> (x+y=w616:i32)
                  n104 = Add(x=w616, y=w615) -> (x+y=w614:i32)
                  n105 = Add(x=w614, y=w613) -> (x+y=w903:i32)
                  n106 = Increment(x=w903) -> (x+1=w902:i32)
                  n107 = Increment(x=w902) -> (x+1=w901:i32)
                  n108 = Increment(x=w901) -> (x+1=w900:i32)
                  n109 = Increment(x=w900) -> (x+1=w904:i32)
                  n110 = Increment(x=w904) -> (x+1=w876:i32)
                  n111 = Add(x=w876, y=w877) -> (x+y=w868:i32)
                  n112 = Increment(x=w868) -> (x+1=w867:i32)
                  n113 = Increment(x=w867) -> (x+1=w557:i32)
                  n114 = Increment(x=w557) -> (x+1=w543:i32)
                  n115 = Add(x=w543, y=w556) -> (x+y=w724:i32)
                  n116 = Increment(x=w724) -> (x+1=w892:i32)
                  n117 = Increment(x=w892) -> (x+1=w845:i32)
                  n118 = Increment(x=w845) -> (x+1=w843:i32)
                  n119 = for {
                    N: w877 -> [_]
                    tunnel: w876 -> [w1393]
                    tunnel: [w1392] -> w1019 mode=indexing
                    i -> [w1394]
                    n120 = Add(x=w1393, y=w1394) -> (x+y=w1392:i32)
                  }
                  n121 = for {
                    N: w596 -> [_]
                    tunnel: w597 -> [w1203]
                    tunnel: [w1202] -> w625 mode=indexing
                    i -> [w1204]
                    n122 = Add(x=w1203, y=w1204) -> (x+y=w1202:i32)
                  }
                  n123 = Index Array(array=w478, index=w564) -> (element=w599:string)
                  n124 = Index Array(array=w478, index=w572) -> (element=w575:string)
                  n125 = for {
                    N: w570 -> [_]
                    tunnel: w571 -> [w1158]
                    tunnel: [w1157] -> w573 mode=indexing
                    i -> [w1159]
                    n126 = Add(x=w1158, y=w1159) -> (x+y=w1157:i32)
                  }
                  n127 = for {
                    N: w615 -> [_]
                    tunnel: w616 -> [w1184]
                    tunnel: [w1183] -> w619 mode=indexing
                    i -> [w1185]
                    n128 = Add(x=w1184, y=w1185) -> (x+y=w1183:i32)
                  }
                  n129 = for {
                    N: w613 -> [_]
                    tunnel: w614 -> [w1170]
                    tunnel: [w1169] -> w618 mode=indexing
                    i -> [w1171]
                    n130 = Add(x=w1170, y=w1171) -> (x+y=w1169:i32)
                  }
                  n131 = Index Array(array=w478, index=w903) -> (element=w1042:string)
                  n132 = Index Array(array=w478, index=w902) -> (element=w1043:string)
                  n133 = Index Array(array=w478, index=w901) -> (element=w1028:string)
                  n134 = Index Array(array=w478, index=w900) -> (element=w1029:string)
                  n135 = Index Array(array=w478, index=w904) -> (element=w1037:string)
                  n136 = Index Array(array=w478, index=w868) -> (element=w879:string)
                  n137 = Index Array(array=w478, index=w867) -> (element=w870:string)
                  n138 = Index Array(array=w478, index=w557) -> (element=w898:string)
                  n139 = for {
                    N: w556 -> [_]
                    tunnel: w543 -> [w1122]
                    tunnel: [w1121] -> w559 mode=indexing
                    i -> [w1123]
                    n140 = Add(x=w1122, y=w1123) -> (x+y=w1121:i32)
                  }
                  n141 = Index Array(array=w478, index=w724) -> (element=w729:string)
                  n142 = Index Array(array=w478, index=w892) -> (element=w1016:string)
                  n143 = Index Array(array=w478, index=w845) -> (element=w1006:string)
                  n144 = Index Array(array=w478, index=w843) -> (element=w846:string)
                  n145 = call "2D array search.vi"("Search For"=w599, "Input Array"=w485) -> ("Column"=w598:i32, "Row"=w591:i32)  [unwired: 7 in, 1 out]
                  n146 = call "2D array search.vi"("Search For"=w575, "Input Array"=w485) -> ("Column"=w576:i32, "Row"=w581:i32)  [unwired: 7 in, 1 out]
                  n147 = call "2D array search.vi"("Search For"=w1042, "Input Array"=w485) -> ("Column"=w1046:i32, "Row"=w1048:i32)  [unwired: 7 in, 1 out]
                  n148 = call "2D array search.vi"("Search For"=w1043, "Input Array"=w485) -> ("Column"=w1049:i32, "Row"=w1051:i32)  [unwired: 7 in, 1 out]
                  n149 = call "2D array search.vi"("Search For"=w1028, "Input Array"=w485) -> ("Column"=w1031:i32, "Row"=w1033:i32)  [unwired: 7 in, 1 out]
                  n150 = call "2D array search.vi"("Search For"=w1029, "Input Array"=w485) -> ("Column"=w1034:i32, "Row"=w1036:i32)  [unwired: 7 in, 1 out]
                  n151 = call "2D array search.vi"("Search For"=w1037, "Input Array"=w485) -> ("Column"=w1039:i32, "Row"=w1041:i32)  [unwired: 7 in, 1 out]
                  n152 = call "2D array search.vi"("Search For"=w879, "Input Array"=w485) -> ("Column"=w880:i32, "Row"=w882:i32)  [unwired: 7 in, 1 out]
                  n153 = call "2D array search.vi"("Search For"=w870, "Input Array"=w485) -> ("Column"=w871:i32, "Row"=w873:i32)  [unwired: 7 in, 1 out]
                  n154 = call "2D array search.vi"("Search For"=w898, "Input Array"=w485) -> ("Column"=w897:i32, "Row"=w895:i32)  [unwired: 7 in, 1 out]
                  n155 = call "2D array search.vi"("Search For"=w729, "Input Array"=w485) -> ("Column"=w727:i32, "Row"=w725:i32)  [unwired: 7 in, 1 out]
                  n156 = call "2D array search.vi"("Search For"=w1016, "Input Array"=w485) -> ("Column"=w1015:i32, "Row"=w1013:i32)  [unwired: 7 in, 1 out]
                  n157 = call "2D array search.vi"("Search For"=w1006, "Input Array"=w485) -> ("Column"=w1007:i32, "Row"=w1008:i32)  [unwired: 7 in, 1 out]
                  n158 = call "2D array search.vi"("Search For"=w846, "Input Array"=w485) -> ("Column"=w847:i32, "Row"=w849:i32)  [unwired: 7 in, 1 out]
                  n159 = for {
                    tunnel: w478 -> [w1400]
                    tunnel: w485 -> [w1399]
                    tunnel: [w1396] -> w1018 mode=indexing
                    tunnel: w1019 -> [w1395] mode=indexing
                    n160 = Index Array(array=w1400, index=w1395) -> (element=w1398:string)
                    n161 = call "2D array search.vi"("Search For"=w1398, "Input Array"=w1399) -> ("Column"=w1404:i32, "Row"=w1402:i32)  [unwired: 7 in, 1 out]
                    n162 = Increment(x=w1404) -> (x+1=w1403:i32)
                    n163 = Index Array(array=w1399, index (row)=w1402, index (col)=w1403) -> (element=w1397:string)
                    n164 = Match True/False String(2:"FALSE" ("true string"), 3:"TRUE" ("true string"), 4:w1397) -> (0:w1396:bool)  [unwired: 1 out]
                  }
                  n165 = Increment(x=w598) -> (x+1=w589:i32)
                  n166 = Increment(x=w576) -> (x+1=w583:i32)
                  n167 = for {
                    tunnel: w478 -> [w1210]
                    tunnel: w485 -> [w1209]
                    tunnel: w625 -> [w1207] mode=indexing
                    tunnel: [w1205] -> w624 mode=indexing
                    n168 = Index Array(array=w1210, index=w1207) -> (element=w1208:string)
                    n169 = call "2D array search.vi"("Search For"=w1208, "Input Array"=w1209) -> ("Column"=w1213:i32, "Row"=w1211:i32)  [unwired: 7 in, 1 out]
                    n170 = Increment(x=w1213) -> (x+1=w1212:i32)
                    n171 = Index Array(array=w1209, index (row)=w1211, index (col)=w1212) -> (element=w1206:string)
                    n172 = Fract/Exp String To Number(string=w1206) -> (number=w1205:dbl)  [unwired: 4 out]
                  }
                  n173 = for {
                    tunnel: w478 -> [w1165]
                    tunnel: w485 -> [w1164]
                    tunnel: w573 -> [w1162] mode=indexing
                    tunnel: [w1160] -> w574 mode=indexing
                    n174 = Index Array(array=w1165, index=w1162) -> (element=w1163:string)
                    n175 = call "2D array search.vi"("Search For"=w1163, "Input Array"=w1164) -> ("Column"=w1168:i32, "Row"=w1166:i32)  [unwired: 7 in, 1 out]
                    n176 = Increment(x=w1168) -> (x+1=w1167:i32)
                    n177 = Index Array(array=w1164, index (row)=w1166, index (col)=w1167) -> (element=w1161:string)
                    n178 = Fract/Exp String To Number(string=w1161) -> (number=w1160:dbl)  [unwired: 4 out]
                  }
                  n179 = for {
                    tunnel: w478 -> [w1179]
                    tunnel: w485 -> [w1178]
                    tunnel: w618 -> [w1176] mode=indexing
                    tunnel: [w1172] -> w617 mode=indexing
                    n180 = Index Array(array=w1179, index=w1176) -> (element=w1177:string)
                    n181 = call "2D array search.vi"("Search For"=w1177, "Input Array"=w1178) -> ("Column"=w1182:i32, "Row"=w1180:i32)  [unwired: 7 in, 1 out]
                    n182 = Increment(x=w1182) -> (x+1=w1181:i32)
                    n183 = Index Array(array=w1178, index (row)=w1180, index (col)=w1181) -> (element=w1173:string)
                    n184 = Match True/False String(2:"FALSE" ("true string"), 3:"TRUE" ("true string"), 4:w1173) -> (0:w1172:bool)  [unwired: 1 out]
                  }
                  n185 = Increment(x=w1046) -> (x+1=w1047:i32)
                  n186 = Increment(x=w1049) -> (x+1=w1050:i32)
                  n187 = Increment(x=w1031) -> (x+1=w1032:i32)
                  n188 = Increment(x=w1034) -> (x+1=w1035:i32)
                  n189 = Increment(x=w1039) -> (x+1=w1040:i32)
                  n190 = Increment(x=w880) -> (x+1=w881:i32)
                  n191 = Increment(x=w871) -> (x+1=w872:i32)
                  n192 = Increment(x=w897) -> (x+1=w896:i32)
                  n193 = Increment(x=w727) -> (x+1=w726:i32)
                  n194 = Increment(x=w1015) -> (x+1=w1014:i32)
                  n195 = Increment(x=w847) -> (x+1=w848:i32)
                  n196 = while {
                    tunnel: w1008 -> [w1384]
                    tunnel: w1007 -> [w1391]
                    tunnel: [w1387] -> w928 mode=indexing
                    tunnel: w485 -> [w1385]
                    i -> [w1389]
                    stop <- w1386 stop-if-true
                    n197 = Increment(x=w1391) -> (x+1=w1390:i32)
                    n198 = Add(x=w1390, y=w1389) -> (x+y=w1383:i32)
                    n199 = Increment(x=w1383) -> (x+1=w1382:i32)
                    n200 = Index Array(array=w1385, index (row)=w1384, index (col)=w1383) -> (element=w1387:string)
                    n201 = Index Array(array=w1385, index (row)=w1384, index (col)=w1382) -> (element=w1381:string)
                    n202 = Equal?(x=w1381, y="") -> (x = y?=w1386:bool)
                  }
                  n203 = Array Subset(array=w485, index (row)=w591, length (row)=1 ("disabled index (col)"), index (col)=w589) -> (w588:string[][])  [unwired: 1 in]
                  n204 = Array Subset(array=w485, index (row)=w581, length (row)=1 ("disabled index (col)"), index (col)=w583) -> (w584:string[][])  [unwired: 1 in]
                  n205 = Index Array(array=w574) -> (element #1=w566:dbl, element #2=w567:dbl, element #3=w568:dbl, element #4=w569:dbl)  [unwired: 4 in]
                  n206 = Index Array(array=w485, index (row)=w1048, index (col)=w1047) -> (element=w1045:string)
                  n207 = Index Array(array=w485, index (row)=w1051, index (col)=w1050) -> (element=w1044:string)
                  n208 = Index Array(array=w485, index (row)=w1033, index (col)=w1032) -> (element=w1024:string)
                  n209 = Index Array(array=w485, index (row)=w1036, index (col)=w1035) -> (element=w1030:string)
                  n210 = Index Array(array=w485, index (row)=w1041, index (col)=w1040) -> (element=w1038:string)
                  n211 = Index Array(array=w485, index (row)=w882, index (col)=w881) -> (element=w883:string)
                  n212 = Index Array(array=w485, index (row)=w873, index (col)=w872) -> (element=w874:string)
                  n213 = Index Array(array=w485, index (row)=w895, index (col)=w896) -> (element=w894:string)
                  n214 = Index Array(array=w485, index (row)=w725, index (col)=w726) -> (element=w728:string)
                  n215 = Index Array(array=w485, index (row)=w1013, index (col)=w1014) -> (element=w1012:string)
                  n216 = Index Array(array=w485, index (row)=w849, index (col)=w848) -> (element=w844:string)
                  n217 = Fract/Exp String To Number(string=w1045) -> (number=w1026:dbl)  [unwired: 4 out]
                  n218 = Fract/Exp String To Number(string=w1044) -> (number=w1025:dbl)  [unwired: 4 out]
                  n219 = Fract/Exp String To Number(string=w1030) -> (number=w1022:dbl)  [unwired: 4 out]
                  n220 = Fract/Exp String To Number(string=w1038) -> (number=w1023:dbl)  [unwired: 4 out]
                  n221 = Match True/False String(2:"FALSE" ("true string"), 3:"TRUE" ("true string"), 4:w883) -> (0:w551:bool)  [unwired: 1 out]
                  n222 = Match True/False String(2:"FALSE" ("true string"), 3:"TRUE" ("true string"), 4:w874) -> (0:w550:bool)  [unwired: 1 out]
                  n223 = Match True/False String(2:"FALSE" ("true string"), 3:"TRUE" ("true string"), 4:w894) -> (0:w549:bool)  [unwired: 1 out]
                  n224 = Fract/Exp String To Number(string=w728) -> (number=w723:dbl)  [unwired: 4 out]
                  n225 = String To Path(string=w1012) -> (path=w1009:path)
                  n226 = local read "Read output"() -> (w1011:T1)
                  n227 = local read "Read output"() -> (w553:T1)
                  n228 = Unbundle By Name(w553) -> ("Focus Index Options"=w552:T25)
                  n229 = local read "Read output"() -> (w1021:T1)
                  n230 = Unbundle By Name(w1021) -> ("Detector Information"=w1027:T8)
                  n231 = Array To Cluster(array=w1018) -> (cluster=w1017:T27)
                  n232 = local read "Read output"() -> (w1053:T1)
                  n233 = Unbundle By Name(w1053) -> ("SEM Scan Parameters"=w1054:T20)
                  n234 = Index Array(array=w624) -> (element #1=w600:dbl, element #2=w623:dbl, element #3=w622:dbl, element #4=w621:dbl, element #5=w620:dbl, element #6=w601:dbl, element #7=w555:dbl, element #8=w554:dbl, element #9=w602:dbl)  [unwired: 9 in]
                  n235 = for {
                    tunnel: w478 -> [w1199]
                    tunnel: w485 -> [w1198]
                    tunnel: w619 -> [w1196] mode=indexing
                    tunnel: w554 -> [w1192]
                    tunnel: w555 -> [w1191]
                    tunnel: [w1186] -> w612 mode=indexing
                    n236 = Index Array(array=w1199, index=w1196) -> (element=w1197:string)
                    n237 = call "2D array search.vi"("Search For"=w1197, "Input Array"=w1198) -> ("Column"=w1201:i32, "Row"=w1200:i32)  [unwired: 7 in, 1 out]
                    n238 = Increment(x=w1201) -> (x+1=w1195:i32)
                    n239 = Array Subset(array=w1198, index (row)=w1200, length (row)=1 ("length"), index (col)=w1195) -> (w1193:string[][])  [unwired: 1 in]
                    n240 = Reshape Array(w1193, w1192, w1191) -> (w1187:string[][])
                    n241 = Array To Spreadsheet String(array=w1187, 3:"%s" ("format string")) -> (spreadsheet string=w1188:string)  [unwired: 1 in]
                    n242 = Spreadsheet String To Array(format string="%f", spreadsheet string=w1188) -> (array=w1186:dbl[][])  [unwired: 2 in]
                  }
                  n243 = for {
                    tunnel: w478 -> [w1139]
                    tunnel: w485 -> [w1127]
                    tunnel: w559 -> [w1137] mode=indexing
                    tunnel: w554 -> [w1132]
                    tunnel: w555 -> [w1131]
                    tunnel: [w1135] -> w558 mode=indexing
                    n244 = Index Array(array=w1139, index=w1137) -> (element=w1138:string)
                    n245 = call "2D array search.vi"("Search For"=w1138, "Input Array"=w1127) -> ("Column"=w1140:i32, "Row"=w1125:i32)  [unwired: 7 in, 1 out]
                    n246 = Multiply(x=w1131, y=w1132) -> (x*y=w1130:dbl)
                    n247 = Increment(x=w1140) -> (x+1=w1126:i32)
                    n248 = To Long Integer(number=w1130) -> (32bit integer=w1128:i32)
                    n249 = Array Subset(array=w1127, index (row)=w1125, length (row)=1 ("length"), index (col)=w1126) -> (w1134:string[][])  [unwired: 1 in]
                    n250 = Array Size(array=w1134) -> (size(s)=w1133:i32[])
                    n251 = Multiply Array Elements(1:w1133) -> (0:w1129:i32)
                    n252 = Equal?(x=w1128, y=w1129) -> ()  [unwired: 1 out]
                    n253 = case shown="False" TRUE {
                      tunnel: w1134 -> [_ w1156]
                      tunnel: w1132 -> [w1142 w1155]
                      tunnel: w1131 -> [w1141 w1154]
                      tunnel: [w1143 w1149] -> w1135
                      tunnel: w1127 -> [w1147 _]
                      tunnel: w1126 -> [w1146 _]
                      tunnel: w1125 -> [w1145 _]
                      frame False {
                        n254 = Index Array(array=w1147, index (row)=w1145, index (col)=w1146) -> (element=w1148:string)
                        n255 = Fract/Exp String To Number(string=w1148) -> (number=w1144:dbl)  [unwired: 4 out]
                        n256 = Initialize Array(w1144, w1142, w1141) -> (w1143:dbl[][])
                      }
                      frame True {
                        n257 = Reshape Array(w1156, w1155, w1154) -> (w1150:string[][])
                        n258 = Array To Spreadsheet String(array=w1150, 3:"%s" ("format string")) -> (spreadsheet string=w1151:string)  [unwired: 1 in]
                        n259 = Spreadsheet String To Array(format string="%f", spreadsheet string=w1151) -> (array=w1149:dbl[][])  [unwired: 2 in]
                      }
                    }
                  }
                  n260 = Reshape Array(w588, w554) -> (w595:string[])
                  n261 = Reshape Array(w584, w555) -> (w577:string[])
                  n262 = Array To Spreadsheet String(array=w595, 3:"%s" ("format string")) -> (spreadsheet string=w594:string)  [unwired: 1 in]
                  n263 = Array To Spreadsheet String(array=w577, 3:"%s" ("format string")) -> (spreadsheet string=w578:string)  [unwired: 1 in]
                  n264 = Index Array(array=w612) -> (element #1=w611:dbl[][], element #2=w610:dbl[][], element #3=w609:dbl[][], element #4=w608:dbl[][], element #5=w607:dbl[][])  [unwired: 15 in]
                  n265 = Index Array(array=w558) -> (element #1=w548:dbl[][], element #2=w547:dbl[][], element #3=w546:dbl[][], element #4=w545:dbl[][])  [unwired: 12 in]
                  n266 = Spreadsheet String To Array(format string="%f", spreadsheet string=w594, array type (2D Dbl)=dbl[] []) -> (array=w586:dbl[])  [unwired: 1 in]
                  n267 = Spreadsheet String To Array(format string="%f", spreadsheet string=w578, array type (2D Dbl)=dbl[] []) -> (array=w565:dbl[])  [unwired: 1 in]
                  n268 = Bundle By Name(cluster=w552, "Keep aspect ratio"=w551, "Show Focus Index"=w550, "Focus Index primary grid center"=w549, "X Grids"=w548, "Y Grids"=w547, "Primary X index"=w546, "Primary Y index"=w545) -> (w544:T25)
                  n269 = Index Array(array=w617) -> (element #1=w606:bool, element #2=w605:bool, element #3=w604:bool)  [unwired: 3 in]
                  n270 = Bundle By Name(cluster=w1054, "X size (um)"=w600, "Y size (um)"=w623, "X center (um)"=w622, "Y center (um)"=w621, "X size (V)"=w620, "Frames"=w601, "X tiles"=w555, "Y tiles"=w554, "Overlap (um)"=w602, "dX (um)"=w586, "dY (um)"=w565, "Scan rate (Hz)"=w566, "Pixel size (nm)"=w567, "Frame line rampdown ratio"=w568, "Oversampling"=w569, "X stig"=w611, "Y stig"=w610, "X aln"=w609, "Y aln"=w608, "WD (mm)"=w607, "X size auto"=w606, "Oversampling auto"=w605, "Interlaced"=w604) -> (w1052:T20)
                  n271 = Bundle By Name(cluster=w1027, "Brightness A"=w1026, "Contrast A"=w1025, "Detector B name"=w1024, "Brightness B"=w1022, "Contrast B"=w1023) -> (w1020:T8)
                  n272 = Unbundle By Name(w1011) -> ("File Information"=w1010:T10)
                  n273 = Array To Spreadsheet String(delimiter (Tab)="," ("string"), array=w928, 3:"%s" ("format string")) -> (spreadsheet string=w920:string)
                  n274 = Search and Replace String(input string=w920, search string="\r\n", replace string="") -> (result string=w923:string)  [unwired: 5 in, 3 out]
                  n275 = call "String trim.vi"("Match string"="\"" ("string"), "Input string"=w923) -> ("Ouput string"=w925:string)  [unwired: 9 in]
                  n276 = Bundle By Name(cluster=w1010, "File path"=w1009, "Notes"=w925, "Sample ID"=w844) -> (w1005:T10)
                  n277 = Increment(x=w843) -> (x+1=w891:i32)
                  n278 = Increment(x=w891) -> (x+1=w890:i32)
                  n279 = Increment(x=w890) -> (x+1=w889:i32)
                  n280 = Increment(x=w889) -> (x+1=w888:i32)
                  n281 = Increment(x=w888) -> (x+1=w887:i32)
                  n282 = Increment(x=w887) -> (x+1=w776:i32)
                  n283 = Increment(x=w776) -> (x+1=w819:i32)
                  n284 = Increment(x=w819) -> (x+1=w820:i32)
                  n285 = Increment(x=w820) -> (x+1=w821:i32)
                  n286 = Increment(x=w821) -> (x+1=w822:i32)
                  n287 = Increment(x=w822) -> (x+1=w751:i32)
                  n288 = Increment(x=w751) -> (x+1=w772:i32)
                  n289 = Increment(x=w772) -> (x+1=w773:i32)
                  n290 = Increment(x=w773) -> (x+1=w774:i32)
                  n291 = Increment(x=w774) -> (x+1=w750:i32)
                  n292 = Increment(x=w750) -> (x+1=w522:i32)
                  n293 = Add(x=w522, y=1) -> (x+y=w512:i32)
                  n294 = Add(x=w512, y=w511) -> (x+y=w510:i32)
                  n295 = Increment(x=w510) -> (x+1=w498:i32)
                  n296 = Increment(x=w498) -> (x+1=w505:i32)
                  n297 = Add(x=w505, y=w504) -> (x+y=w497:i32)
                  n298 = Add(x=w497, y=w496) -> (x+y=w495:i32)
                  n299 = Increment(x=w495) -> (x+1=w835:i32)
                  n300 = Increment(x=w835) -> (x+1=w642:i32)
                  n301 = Increment(x=w642) -> (x+1=w487:i32)
                  n302 = Add(x=w487, y=w486) -> (x+y=w484:i32)
                  n303 = Increment(x=w484) -> (x+1=w483:i32)
                  n304 = Index Array(array=w478, index=w891) -> (element=w1003:string)
                  n305 = Index Array(array=w478, index=w890) -> (element=w992:string)
                  n306 = Index Array(array=w478, index=w889) -> (element=w976:string)
                  n307 = Index Array(array=w478, index=w888) -> (element=w981:string)
                  n308 = Index Array(array=w478, index=w887) -> (element=w982:string)
                  n309 = Index Array(array=w478, index=w776) -> (element=w974:string)
                  n310 = Index Array(array=w478, index=w819) -> (element=w778:string)
                  n311 = Index Array(array=w478, index=w820) -> (element=w788:string)
                  n312 = Index Array(array=w478, index=w821) -> (element=w804:string)
                  n313 = Index Array(array=w478, index=w822) -> (element=w799:string)
                  n314 = Index Array(array=w478, index=w751) -> (element=w798:string)
                  n315 = Index Array(array=w478, index=w772) -> (element=w752:string)
                  n316 = Index Array(array=w478, index=w773) -> (element=w757:string)
                  n317 = Index Array(array=w478, index=w774) -> (element=w758:string)
                  n318 = Index Array(array=w478, index=w750) -> (element=w771:string)
                  n319 = Index Array(array=w478, index=w522) -> (element=w806:string)
                  n320 = for {
                    N: w511 -> [_]
                    tunnel: w512 -> [w1082]
                    tunnel: [w1081] -> w524 mode=indexing
                    i -> [w1083]
                    n321 = Add(x=w1082, y=w1083) -> (x+y=w1081:i32)
                  }
                  n322 = Index Array(array=w478, index=w510) -> (element=w857:string)
                  n323 = Index Array(array=w478, index=w498) -> (element=w862:string)
                  n324 = for {
                    N: w504 -> [_]
                    tunnel: w505 -> [w1070]
                    tunnel: [w1069] -> w509 mode=indexing
                    i -> [w1071]
                    n325 = Add(x=w1070, y=w1071) -> (x+y=w1069:i32)
                  }
                  n326 = for {
                    N: w496 -> [_]
                    tunnel: w497 -> [w1056]
                    tunnel: [w1055] -> w507 mode=indexing
                    i -> [w1057]
                    n327 = Add(x=w1056, y=w1057) -> (x+y=w1055:i32)
                  }
                  n328 = Index Array(array=w478, index=w495) -> (element=w960:string)
                  n329 = Index Array(array=w478, index=w835) -> (element=w952:string)
                  n330 = Index Array(array=w478, index=w642) -> (element=w840:string)
                  n331 = for {
                    N: w486 -> [_]
                    tunnel: w487 -> [w1227]
                    tunnel: [w1226] -> w644 mode=indexing
                    i -> [w1228]
                    n332 = Add(x=w1227, y=w1228) -> (x+y=w1226:i32)
                  }
                  n333 = Index Array(array=w478, index=w484) -> (element=w493:string)
                  n334 = call "2D array search.vi"("Search For"=w1003, "Input Array"=w485) -> ("Column"=w1002:i32, "Row"=w1000:i32)  [unwired: 7 in, 1 out]
                  n335 = call "2D array search.vi"("Search For"=w992, "Input Array"=w485) -> ("Column"=w993:i32, "Row"=w995:i32)  [unwired: 7 in, 1 out]
                  n336 = call "2D array search.vi"("Search For"=w976, "Input Array"=w485) -> ("Column"=w978:i32, "Row"=w980:i32)  [unwired: 7 in, 1 out]
                  n337 = call "2D array search.vi"("Search For"=w981, "Input Array"=w485) -> ("Column"=w985:i32, "Row"=w987:i32)  [unwired: 7 in, 1 out]
                  n338 = call "2D array search.vi"("Search For"=w982, "Input Array"=w485) -> ("Column"=w988:i32, "Row"=w990:i32)  [unwired: 7 in, 1 out]
                  n339 = call "2D array search.vi"("Search For"=w974, "Input Array"=w485) -> ("Column"=w973:i32, "Row"=w971:i32)  [unwired: 7 in, 1 out]
                  n340 = call "2D array search.vi"("Search For"=w778, "Input Array"=w485) -> ("Column"=w779:i32, "Row"=w781:i32)  [unwired: 7 in, 1 out]
                  n341 = call "2D array search.vi"("Search For"=w788, "Input Array"=w485) -> ("Column"=w787:i32, "Row"=w785:i32)  [unwired: 7 in, 1 out]
                  n342 = call "2D array search.vi"("Search For"=w804, "Input Array"=w485) -> ("Column"=w802:i32, "Row"=w800:i32)  [unwired: 7 in, 1 out]
                  n343 = call "2D array search.vi"("Search For"=w799, "Input Array"=w485) -> ("Column"=w795:i32, "Row"=w793:i32)  [unwired: 7 in, 1 out]
                  n344 = call "2D array search.vi"("Search For"=w798, "Input Array"=w485) -> ("Column"=w792:i32, "Row"=w790:i32)  [unwired: 7 in, 1 out]
                  n345 = call "2D array search.vi"("Search For"=w752, "Input Array"=w485) -> ("Column"=w754:i32, "Row"=w756:i32)  [unwired: 7 in, 1 out]
                  n346 = call "2D array search.vi"("Search For"=w757, "Input Array"=w485) -> ("Column"=w761:i32, "Row"=w763:i32)  [unwired: 7 in, 1 out]
                  n347 = call "2D array search.vi"("Search For"=w758, "Input Array"=w485) -> ("Column"=w764:i32, "Row"=w766:i32)  [unwired: 7 in, 1 out]
                  n348 = call "2D array search.vi"("Search For"=w771, "Input Array"=w485) -> ("Column"=w769:i32, "Row"=w767:i32)  [unwired: 7 in, 1 out]
                  n349 = call "2D array search.vi"("Search For"=w806, "Input Array"=w485) -> ("Column"=w807:i32, "Row"=w809:i32)  [unwired: 7 in, 1 out]
                  n350 = call "2D array search.vi"("Search For"=w857, "Input Array"=w485) -> ("Column"=w859:i32, "Row"=w861:i32)  [unwired: 7 in, 1 out]
                  n351 = call "2D array search.vi"("Search For"=w862, "Input Array"=w485) -> ("Column"=w864:i32, "Row"=w866:i32)  [unwired: 7 in, 1 out]
                  n352 = call "2D array search.vi"("Search For"=w960, "Input Array"=w485) -> ("Column"=w959:i32, "Row"=w957:i32)  [unwired: 7 in, 1 out]
                  n353 = call "2D array search.vi"("Search For"=w952, "Input Array"=w485) -> ("Column"=w953:i32, "Row"=w955:i32)  [unwired: 7 in, 1 out]
                  n354 = call "2D array search.vi"("Search For"=w840, "Input Array"=w485) -> ("Column"=w839:i32, "Row"=w837:i32)  [unwired: 7 in, 1 out]
                  n355 = call "2D array search.vi"("Search For"=w493, "Input Array"=w485) -> ("Column"=w492:i32, "Row"=w490:i32)  [unwired: 7 in, 1 out]
                  n356 = for {
                    tunnel: w478 -> [w1091]
                    tunnel: w485 -> [w1090]
                    tunnel: w524 -> [w1088] mode=indexing
                    tunnel: [w1086] -> w523 mode=indexing
                    n357 = Index Array(array=w1091, index=w1088) -> (element=w1089:string)
                    n358 = call "2D array search.vi"("Alternative"="Y" ("Option for alternative"), "Option for alternative"="Z", "Search For"=w1089, "Input Array"=w1090) -> ("Column"=w1094:i32, "Row"=w1092:i32)  [unwired: 5 in, 1 out]
                    n359 = Increment(x=w1094) -> (x+1=w1093:i32)
                    n360 = Index Array(array=w1090, index (row)=w1092, index (col)=w1093) -> (element=w1087:string)
                    n361 = Fract/Exp String To Number(string=w1087) -> (number=w1086:dbl)  [unwired: 4 out]
                  }
                  n362 = for {
                    tunnel: w478 -> [w1077]
                    tunnel: w485 -> [w1076]
                    tunnel: w509 -> [w1074] mode=indexing
                    tunnel: [w1072] -> w506 mode=indexing
                    n363 = Index Array(array=w1077, index=w1074) -> (element=w1075:string)
                    n364 = call "2D array search.vi"("Search For"=w1075, "Input Array"=w1076) -> ("Column"=w1080:i32, "Row"=w1078:i32)  [unwired: 7 in, 1 out]
                    n365 = Increment(x=w1080) -> (x+1=w1079:i32)
                    n366 = Index Array(array=w1076, index (row)=w1078, index (col)=w1079) -> (element=w1073:string)
                    n367 = Fract/Exp String To Number(string=w1073) -> (number=w1072:dbl)  [unwired: 4 out]
                  }
                  n368 = for {
                    tunnel: w478 -> [w1065]
                    tunnel: w485 -> [w1064]
                    tunnel: w507 -> [w1062] mode=indexing
                    tunnel: [w1058] -> w508 mode=indexing
                    n369 = Index Array(array=w1065, index=w1062) -> (element=w1063:string)
                    n370 = call "2D array search.vi"("Search For"=w1063, "Input Array"=w1064) -> ("Column"=w1068:i32, "Row"=w1066:i32)  [unwired: 7 in, 1 out]
                    n371 = Increment(x=w1068) -> (x+1=w1067:i32)
                    n372 = Index Array(array=w1064, index (row)=w1066, index (col)=w1067) -> (element=w1059:string)
                    n373 = Match True/False String(2:"FALSE" ("true string"), 3:"TRUE" ("true string"), 4:w1059) -> (0:w1058:bool)  [unwired: 1 out]
                  }
                  n374 = for {
                    tunnel: w478 -> [w1234]
                    tunnel: w485 -> [w1233]
                    tunnel: w644 -> [w1231] mode=indexing
                    tunnel: [w1229] -> w643 mode=indexing
                    n375 = Index Array(array=w1234, index=w1231) -> (element=w1232:string)
                    n376 = call "2D array search.vi"("Search For"=w1232, "Input Array"=w1233) -> ("Column"=w1237:i32, "Row"=w1235:i32)  [unwired: 7 in, 1 out]
                    n377 = Increment(x=w1237) -> (x+1=w1236:i32)
                    n378 = Index Array(array=w1233, index (row)=w1235, index (col)=w1236) -> (element=w1230:string)
                    n379 = Fract/Exp String To Number(string=w1230) -> (number=w1229:dbl)  [unwired: 4 out]
                  }
                  n380 = Increment(x=w1002) -> (x+1=w1001:i32)
                  n381 = Increment(x=w993) -> (x+1=w994:i32)
                  n382 = Increment(x=w978) -> (x+1=w979:i32)
                  n383 = Increment(x=w985) -> (x+1=w986:i32)
                  n384 = Increment(x=w988) -> (x+1=w989:i32)
                  n385 = Increment(x=w973) -> (x+1=w972:i32)
                  n386 = Increment(x=w779) -> (x+1=w780:i32)
                  n387 = Increment(x=w787) -> (x+1=w786:i32)
                  n388 = Increment(x=w802) -> (x+1=w801:i32)
                  n389 = Increment(x=w795) -> (x+1=w794:i32)
                  n390 = Increment(x=w792) -> (x+1=w791:i32)
                  n391 = Increment(x=w754) -> (x+1=w755:i32)
                  n392 = Increment(x=w761) -> (x+1=w762:i32)
                  n393 = Increment(x=w764) -> (x+1=w765:i32)
                  n394 = Increment(x=w769) -> (x+1=w768:i32)
                  n395 = Increment(x=w807) -> (x+1=w808:i32)
                  n396 = Increment(x=w859) -> (x+1=w860:i32)
                  n397 = Increment(x=w864) -> (x+1=w865:i32)
                  n398 = Increment(x=w959) -> (x+1=w958:i32)
                  n399 = Increment(x=w953) -> (x+1=w954:i32)
                  n400 = Increment(x=w839) -> (x+1=w838:i32)
                  n401 = Increment(x=w492) -> (x+1=w491:i32)
                  n402 = Index Array(array=w485, index (row)=w1000, index (col)=w1001) -> (element=w999:string)
                  n403 = Index Array(array=w485, index (row)=w995, index (col)=w994) -> (element=w996:string)
                  n404 = Index Array(array=w485, index (row)=w980, index (col)=w979) -> (element=w977:string)
                  n405 = Index Array(array=w485, index (row)=w987, index (col)=w986) -> (element=w984:string)
                  n406 = Index Array(array=w485, index (row)=w990, index (col)=w989) -> (element=w983:string)
                  n407 = Index Array(array=w485, index (row)=w971, index (col)=w972) -> (element=w970:string)
                  n408 = Index Array(array=w485, index (row)=w781, index (col)=w780) -> (element=w744:string)
                  n409 = Index Array(array=w485, index (row)=w785, index (col)=w786) -> (element=w784:string)
                  n410 = Index Array(array=w485, index (row)=w800, index (col)=w801) -> (element=w803:string)
                  n411 = Index Array(array=w485, index (row)=w793, index (col)=w794) -> (element=w796:string)
                  n412 = Index Array(array=w485, index (row)=w790, index (col)=w791) -> (element=w797:string)
                  n413 = Index Array(array=w485, index (row)=w756, index (col)=w755) -> (element=w753:string)
                  n414 = Index Array(array=w485, index (row)=w763, index (col)=w762) -> (element=w760:string)
                  n415 = Index Array(array=w485, index (row)=w766, index (col)=w765) -> (element=w759:string)
                  n416 = Index Array(array=w485, index (row)=w767, index (col)=w768) -> (element=w770:string)
                  n417 = Index Array(array=w485, index (row)=w809, index (col)=w808) -> (element=w810:string)
                  n418 = Index Array(array=w485, index (row)=w861, index (col)=w860) -> (element=w858:string)
                  n419 = Index Array(array=w485, index (row)=w866, index (col)=w865) -> (element=w863:string)
                  n420 = Index Array(array=w485, index (row)=w957, index (col)=w958) -> (element=w946:string)
                  n421 = Index Array(array=w485, index (row)=w955, index (col)=w954) -> (element=w945:string)
                  n422 = Index Array(array=w485, index (row)=w837, index (col)=w838) -> (element=w842:string)
                  n423 = Index Array(array=w485, index (row)=w490, index (col)=w491) -> (element=w489:string)
                  n424 = Match True/False String(2:"FALSE" ("true string"), 3:"TRUE" ("true string"), 4:w999) -> (0:w967:bool)  [unwired: 1 out]
                  n425 = Match True/False String(2:"FALSE" ("true string"), 3:"TRUE" ("true string"), 4:w996) -> (0:w966:bool)  [unwired: 1 out]
                  n426 = Fract/Exp String To Number(string=w977) -> (number=w965:dbl)  [unwired: 4 out]
                  n427 = Fract/Exp String To Number(string=w984) -> (number=w964:dbl)  [unwired: 4 out]
                  n428 = Fract/Exp String To Number(string=w983) -> (number=w962:dbl)  [unwired: 4 out]
                  n429 = Match True/False String(2:"FALSE" ("true string"), 3:"TRUE" ("true string"), 4:w970) -> (0:w963:bool)  [unwired: 1 out]
                  n430 = Match True/False String(2:"FALSE" ("true string"), 3:"TRUE" ("true string"), 4:w744) -> (0:w813:bool)  [unwired: 1 out]
                  n431 = Match True/False String(2:"FALSE" ("true string"), 3:"TRUE" ("true string"), 4:w784) -> (0:w814:bool)  [unwired: 1 out]
                  n432 = Fract/Exp String To Number(string=w803) -> (number=w815:dbl)  [unwired: 4 out]
                  n433 = Fract/Exp String To Number(string=w796) -> (number=w816:dbl)  [unwired: 4 out]
                  n434 = Fract/Exp String To Number(string=w797) -> (number=w817:dbl)  [unwired: 4 out]
                  n435 = Fract/Exp String To Number(string=w753) -> (number=w749:dbl)  [unwired: 4 out]
                  n436 = Fract/Exp String To Number(string=w760) -> (number=w748:dbl)  [unwired: 4 out]
                  n437 = Fract/Exp String To Number(string=w759) -> (number=w747:dbl)  [unwired: 4 out]
                  n438 = Fract/Exp String To Number(string=w770) -> (number=w746:dbl)  [unwired: 4 out]
                  n439 = Match True/False String(2:"FALSE" ("true string"), 3:"TRUE" ("true string"), 4:w810) -> (0:w775:bool)  [unwired: 1 out]
                  n440 = Fract/Exp String To Number(string=w858) -> (number=w855:dbl)  [unwired: 4 out]
                  n441 = Fract/Exp String To Number(string=w863) -> (number=w852:dbl)  [unwired: 4 out]
                  n442 = Fract/Exp String To Number(string=w946) -> (number=w948:dbl)  [unwired: 4 out]
                  n443 = Match True/False String(2:"FALSE" ("true string"), 3:"TRUE" ("true string"), 4:w945) -> (0:w947:bool)  [unwired: 1 out]
                  n444 = Match True/False String(2:"FALSE" ("true string"), 3:"TRUE" ("true string"), 4:w842) -> (0:w834:bool)  [unwired: 1 out]
                  n445 = Match True/False String(2:"FALSE" ("true string"), 3:"TRUE" ("true string"), 4:w489) -> (0:w482:bool)  [unwired: 1 out]
                  n446 = Equal To 0?(x=w855) -> (x = 0?=w856:bool)
                  n447 = Equal To 0?(x=w852) -> (x = 0?=w853:bool)
                  n448 = Select(t=w851, s=w856, f=w855) -> (s? t:f=w854:dbl)
                  n449 = Select(t=w851, s=w853, f=w852) -> (s? t:f=w850:dbl)
                  n450 = local read "Read output"() -> (w961:T1)
                  n451 = Unbundle By Name(w961) -> ("Low mag SEM"=w968:T11)
                  n452 = Bundle By Name(cluster=w968, "Low mag scan"=w967, "Prior to main scan"=w966, "Low mag interval"=w965, "Low mag scan FOV (micron)"=w964, "Low mag scan rate (Hz)"=w962, "Show HM box"=w963) -> (w944:T11)
                  n453 = local read "Read output"() -> (w818:T1)
                  n454 = Unbundle By Name(w818) -> ("Mid Mag SEM"=w812:T12)
                  n455 = Bundle By Name(cluster=w812, "Mid mag scan"=w813, "Prior to main scan"=w814, "Mid mag interval"=w815, "X size (um)"=w816, "Y size (um)"=w817, "X center (um)"=w749, "Y center (um)"=w748, "Mid mag scan rate (Hz)"=w747, "Pixel size (nm)"=w746, "Show MM box"=w775) -> (w745:T12)
                  n456 = Index Array(array=w523) -> (element #1=w521:dbl, element #2=w520:dbl, element #3=w519:dbl, element #4=w518:dbl, element #5=w517:dbl, element #6=w516:dbl, element #7=w515:dbl, element #8=w514:dbl, element #9=w513:dbl)  [unwired: 9 in]
                  n457 = Index Array(array=w506) -> (element #1=w501:dbl, element #2=w500:dbl, element #3=w499:dbl)  [unwired: 3 in]
                  n458 = Index Array(array=w508) -> (element #1=w503:bool, element #2=w502:bool)  [unwired: 2 in]
                  n459 = Index Array(array=w643) -> (element #1=w641:dbl, element #2=w640:dbl, element #3=w639:dbl, element #4=w638:dbl, element #5=w637:dbl, element #6=w636:dbl, element #7=w527:dbl, element #8=w526:dbl)  [unwired: 8 in]
                  n460 = local read "Read output"() -> (w950:T1)
                  n461 = Unbundle By Name(w950) -> ("Milling para"=w949:T28)
                  n462 = Bundle By Name(cluster=w949, "X resolution"=w520, "Z resolution"=w519, "X offset (um)"=w518, "Z offset (um)"=w517, "X center (um)"=w516, "Z center (um)"=w515, "X size (um)"=w514, "Z size (um)"=w513, "UL-Ang"=w854, "UR-Ang"=w850, "Line milling time (s)"=w501, "Z-step (nm)"=w500, "Lines auto pause"=w499, "Auto pause"=w503, "Mill from Bottom"=w502, "FIB FOV (um)"=w948, "Auto Profile"=w947, "FIB PID on"=w834, "FIB PID measured"=w641, "FIB PID target"=w640, "FIB PID target slope"=w639, "FIB PID P"=w638, "FIB PID I"=w637, "FIB PID D"=w636, "Emission (uA)"=w527, "Suppressor (V)"=w526, "Auto reheat"=w482) -> (w943:T28)
                  n463 = Increment(x=w483) -> (x+1=w740:i32)
                  n464 = Increment(x=w740) -> (x+1=w480:i32)
                  n465 = Add(x=w480, y=w479) -> (x+y=w886:i32)
                  n466 = Increment(x=w886) -> (x+1=w885:i32)
                  n467 = Increment(x=w885) -> (x+1=w721:i32)
                  n468 = Increment(x=w721) -> (x+1=w710:i32)
                  n469 = Add(x=w710, y=w709) -> (x+y=w708:i32)
                  n470 = Add(x=w708, y=w707) -> (x+y=w535:i32)
                  n471 = Add(x=w535, y=w534) -> (x+y=w540:i32)
                  n472 = Add(x=w540, y=w541) -> (x+y=w533:i32)
                  n473 = Add(x=w533, y=w532) -> (x+y=w702:i32)
                  n474 = Add(x=w702, y=w701) -> (x+y=w694:i32)
                  n475 = Increment(x=w694) -> (x+1=w699:i32)
                  n476 = Add(x=w699, y=w700) -> (x+y=w632:i32)
                  n477 = Add(x=w632, y=w633) -> (x+y=w630:i32)
                  n478 = Add(x=w630, y=w631) -> (x+y=w629:i32)
                  n479 = Add(x=w629, y=w683) -> (x+y=w666:i32)
                  n480 = Add(x=w666, y=w665) -> (x+y=w667:i32)
                  n481 = Increment(x=w667) -> (x+1=w668:i32)
                  n482 = Increment(x=w668) -> (x+1=w649:i32)
                  n483 = Add(x=w649, y=w648) -> (x+y=w655:i32)
                  n484 = Index Array(array=w478, index=w483) -> (element=w935:string)
                  n485 = Index Array(array=w478, index=w740) -> (element=w941:string)
                  n486 = for {
                    N: w479 -> [_]
                    tunnel: w480 -> [w1359]
                    tunnel: [w1358] -> w741 mode=indexing
                    i -> [w1360]
                    n487 = Add(x=w1359, y=w1360) -> (x+y=w1358:i32)
                  }
                  n488 = Index Array(array=w478, index=w886) -> (element=w919:string)
                  n489 = Index Array(array=w478, index=w885) -> (element=w913:string)
                  n490 = Index Array(array=w478, index=w721) -> (element=w909:string)
                  n491 = for {
                    N: w709 -> [_]
                    tunnel: w710 -> [w1345]
                    tunnel: [w1344] -> w722 mode=indexing
                    i -> [w1346]
                    n492 = Add(x=w1345, y=w1346) -> (x+y=w1344:i32)
                  }
                  n493 = for {
                    N: w707 -> [_]
                    tunnel: w708 -> [w1333]
                    tunnel: [w1332] -> w719 mode=indexing
                    i -> [w1334]
                    n494 = Add(x=w1333, y=w1334) -> (x+y=w1332:i32)
                  }
                  n495 = for {
                    N: w534 -> [_]
                    tunnel: w535 -> [w1317]
                    tunnel: [w1316] -> w717 mode=indexing
                    i -> [w1318]
                    n496 = Add(x=w1317, y=w1318) -> (x+y=w1316:i32)
                  }
                  n497 = for {
                    N: w541 -> [_]
                    tunnel: w540 -> [w1110]
                    tunnel: [w1109] -> w536 mode=indexing
                    i -> [w1111]
                    n498 = Add(x=w1110, y=w1111) -> (x+y=w1109:i32)
                  }
                  n499 = for {
                    N: w532 -> [_]
                    tunnel: w533 -> [w1096]
                    tunnel: [w1095] -> w538 mode=indexing
                    i -> [w1097]
                    n500 = Add(x=w1096, y=w1097) -> (x+y=w1095:i32)
                  }
                  n501 = for {
                    N: w701 -> [_]
                    tunnel: w702 -> [w1305]
                    tunnel: [w1304] -> w716 mode=indexing
                    i -> [w1306]
                    n502 = Add(x=w1305, y=w1306) -> (x+y=w1304:i32)
                  }
                  n503 = Index Array(array=w478, index=w694) -> (element=w825:string)
                  n504 = for {
                    N: w700 -> [_]
                    tunnel: w699 -> [w1293]
                    tunnel: [w1292] -> w695 mode=indexing
                    i -> [w1294]
                    n505 = Add(x=w1293, y=w1294) -> (x+y=w1292:i32)
                  }
                  n506 = for {
                    N: w633 -> [_]
                    tunnel: w632 -> [w1279]
                    tunnel: [w1278] -> w697 mode=indexing
                    i -> [w1280]
                    n507 = Add(x=w1279, y=w1280) -> (x+y=w1278:i32)
                  }
                  n508 = for {
                    N: w631 -> [_]
                    tunnel: w630 -> [w1215]
                    tunnel: [w1214] -> w635 mode=indexing
                    i -> [w1216]
                    n509 = Add(x=w1215, y=w1216) -> (x+y=w1214:i32)
                  }
                  n510 = for {
                    N: w683 -> [_]
                    tunnel: w629 -> [w1265]
                    tunnel: [w1264] -> w688 mode=indexing
                    i -> [w1266]
                    n511 = Add(x=w1265, y=w1266) -> (x+y=w1264:i32)
                  }
                  n512 = for {
                    N: w665 -> [_]
                    tunnel: w666 -> [w1253]
                    tunnel: [w1252] -> w684 mode=indexing
                    i -> [w1254]
                    n513 = Add(x=w1253, y=w1254) -> (x+y=w1252:i32)
                  }
                  n514 = Index Array(array=w478, index=w667) -> (element=w681:string)
                  n515 = Index Array(array=w478, index=w668) -> (element=w674:string)
                  n516 = for {
                    N: w648 -> [_]
                    tunnel: w649 -> [w1239]
                    tunnel: [w1238] -> w670 mode=indexing
                    i -> [w1240]
                    n517 = Add(x=w1239, y=w1240) -> (x+y=w1238:i32)
                  }
                  n518 = Index Array(array=w478, index=w655) -> (element=w651:string)
                  n519 = call "2D array search.vi"("Search For"=w935, "Input Array"=w485) -> ("Column"=w931:i32, "Row"=w933:i32)  [unwired: 7 in, 1 out]
                  n520 = call "2D array search.vi"("Search For"=w941, "Input Array"=w485) -> ("Column"=w940:i32, "Row"=w938:i32)  [unwired: 7 in, 1 out]
                  n521 = call "2D array search.vi"("Search For"=w919, "Input Array"=w485) -> ("Column"=w917:i32, "Row"=w915:i32)  [unwired: 7 in, 1 out]
                  n522 = call "2D array search.vi"("Search For"=w913, "Input Array"=w485) -> ("Column"=w910:i32, "Row"=w912:i32)  [unwired: 7 in, 1 out]
                  n523 = call "2D array search.vi"("Search For"=w909, "Input Array"=w485) -> ("Column"=w906:i32, "Row"=w907:i32)  [unwired: 7 in, 1 out]
                  n524 = call "2D array search.vi"("Search For"=w825, "Input Array"=w485) -> ("Column"=w826:i32, "Row"=w828:i32)  [unwired: 7 in, 1 out]
                  n525 = call "2D array search.vi"("Search For"=w681, "Input Array"=w485) -> ("Column"=w680:i32, "Row"=w678:i32)  [unwired: 7 in, 1 out]
                  n526 = call "2D array search.vi"("Search For"=w674, "Input Array"=w485) -> ("Column"=w673:i32, "Row"=w671:i32)  [unwired: 7 in, 1 out]
                  n527 = call "2D array search.vi"("Search For"=w651, "Input Array"=w485) -> ("Column"=w652:i32, "Row"=w654:i32)  [unwired: 7 in, 1 out]
                  n528 = for {
                    tunnel: w478 -> [w1366]
                    tunnel: w485 -> [w1365]
                    tunnel: w741 -> [w1363] mode=indexing
                    tunnel: [w1361] -> w739 mode=indexing
                    n529 = Index Array(array=w1366, index=w1363) -> (element=w1364:string)
                    n530 = call "2D array search.vi"("Search For"=w1364, "Input Array"=w1365) -> ("Column"=w1369:i32, "Row"=w1367:i32)  [unwired: 7 in, 1 out]
                    n531 = Increment(x=w1369) -> (x+1=w1368:i32)
                    n532 = Index Array(array=w1365, index (row)=w1367, index (col)=w1368) -> (element=w1362:string)
                    n533 = Fract/Exp String To Number(string=w1362) -> (number=w1361:dbl)  [unwired: 4 out]
                  }
                  n534 = for {
                    tunnel: w478 -> [w1354]
                    tunnel: w485 -> [w1353]
                    tunnel: w722 -> [w1351] mode=indexing
                    tunnel: [w1347] -> w720 mode=indexing
                    n535 = Index Array(array=w1354, index=w1351) -> (element=w1352:string)
                    n536 = call "2D array search.vi"("Search For"=w1352, "Input Array"=w1353) -> ("Column"=w1357:i32, "Row"=w1355:i32)  [unwired: 7 in, 1 out]
                    n537 = Increment(x=w1357) -> (x+1=w1356:i32)
                    n538 = Index Array(array=w1353, index (row)=w1355, index (col)=w1356) -> (element=w1348:string)
                    n539 = Match True/False String(2:"FALSE" ("true string"), 3:"TRUE" ("true string"), 4:w1348) -> (0:w1347:bool)  [unwired: 1 out]
                  }
                  n540 = for {
                    tunnel: w478 -> [w1340]
                    tunnel: w485 -> [w1339]
                    tunnel: w719 -> [w1337] mode=indexing
                    tunnel: [w1335] -> w713 mode=indexing
                    n541 = Index Array(array=w1340, index=w1337) -> (element=w1338:string)
                    n542 = call "2D array search.vi"("Search For"=w1338, "Input Array"=w1339) -> ("Column"=w1343:i32, "Row"=w1341:i32)  [unwired: 7 in, 1 out]
                    n543 = Increment(x=w1343) -> (x+1=w1342:i32)
                    n544 = Index Array(array=w1339, index (row)=w1341, index (col)=w1342) -> (element=w1336:string)
                    n545 = Fract/Exp String To Number(string=w1336) -> (number=w1335:dbl)  [unwired: 4 out]
                  }
                  n546 = for {
                    tunnel: w478 -> [w1328]
                    tunnel: w485 -> [w1327]
                    tunnel: w717 -> [w1325] mode=indexing
                    tunnel: [w1321] -> w718 mode=indexing
                    n547 = Index Array(array=w1328, index=w1325) -> (element=w1326:string)
                    n548 = call "2D array search.vi"("Alternative"="Y" ("Option for alternative"), "Option for alternative"="Z", "Search For"=w1326, "Input Array"=w1327) -> ("Column"=w1331:i32, "Row"=w1329:i32)  [unwired: 5 in, 1 out]
                    n549 = Increment(x=w1331) -> (x+1=w1330:i32)
                    n550 = Index Array(array=w1327, index (row)=w1329, index (col)=w1330) -> (element=w1322:string)
                    n551 = Match True/False String(2:"FALSE" ("true string"), 3:"TRUE" ("true string"), 4:w1322) -> (0:w1321:bool)  [unwired: 1 out]
                  }
                  n552 = for {
                    tunnel: w478 -> [w1117]
                    tunnel: w485 -> [w1116]
                    tunnel: w536 -> [w1114] mode=indexing
                    tunnel: [w1112] -> w539 mode=indexing
                    n553 = Index Array(array=w1117, index=w1114) -> (element=w1115:string)
                    n554 = call "2D array search.vi"("Search For"=w1115, "Input Array"=w1116) -> ("Column"=w1120:i32, "Row"=w1118:i32)  [unwired: 7 in, 1 out]
                    n555 = Increment(x=w1120) -> (x+1=w1119:i32)
                    n556 = Index Array(array=w1116, index (row)=w1118, index (col)=w1119) -> (element=w1113:string)
                    n557 = Fract/Exp String To Number(string=w1113) -> (number=w1112:dbl)  [unwired: 4 out]
                  }
                  n558 = for {
                    tunnel: w478 -> [w1105]
                    tunnel: w485 -> [w1104]
                    tunnel: w538 -> [w1102] mode=indexing
                    tunnel: [w1098] -> w537 mode=indexing
                    n559 = Index Array(array=w1105, index=w1102) -> (element=w1103:string)
                    n560 = call "2D array search.vi"("Search For"=w1103, "Input Array"=w1104) -> ("Column"=w1108:i32, "Row"=w1106:i32)  [unwired: 7 in, 1 out]
                    n561 = Increment(x=w1108) -> (x+1=w1107:i32)
                    n562 = Index Array(array=w1104, index (row)=w1106, index (col)=w1107) -> (element=w1099:string)
                    n563 = Match True/False String(2:"FALSE" ("true string"), 3:"TRUE" ("true string"), 4:w1099) -> (0:w1098:bool)  [unwired: 1 out]
                  }
                  n564 = for {
                    tunnel: w478 -> [w1312]
                    tunnel: w485 -> [w1311]
                    tunnel: w716 -> [w1309] mode=indexing
                    tunnel: [w1307] -> w705 mode=indexing
                    n565 = Index Array(array=w1312, index=w1309) -> (element=w1310:string)
                    n566 = call "2D array search.vi"("Search For"=w1310, "Input Array"=w1311) -> ("Column"=w1315:i32, "Row"=w1313:i32)  [unwired: 7 in, 1 out]
                    n567 = Increment(x=w1315) -> (x+1=w1314:i32)
                    n568 = Index Array(array=w1311, index (row)=w1313, index (col)=w1314) -> (element=w1308:string)
                    n569 = Fract/Exp String To Number(string=w1308) -> (number=w1307:dbl)  [unwired: 4 out]
                  }
                  n570 = for {
                    tunnel: w478 -> [w1300]
                    tunnel: w485 -> [w1299]
                    tunnel: w695 -> [w1297] mode=indexing
                    tunnel: [w1295] -> w698 mode=indexing
                    n571 = Index Array(array=w1300, index=w1297) -> (element=w1298:string)
                    n572 = call "2D array search.vi"("Search For"=w1298, "Input Array"=w1299) -> ("Column"=w1303:i32, "Row"=w1301:i32)  [unwired: 7 in, 1 out]
                    n573 = Increment(x=w1303) -> (x+1=w1302:i32)
                    n574 = Index Array(array=w1299, index (row)=w1301, index (col)=w1302) -> (element=w1296:string)
                    n575 = Fract/Exp String To Number(string=w1296) -> (number=w1295:dbl)  [unwired: 4 out]
                  }
                  n576 = for {
                    tunnel: w478 -> [w1288]
                    tunnel: w485 -> [w1287]
                    tunnel: w697 -> [w1285] mode=indexing
                    tunnel: [w1281] -> w696 mode=indexing
                    n577 = Index Array(array=w1288, index=w1285) -> (element=w1286:string)
                    n578 = call "2D array search.vi"("Search For"=w1286, "Input Array"=w1287) -> ("Column"=w1291:i32, "Row"=w1289:i32)  [unwired: 7 in, 1 out]
                    n579 = Increment(x=w1291) -> (x+1=w1290:i32)
                    n580 = Index Array(array=w1287, index (row)=w1289, index (col)=w1290) -> (element=w1282:string)
                    n581 = Match True/False String(2:"FALSE" ("true string"), 3:"TRUE" ("true string"), 4:w1282) -> (0:w1281:bool)  [unwired: 1 out]
                  }
                  n582 = for {
                    tunnel: w478 -> [w1222]
                    tunnel: w485 -> [w1221]
                    tunnel: w635 -> [w1219] mode=indexing
                    tunnel: [w1217] -> w634 mode=indexing
                    n583 = Index Array(array=w1222, index=w1219) -> (element=w1220:string)
                    n584 = call "2D array search.vi"("Search For"=w1220, "Input Array"=w1221) -> ("Column"=w1225:i32, "Row"=w1223:i32)  [unwired: 7 in, 1 out]
                    n585 = Increment(x=w1225) -> (x+1=w1224:i32)
                    n586 = Index Array(array=w1221, index (row)=w1223, index (col)=w1224) -> (element=w1218:string)
                    n587 = Fract/Exp String To Number(string=w1218) -> (number=w1217:dbl)  [unwired: 4 out]
                  }
                  n588 = for {
                    tunnel: w478 -> [w1274]
                    tunnel: w485 -> [w1273]
                    tunnel: w688 -> [w1271] mode=indexing
                    tunnel: [w1267] -> w689 mode=indexing
                    n589 = Index Array(array=w1274, index=w1271) -> (element=w1272:string)
                    n590 = call "2D array search.vi"("Search For"=w1272, "Input Array"=w1273) -> ("Column"=w1277:i32, "Row"=w1275:i32)  [unwired: 7 in, 1 out]
                    n591 = Increment(x=w1277) -> (x+1=w1276:i32)
                    n592 = Index Array(array=w1273, index (row)=w1275, index (col)=w1276) -> (element=w1268:string)
                    n593 = Match True/False String(2:"FALSE" ("true string"), 3:"TRUE" ("true string"), 4:w1268) -> (0:w1267:bool)  [unwired: 1 out]
                  }
                  n594 = for {
                    tunnel: w478 -> [w1260]
                    tunnel: w485 -> [w1259]
                    tunnel: w684 -> [w1257] mode=indexing
                    tunnel: [w1255] -> w685 mode=indexing
                    n595 = Index Array(array=w1260, index=w1257) -> (element=w1258:string)
                    n596 = call "2D array search.vi"("Search For"=w1258, "Input Array"=w1259) -> ("Column"=w1263:i32, "Row"=w1261:i32)  [unwired: 7 in, 1 out]
                    n597 = Increment(x=w1263) -> (x+1=w1262:i32)
                    n598 = Index Array(array=w1259, index (row)=w1261, index (col)=w1262) -> (element=w1256:string)
                    n599 = Fract/Exp String To Number(string=w1256) -> (number=w1255:dbl)  [unwired: 4 out]
                  }
                  n600 = for {
                    tunnel: w478 -> [w1248]
                    tunnel: w485 -> [w1247]
                    tunnel: w670 -> [w1245] mode=indexing
                    tunnel: [w1241] -> w669 mode=indexing
                    n601 = Index Array(array=w1248, index=w1245) -> (element=w1246:string)
                    n602 = call "2D array search.vi"("Search For"=w1246, "Input Array"=w1247) -> ("Column"=w1251:i32, "Row"=w1249:i32)  [unwired: 7 in, 1 out]
                    n603 = Increment(x=w1251) -> (x+1=w1250:i32)
                    n604 = Index Array(array=w1247, index (row)=w1249, index (col)=w1250) -> (element=w1242:string)
                    n605 = Match True/False String(2:"FALSE" ("true string"), 3:"TRUE" ("true string"), 4:w1242) -> (0:w1241:bool)  [unwired: 1 out]
                  }
                  n606 = Increment(x=w931) -> (x+1=w932:i32)
                  n607 = Increment(x=w940) -> (x+1=w939:i32)
                  n608 = Increment(x=w917) -> (x+1=w916:i32)
                  n609 = Increment(x=w910) -> (x+1=w911:i32)
                  n610 = Increment(x=w826) -> (x+1=w827:i32)
                  n611 = Increment(x=w680) -> (x+1=w679:i32)
                  n612 = Increment(x=w673) -> (x+1=w672:i32)
                  n613 = Increment(x=w652) -> (x+1=w653:i32)
                  n614 = Index Array(array=w485, index (row)=w933, index (col)=w932) -> (element=w934:string)
                  n615 = Index Array(array=w485, index (row)=w938, index (col)=w939) -> (element=w937:string)
                  n616 = Index Array(array=w485, index (row)=w915, index (col)=w916) -> (element=w918:string)
                  n617 = Index Array(array=w485, index (row)=w912, index (col)=w911) -> (element=w908:string)
                  n618 = while {
                    tunnel: w907 -> [w1373]
                    tunnel: w906 -> [w1380]
                    tunnel: [w1376] -> w905 mode=indexing
                    tunnel: w485 -> [w1374]
                    i -> [w1378]
                    stop <- w1375 stop-if-true
                    n619 = Increment(x=w1380) -> (x+1=w1379:i32)
                    n620 = Add(x=w1379, y=w1378) -> (x+y=w1372:i32)
                    n621 = Increment(x=w1372) -> (x+1=w1371:i32)
                    n622 = Index Array(array=w1374, index (row)=w1373, index (col)=w1372) -> (element=w1376:string)
                    n623 = Index Array(array=w1374, index (row)=w1373, index (col)=w1371) -> (element=w1370:string)
                    n624 = Equal?(x=w1370, y="") -> (x = y?=w1375:bool)
                  }
                  n625 = Index Array(array=w485, index (row)=w828, index (col)=w827) -> (element=w829:string)
                  n626 = Index Array(array=w485, index (row)=w678, index (col)=w679) -> (element=w677:string)
                  n627 = Index Array(array=w485, index (row)=w671, index (col)=w672) -> (element=w675:string)
                  n628 = Index Array(array=w485, index (row)=w654, index (col)=w653) -> (element=w650:string)
                  n629 = Fract/Exp String To Number(string=w934) -> (number=w930:dbl)  [unwired: 4 out]
                  n630 = Match True/False String(2:"FALSE" ("true string"), 3:"TRUE" ("true string"), 4:w937) -> (0:w929:bool)  [unwired: 1 out]
                  n631 = Fract/Exp String To Number(string=w918) -> (number=w914:dbl)  [unwired: 4 out]
                  n632 = Match True/False String(2:"FALSE" ("true string"), 3:"TRUE" ("true string"), 4:w829) -> (0:w823:bool)  [unwired: 1 out]
                  n633 = Match True/False String(2:"FALSE" ("true string"), 3:"TRUE" ("true string"), 4:w677) -> (0:w659:bool)  [unwired: 1 out]
                  n634 = Fract/Exp String To Number(string=w675) -> (number=w658:dbl)  [unwired: 4 out]
                  n635 = Fract/Exp String To Number(string=w650) -> (number=w645:dbl)  [unwired: 4 out]
                  n636 = Index Array(array=w720) -> (element #1=w715:bool, element #2=w714:bool)  [unwired: 2 in]
                  n637 = Index Array(array=w713) -> (element #1=w712:dbl, element #2=w711:dbl)  [unwired: 2 in]
                  n638 = Index Array(array=w718) -> (element #1=w603:bool, element #2=w706:bool, element #3=w563:bool, element #4=w562:bool, element #5=w561:bool, element #6=w560:bool, element #7=w542:bool)  [unwired: 7 in]
                  n639 = Index Array(array=w539) -> (element #1=w531:dbl, element #2=w530:dbl)  [unwired: 2 in]
                  n640 = Index Array(array=w537) -> (element #1=w529:bool, element #2=w528:bool)  [unwired: 2 in]
                  n641 = Index Array(array=w705) -> (element #1=w704:dbl, element #2=w703:dbl)  [unwired: 2 in]
                  n642 = Index Array(array=w698) -> (element #1=w693:dbl, element #2=w692:dbl)  [unwired: 2 in]
                  n643 = Index Array(array=w696) -> (element #1=w691:bool, element #2=w690:bool)  [unwired: 2 in]
                  n644 = Index Array(array=w634) -> (element #1=w628:dbl, element #2=w627:dbl)  [unwired: 2 in]
                  n645 = Index Array(array=w689) -> (element #1=w687:bool, element #2=w686:bool, element #3=w626:bool)  [unwired: 3 in]
                  n646 = local read "Read output"() -> (w664:T1)
                  n647 = Index Array(array=w685) -> (element #1=w662:dbl, element #2=w661:dbl, element #3=w660:dbl)  [unwired: 3 in]
                  n648 = Index Array(array=w669) -> (element #1=w657:bool, element #2=w656:bool, element #3=w646:bool)  [unwired: 3 in]
                  n649 = Index Array(array=w739) -> (element #1=w738:dbl, element #2=w737:dbl, element #3=w736:dbl, element #4=w735:dbl, element #5=w734:dbl, element #6=w733:dbl, element #7=w732:dbl, element #8=w731:dbl, element #9=w730:dbl)  [unwired: 9 in]
                  n650 = Unbundle By Name(w664) -> ("Reheat Parameters"=w663:T16)
                  n651 = Bundle By Name(cluster=w663, "Filament I (A)"=w662, "Reheat time (s)"=w661, "Emission (uA)"=w660, "Calculate V/I slope"=w659, "Pre-calc delay (min)"=w658, "Disable Reheat Retries"=w657, "Restore Voltages"=w656) -> (w647:T16)
                  n652 = local read "Read output"() -> (w832:T1)
                  n653 = Unbundle By Name(w832) -> ("Alert Settings"=w833:T29)
                  n654 = Bundle By Name(cluster=w833, "3D imaging paused alarm"=w715, "FIB emission limit warning"=w714, "Low limit"=w712, "High limit"=w711, "Specimen @ SEM alarm"=w603, "FIB CL current alarm"=w706, "Beam Dump 1 alarm"=w563, "Milling Z voltage alarm"=w562, "EHT off alarm"=w561, "Detector over scale warning"=w560, "Image clipping alarm"=w542, "Warning limit (um)"=w531, "Stop limit (um)"=w530, "Temperature alarm"=w529, "Pause 3D-ING"=w528, "Low limit (F)"=w704, "High limit (F)"=w703, "Temp limit auto"=w823, "Delta (F)"=w693, "Gradient limit (F/min)"=w692, "SW error warning"=w691, "Focus index warning"=w690, "Focus index low limit"=w628, "Focus index stop limit"=w627, "Run Auto Stig"=w687, "FI low limit auto"=w686, "FI stop limit auto"=w626) -> (w831:T29)
                  n655 = Bundle By Name(cluster=w1053, "SEM Scan Parameters"=w1052, "Detector Information"=w1020, "SEM Options"=w1017, "Focus Index Options"=w544, "Image fit to"=w723, "File Information"=w1005, "Low mag SEM"=w944, "Mid Mag SEM"=w745, "FIB-SEM Angle"=w521, "Milling para"=w943, "FI Detector"=w930, "Auto Optimzation"=w929, "Images per Auto Optimization"=w738, "AF Range (nm)"=w737, "AF Steps"=w736, "AS Range (%)"=w735, "AS Steps"=w734, "AA Range (%)"=w733, "AA Steps"=w732, "X shift (nm/frame)"=w731, "Y shift (nm/frame)"=w730, "FIB Y zoom pixel (nm)"=w914, "Mail server"=w908, "Email Alert Recipients"=w905, "Alert Settings"=w831, "Reheat Parameters"=w647, "Start FIB HV DataLog"=w646, "Interval (s)"=w645) -> (w481:T1)
                }
              }
            }
          }
          "Read output" <- w3
        }
        frame True {
          w1588 = "\"" ("string")
          n656 = Unbundle By Name("Write input") -> ("SEM Scan Parameters"=w1450:T20, "Detector Information"=w1608:T8, "SEM Options"=w1607:T9)
          n657 = Unbundle By Name("Write input") -> ("Focus Index Options.Keep aspect ratio"=w1568:bool, "Focus Index Options.Show Focus Index"=w1563:bool, "Focus Index Options.Focus Index primary grid center"=w1564:bool, "Focus Index Options.X Grids"=w1429:u8[][], "Focus Index Options.Y Grids"=w1428:u8[][], "Focus Index Options.Primary X index"=w1427:u8[][], "Focus Index Options.Primary Y index"=w1426:u8[][], "Image fit to"=w1430:u8)
          n658 = Unbundle By Name("Write input") -> ("File Information"=w1572:T10, "Low mag SEM"=w1573:T11, "Mid Mag SEM"=w1528:T12, "FIB-SEM Angle"=w1574:dbl, "Milling para"=w1575:T28)
          n659 = Unbundle By Name("Write input") -> ("FIB Y zoom pixel (nm)"=w1587:dbl, "Mail server"=w1585:string, "Email Alert Recipients"=w1578:string[])
          n660 = Unbundle By Name("Write input") -> ("Reheat Parameters"=w1513:T16)
          n661 = Unbundle By Name("Write input") -> ("Start FIB HV DataLog"=w1502:bool, "Interval (s)"=w1501:u16)
          n662 = Unbundle By Name("Write input") -> ("Alert Settings"=w1550:T29)
          n663 = Unbundle By Name(w1550) -> ("3D imaging paused alarm"=w1489:bool, "FIB emission limit warning"=w1488:bool, "Low limit"=w1548:sgl, "High limit"=w1547:sgl, "Specimen @ SEM alarm"=w1462:bool, "FIB CL current alarm"=w1492:bool, "Beam Dump 1 alarm"=w1491:bool, "Milling Z voltage alarm"=w1432:bool, "EHT off alarm"=w1431:bool, "Detector over scale warning"=w1423:bool, "Image clipping alarm"=w1422:bool, "Warning limit (um)"=w1419:sgl, "Stop limit (um)"=w1418:sgl, "Temperature alarm"=w1416:bool, "Pause 3D-ING"=w1415:bool, "Low limit (F)"=w1545:sgl, "High limit (F)"=w1544:sgl, "Temp limit auto"=w1537:bool, "Delta (F)"=w1539:sgl, "Gradient limit (F/min)"=w1538:sgl, "SW error warning"=w1543:bool, "Focus index warning"=w1542:bool, "Focus index low limit"=w1541:sgl, "Focus index stop limit"=w1485:sgl, "Run Auto Stig"=w1482:bool, "FI low limit auto"=w1481:bool, "FI stop limit auto"=w1480:bool)
          n664 = Unbundle By Name(w1513) -> ("Filament I (A)"=w1512:sgl, "Reheat time (s)"=w1510:sgl, "Emission (uA)"=w1509:sgl, "Calculate V/I slope"=w1508:bool, "Pre-calc delay (min)"=w1507:sgl, "Disable Reheat Retries"=w1506:bool, "Restore Voltages"=w1505:bool)
          n665 = Unbundle By Name(w1450) -> ("X size (um)"=w1459:sgl, "Y size (um)"=w1458:sgl, "X center (um)"=w1457:dbl, "Y center (um)"=w1456:dbl, "X size (V)"=w1455:dbl, "Frames"=w1454:u8, "X tiles"=w1453:u8, "Y tiles"=w1452:u8, "Overlap (um)"=w1451:sgl)
          n666 = Unbundle By Name(w1450) -> ("dX (um)"=w1441:sgl[], "dY (um)"=w1434:sgl[])
          n667 = Unbundle By Name(w1450) -> ("Scan rate (Hz)"=w1478:u32, "Pixel size (nm)"=w1477:sgl, "Frame line rampdown ratio"=w1476:sgl, "Oversampling"=w1475:u32, "X stig"=w1469:sgl[][], "Y stig"=w1468:sgl[][], "X aln"=w1467:sgl[][], "Y aln"=w1466:sgl[][], "WD (mm)"=w1465:sgl[][], "X size auto"=w1474:bool, "Oversampling auto"=w1473:bool, "Interlaced"=w1472:bool)
          n668 = Unbundle By Name(w1608) -> ("Brightness A"=w1612:dbl, "Contrast A"=w1613:dbl, "Detector B name"=w1618:string, "Brightness B"=w1615:dbl, "Contrast B"=w1616:dbl)
          n669 = Unbundle By Name(w1607) -> ("GetInfo"=w1623:bool, "Set Det A para"=w1624:bool, "Set WD"=w1625:bool, "Set Mag"=w1626:bool, "Set stig"=w1627:bool, "Set aln"=w1516:bool, "Display"=w1628:bool, "Save"=w1629:bool, "8-bit"=w1461:bool, "Detector A"=w1630:bool, "Detector B"=w1631:bool, "Detector C"=w1632:bool, "Detector D"=w1633:bool, "Inverse A"=w1634:bool, "Inverse B"=w1635:bool, "Inverse C"=w1636:bool, "Inverse D"=w1637:bool, "Inverse PNG"=w1638:bool, "Freeze"=w1639:bool, "PNG only"=w1640:bool, "Upload"=w1576:bool, "Delete after upload"=w1560:bool)
          n670 = Unbundle By Name(w1572) -> ("File path"=w1606:path, "Notes"=w1589:string, "Sample ID"=w1559:string)
          n671 = Unbundle By Name(w1573) -> ("Low mag scan"=w1669:bool, "Prior to main scan"=w1668:bool, "Low mag interval"=w1670:u32, "Low mag scan FOV (micron)"=w1671:dbl, "Low mag scan rate (Hz)"=w1672:u32, "Show HM box"=w1673:bool)
          n672 = Unbundle By Name(w1528) -> ("Mid mag scan"=w1532:bool, "Prior to main scan"=w1533:bool, "Mid mag interval"=w1531:u32, "X size (um)"=w1530:sgl, "Y size (um)"=w1529:sgl, "X center (um)"=w1526:dbl, "Y center (um)"=w1525:dbl, "Mid mag scan rate (Hz)"=w1524:u32, "Pixel size (nm)"=w1523:dbl, "Show MM box"=w1527:bool)
          n673 = Unbundle By Name(w1575) -> ("X resolution"=w1649:u32, "Z resolution"=w1650:u32, "X offset (um)"=w1651:sgl, "Z offset (um)"=w1652:sgl, "X center (um)"=w1653:sgl, "Z center (um)"=w1654:sgl, "X size (um)"=w1655:sgl, "Z size (um)"=w1656:sgl, "UL-Ang"=w1562:sgl, "UR-Ang"=w1561:sgl, "Line milling time (s)"=w1657:sgl, "Z-step (nm)"=w1413:dbl, "Lines auto pause"=w1410:u16, "Auto pause"=w1660:bool, "Mill from Bottom"=w1661:bool, "FIB FOV (um)"=w1662:sgl, "Auto Profile"=w1663:bool, "FIB PID on"=w1558:bool, "FIB PID measured"=w1494:u8, "FIB PID target"=w1556:sgl, "FIB PID target slope"=w1518:sgl, "FIB PID P"=w1555:sgl, "FIB PID I"=w1554:sgl, "FIB PID D"=w1553:sgl, "Emission (uA)"=w1409:dbl, "Suppressor (V)"=w1408:sgl, "Auto reheat"=w1407:bool)
          n674 = Unbundle By Name("Write input") -> ("FI Detector"=w1604:u16, "Auto Optimzation"=w1605:bool, "Images per Auto Optimization"=w1601:u16, "AF Range (nm)"=w1600:sgl, "AF Steps"=w1599:u8, "AS Range (%)"=w1598:sgl, "AS Steps"=w1597:u8, "AA Range (%)"=w1515:sgl, "AA Steps"=w1514:u8, "X shift (nm/frame)"=w1596:dbl, "Y shift (nm/frame)"=w1595:dbl)
          n675 = Array To Spreadsheet String(delimiter (Tab)="," ("string"), array=w1578, 3:"%s" ("format string")) -> (spreadsheet string=w1583:string)
          n676 = Search and Replace String(input string=w1583, search string="\r\n", replace string="") -> (result string=w1577:string)  [unwired: 5 in, 3 out]
          n677 = Build Array(w1489, w1488) -> (w1487:bool[])
          n678 = Build Array(w1462, w1492, w1491, w1432, w1431, w1423, w1422) -> (w1493:bool[])
          n679 = Build Array(w1416, w1415) -> (w1421:bool[])
          n680 = Build Array(w1539, w1538) -> (w1540:sgl[])
          n681 = Build Array(w1482, w1481, w1480) -> (w1483:bool[])
          n682 = Build Array(w1512, w1510, w1509) -> (w1511:sgl[])
          n683 = Build Array(w1506, w1505, w1502) -> (w1504:bool[])
          n684 = Concatenate Strings(w1588, w1589, w1588) -> (w1590:string)
          n685 = Format Into String(w1430) -> (resulting string=w1571:string)  [unwired: 3 in, 1 out]
          n686 = Build Array(w1429, w1428, w1427, w1426) -> (w1425:u8[][][])
          n687 = for {
            tunnel: w1487 -> [w1702] mode=indexing
            tunnel: [w1703] -> w1486 mode=indexing
            n688 = Format Into String(w1702) -> (resulting string=w1703:string)  [unwired: 3 in, 1 out]
          }
          n689 = Build Array(w1548, w1547) -> (w1549:sgl[])
          n690 = for {
            tunnel: w1493 -> [w1704] mode=indexing
            tunnel: [w1705] -> w1490 mode=indexing
            n691 = Format Into String(w1704) -> (resulting string=w1705:string)  [unwired: 3 in, 1 out]
          }
          n692 = Build Array(w1419, w1418) -> (w1420:sgl[])
          n693 = for {
            tunnel: w1421 -> [w1676] mode=indexing
            tunnel: [w1677] -> w1414 mode=indexing
            n694 = Format Into String(w1676) -> (resulting string=w1677:string)  [unwired: 3 in, 1 out]
          }
          n695 = Build Array(w1545, w1544) -> (w1570:sgl[])
          n696 = for {
            tunnel: w1540 -> [w1865] mode=indexing
            tunnel: [w1866] -> w1535 mode=indexing
            n697 = Format Into String(w1865) -> (resulting string=w1866:string)  [unwired: 3 in, 1 out]
          }
          n698 = for {
            tunnel: w1483 -> [w1700] mode=indexing
            tunnel: [w1701] -> w1479 mode=indexing
            n699 = Format Into String(w1700) -> (resulting string=w1701:string)  [unwired: 3 in, 1 out]
          }
          n700 = for {
            tunnel: w1511 -> [w1708] mode=indexing
            tunnel: [w1709] -> w1500 mode=indexing
            n701 = Format Into String(w1708) -> (resulting string=w1709:string)  [unwired: 3 in, 1 out]
          }
          n702 = for {
            tunnel: w1504 -> [w1706] mode=indexing
            tunnel: [w1707] -> w1497 mode=indexing
            n703 = Format Into String(w1706) -> (resulting string=w1707:string)  [unwired: 3 in, 1 out]
          }
          n704 = Path To String(path=w1606) -> (string=w1648:string)
          n705 = for {
            tunnel: w1425 -> [w1678] mode=indexing
            tunnel: [w1679] -> w1424 mode=indexing
            n706 = Array Size(array=w1678) -> (size(s)=w1682:i32[])
            n707 = Multiply Array Elements(1:w1682) -> (0:w1683:i32)
            n708 = Reshape Array(w1678, w1683) -> (w1684:u8[])
            n709 = Array To Spreadsheet String(delimiter (Tab)=",", array=w1684, 3:"%#g" ("format string")) -> (spreadsheet string=w1680:string)
            n710 = Match Pattern(string=w1680, regular expression="\r\n") -> (before substring=w1679:string)  [unwired: 1 in, 3 out]
          }
          n711 = Build Array(w1612, w1613) -> (w1611:dbl[])
          n712 = Build Array(w1615, w1616) -> (w1614:dbl[])
          n713 = Format Into String(w1669) -> (resulting string=w1643:string)  [unwired: 3 in, 1 out]
          n714 = Format Into String(w1668) -> (resulting string=w1644:string)  [unwired: 3 in, 1 out]
          n715 = Build Array(w1670, w1671, w1672) -> (w1642:dbl[])
          n716 = Format Into String(w1673) -> (resulting string=w1646:string)  [unwired: 3 in, 1 out]
          n717 = Format Into String(w1532) -> (resulting string=w1522:string)  [unwired: 3 in, 1 out]
          n718 = Format Into String(w1533) -> (resulting string=w1521:string)  [unwired: 3 in, 1 out]
          n719 = Build Array(w1531, w1530, w1529, w1526, w1525, w1524, w1523) -> (w1534:dbl[])
          n720 = Format Into String(w1527) -> (resulting string=w1519:string)  [unwired: 3 in, 1 out]
          n721 = Build Array(w1574, w1649, w1650, w1651, w1652, w1653, w1654, w1655, w1656, w1562, w1561, w1657, w1413) -> (w1658:dbl[])
          n722 = Build Array(w1494, w1556, w1518, w1555, w1554, w1553, w1409, w1408) -> (w1552:dbl[])
          n723 = Build Array(w1459, w1458, w1457, w1456, w1455, w1454, w1453, w1452, w1451) -> (w1460:dbl[])
          n724 = Build Array(w1478, w1477, w1476, w1475) -> (w1620:sgl[])
          n725 = Build Array(w1469, w1468, w1467, w1466, w1465) -> (w1464:sgl[][][])
          n726 = Build Array(w1474, w1473, w1472) -> (w1471:bool[])
          n727 = Build Array(w1623, w1624, w1625, w1626, w1627, w1516, w1628, w1629, w1461, w1630, w1631, w1632, w1633, w1634, w1635, w1636, w1637, w1638, w1639, w1640, w1576, w1560, w1568, w1563, w1564) -> (w1622:bool[])
          n728 = Build Array(w1601, w1600, w1599, w1598, w1597, w1515, w1514, w1596, w1595) -> (w1594:dbl[])
          n729 = Format Into String(w1410) -> (resulting string=w1411:string)  [unwired: 3 in, 1 out]
          n730 = Format Into String(w1661) -> (resulting string=w1664:string)  [unwired: 3 in, 1 out]
          n731 = Format Into String(w1663) -> (resulting string=w1666:string)  [unwired: 3 in, 1 out]
          n732 = Format Into String(w1407) -> (resulting string=w1406:string)  [unwired: 3 in, 1 out]
          n733 = Format Into String(w1604) -> (resulting string=w1603:string)  [unwired: 3 in, 1 out]
          n734 = Format Into String(w1587) -> (resulting string=w1586:string)  [unwired: 3 in, 1 out]
          n735 = for {
            tunnel: w1549 -> [w1867] mode=indexing
            tunnel: [w1868] -> w1546 mode=indexing
            n736 = Format Into String(w1867) -> (resulting string=w1868:string)  [unwired: 3 in, 1 out]
          }
          n737 = for {
            tunnel: w1420 -> [w1674] mode=indexing
            tunnel: [w1675] -> w1417 mode=indexing
            n738 = Format Into String(w1674) -> (resulting string=w1675:string)  [unwired: 3 in, 1 out]
          }
          n739 = for {
            tunnel: w1570 -> [w1871] mode=indexing
            tunnel: [w1872] -> w1569 mode=indexing
            n740 = Format Into String(w1871) -> (resulting string=w1872:string)  [unwired: 3 in, 1 out]
          }
          n741 = Format Into String(w1543) -> (resulting string=w1567:string)  [unwired: 3 in, 1 out]
          n742 = for {
            tunnel: w1611 -> [w1889] mode=indexing
            tunnel: [w1890] -> w1617 mode=indexing
            n743 = Format Into String(w1889) -> (resulting string=w1890:string)  [unwired: 3 in, 1 out]
          }
          n744 = for {
            tunnel: w1614 -> [w1887] mode=indexing
            tunnel: [w1888] -> w1619 mode=indexing
            n745 = Format Into String(w1887) -> (resulting string=w1888:string)  [unwired: 3 in, 1 out]
          }
          n746 = for {
            tunnel: w1642 -> [w1881] mode=indexing
            tunnel: [w1882] -> w1645 mode=indexing
            n747 = Format Into String(w1881) -> (resulting string=w1882:string)  [unwired: 3 in, 1 out]
          }
          n748 = for {
            tunnel: w1534 -> [w1863] mode=indexing
            tunnel: [w1864] -> w1520 mode=indexing
            n749 = Format Into String(w1863) -> (resulting string=w1864:string)  [unwired: 3 in, 1 out]
          }
          n750 = for {
            tunnel: w1658 -> [w1879] mode=indexing
            tunnel: [w1880] -> w1659 mode=indexing
            n751 = Format Into String(w1879) -> (resulting string=w1880:string)  [unwired: 3 in, 1 out]
          }
          n752 = for {
            tunnel: w1552 -> [w1869] mode=indexing
            tunnel: [w1870] -> w1551 mode=indexing
            n753 = Format Into String(w1869) -> (resulting string=w1870:string)  [unwired: 3 in, 1 out]
          }
          n754 = for {
            tunnel: w1594 -> [w1873] mode=indexing
            tunnel: [w1874] -> w1593 mode=indexing
            n755 = Format Into String(w1873) -> (resulting string=w1874:string)  [unwired: 3 in, 1 out]
          }
          n756 = Format Into String(w1508) -> (resulting string=w1499:string)  [unwired: 3 in, 1 out]
          n757 = Format Into String(w1501) -> (resulting string=w1496:string)  [unwired: 3 in, 1 out]
          n758 = for {
            tunnel: w1460 -> [w1687] mode=indexing
            tunnel: [w1688] -> w1448 mode=indexing
            n759 = Format Into String(w1687) -> (resulting string=w1688:string)  [unwired: 3 in, 1 out]
          }
          n760 = for {
            tunnel: w1620 -> [w1885] mode=indexing
            tunnel: [w1886] -> w1621 mode=indexing
            n761 = Format Into String(w1885) -> (resulting string=w1886:string)  [unwired: 3 in, 1 out]
          }
          n762 = for {
            tunnel: w1464 -> [w1689] mode=indexing
            tunnel: [w1690] -> w1463 mode=indexing
            n763 = Array Size(array=w1689) -> (size(s)=w1693:i32[])
            n764 = Multiply Array Elements(1:w1693) -> (0:w1694:i32)
            n765 = Reshape Array(w1689, w1694) -> (w1695:sgl[])
            n766 = Array To Spreadsheet String(delimiter (Tab)=",", array=w1695, 3:"%#g" ("format string")) -> (spreadsheet string=w1691:string)
            n767 = Match Pattern(string=w1691, regular expression="\r\n") -> (before substring=w1690:string)  [unwired: 1 in, 3 out]
          }
          n768 = for {
            tunnel: w1471 -> [w1698] mode=indexing
            tunnel: [w1699] -> w1470 mode=indexing
            n769 = Format Into String(w1698) -> (resulting string=w1699:string)  [unwired: 3 in, 1 out]
          }
          n770 = for {
            tunnel: w1622 -> [w1883] mode=indexing
            tunnel: [w1884] -> w1641 mode=indexing
            n771 = Format Into String(w1883) -> (resulting string=w1884:string)  [unwired: 3 in, 1 out]
          }
          n772 = Format Into String(w1660) -> (resulting string=w1412:string)  [unwired: 3 in, 1 out]
          n773 = Format Into String(w1662) -> (resulting string=w1665:string)  [unwired: 3 in, 1 out]
          n774 = Format Into String(w1558) -> (resulting string=w1557:string)  [unwired: 3 in, 1 out]
          n775 = Format Into String(w1605) -> (resulting string=w1602:string)  [unwired: 3 in, 1 out]
          n776 = Array Size(array=w1441) -> (size(s)=w1442:i32)
          n777 = Array Size(array=w1434) -> (size(s)=w1440:i32)
          n778 = Format Into String(w1542) -> (resulting string=w1566:string)  [unwired: 3 in, 1 out]
          n779 = Format Into String(w1507) -> (resulting string=w1498:string)  [unwired: 3 in, 1 out]
          n780 = Build Array(w1411, w1412, w1664, w1665, w1666, w1557) -> (w1667:string[])
          n781 = Format Into String(w1541) -> (resulting string=w1565:string)  [unwired: 3 in, 1 out]
          n782 = Format Into String(w1537) -> (resulting string=w1536:string)  [unwired: 3 in, 1 out]
          n783 = Reshape Array(w1441, w1442) -> (w1445:sgl[])
          n784 = Reshape Array(w1434, w1440) -> (w1437:sgl[])
          n785 = Format Into String(w1485) -> (resulting string=w1484:string)  [unwired: 3 in, 1 out]
          n786 = Array To Spreadsheet String(delimiter (Tab)=",", array=w1445, 3:"%#g" ("format string")) -> (spreadsheet string=w1443:string)
          n787 = Array To Spreadsheet String(delimiter (Tab)=",", array=w1437, 3:"%#g" ("format string")) -> (spreadsheet string=w1439:string)
          n788 = Match Pattern(string=w1443, regular expression="\r\n") -> (before substring=w1449:string)  [unwired: 1 in, 3 out]
          n789 = Match Pattern(string=w1439, regular expression="\r\n") -> (before substring=w1433:string)  [unwired: 1 in, 3 out]
          n790 = Build Array (concatenate)(w1648, w1590, w1559, w1643, w1644, w1645, w1646, w1522, w1521, w1520, w1519, w1659, w1667, w1551) -> (w1647:string[])
          n791 = Build Array (concatenate)(w1406, w1603, w1602, w1593, w1586) -> (w1592:string[])
          n792 = Build Array (concatenate)(w1500, w1499, w1498, w1497, w1496) -> (w1495:string[])
          n793 = Build Array (concatenate)(w1585, w1577, w1486, w1546, w1490, w1417, w1414, w1569, w1536, w1535, w1567, w1566, w1565, w1484, w1479) -> (w1584:string[])
          n794 = Build Array (concatenate)(w1448, w1449, w1433, w1621, w1463, w1470, w1617, w1618, w1619, w1641, w1424, w1571, w1647, w1592, w1584, w1495) -> (w1609:string[])
          n795 = local read "Recipe items"() -> (w1591:string[])
          n796 = for {
            tunnel: w1591 -> [w1876] mode=indexing
            tunnel: [w1877] -> w1610 mode=indexing
            tunnel: w1609 -> [w1875] mode=indexing
            n797 = Concatenate Strings(w1876, "," ("string"), w1875) -> (w1877:string)
          }
          n798 = case shown="True" "Use csv file" {
            tunnel: w1610 -> [w1710 w1720]
            frame False {
              "Recipe csv array" <- w1710
            }
            frame True {
              n799 = Strip Path(path="Recipe path") -> (name=w1713:string)  [unwired: 1 out]
              n800 = xnode "Match Regular Expression"("input string"=w1713, "regular expression"=".csv") -> ("offset past match"=w1715:i32)  [unwired: 4 in, 4 out]
              n801 = Equal?(x=w1715, y=-1) -> (x = y?=w1712:bool)
              n802 = case shown="True" w1712 {
                tunnel: [w1834 w1846] -> w1719
                tunnel: [w1836 w1845] -> w1718
                tunnel: [w1835 w1838] -> w1717
                tunnel: "Recipe path" -> [w1832 w1837]
                frame False {
                  n803 = Open/Create/Replace File(file path (use dialog)=w1832, operation (0:open)=T6."replace or create with confirmation") -> (refnum out=w1836:refnum<file>, cancelled=w1835:bool, error out=w1834:errorcluster)  [unwired: 1 in, 3 out]
                }
                frame True {
                  n804 = Equal?(x="", y="Info") -> (x = y?=w1841:bool)
                  n805 = Get Date/Time In Seconds() -> (seconds since 1Jan1904=w1849:timestamp)
                  n806 = case shown="True" w1841 {
                    tunnel: [" " ("string") ""] -> w1842
                    frame False {
                    }
                    frame True {
                    }
                  }
                  n807 = Format Date/Time String(time format string (%c)="%y-%m-%d", seconds (now)=w1849) -> (date/time string=w1850:string)  [unwired: 1 out]
                  n808 = Concatenate Strings("FIB-SEM recipe " ("string"), w1850, w1842, "Info", ".csv" ("string")) -> (w1852:string)
                  n809 = Build Path(base path=w1837, name or relative path=w1852) -> (appended path=w1844:path)
                  n810 = Open/Create/Replace File(file path (use dialog)=w1844, operation (0:open)=T6."replace or create with confirmation") -> (refnum out=w1845:refnum<file>, cancelled=w1838:bool, error out=w1846:errorcluster)  [unwired: 1 in, 3 out]
                }
              }
              n811 = case shown="False" w1717 {
                tunnel: w1720 -> [w1862 _]
                tunnel: w1719 -> [w1858 _]
                tunnel: w1718 -> [w1857 _]
                frame False {
                  n812 = Set File Position(refnum=w1857, from (0:start)=enum16{"start", "end", "current"}."end", error in=w1858) -> (refnum out=w1859:refnum<file>, error out=w1856:errorcluster)  [unwired: 1 out]
                  n813 = Write to Text File(file (use dialog)=w1859, text=w1862, error in=w1856) -> (refnum out=w1860:refnum<file>, error out=w1861:errorcluster)  [unwired: 2 out]
                  n814 = Close File(refnum=w1860, error in=w1861) -> ()  [unwired: 2 out]
                }
                frame True {
                }
              }
            }
          }
        }
      }
    }
  }
